vi "CRYPost Processing Editor.vi"() -> ()   [LabVIEW 2013]
uses:
  <vilib>/Utility/miscctls.llb/LVBoundsTypeDef.ctl
  Typedef Control/CRYPost Processing Cluster.ctl
  Typedef Control/CRYUser Equation Cluster.ctl
  CRYProject/CRYProject Editor Global.vi
  SubVI/CRYPost Processing Global.vi
  Program/CRYRef nums global.vi
  CRYWindow/SubVI/CRYMain Sub Window Global.vi
  CRYMainGlobal.vi
  CRYStepSetup/CRYStepSetup Global.vi
panel:
  out "Result Data":string[](array[string])
  in  "A log/lin":u16
  in  "tmp Val_B":dbl min=1.0 format="%#_6p"
  in  "tmp Val_A":dbl min=1.0 format="%#_6p"
  out "Show Calcu":bool
  out "Post Processing Bk":T1 {"user equation cluster"."Results axis" items=["x", "y", "z"]; "user equation cluster"."Input axis" items=["x", "y", "z"]; "user equation cluster"."Custom unit results array"."dB ref" format="%.2f"; "user equation cluster"."Custom unit input array"."dB ref" format="%.2f"; "Constant" format="%#.5p"; "Unary Operator" format="%10.0f"; "Custom unit info"."dB ref" format="%.2f"; "Sampling Rate" format="%#.2p"}
  in  "SW_EdtObj":u8
  in  "CurLibChange":bool caption="Add Lib"
  out "Old Exponent":sgl
  out "Loading_F":bool
  in  "Add Lib":bool
  in  "AddStep":bool
  in  "StateOut":bool
  in  "Board Tab":enum32{"Page 1"}(tab)
  in  "Cancel":bool caption="Apply"
  in  "OK":bool caption="Apply"
  in  "Main Tab":enum32{"Setting", "Help"}(tab)
  in  "Smoothing_Res":bool caption="平滑"
  in  "Freq Sampling Rate":dbl caption="频率" format="%#.2p"
  in  "Freq Sampling Mode":u16(slide) caption="Ref Freq Mode"
  out "Freq Sampling":bool caption="频率"
  in  "Operation1 Tab":enum32{"Page 1"}(tab)
  in  "binary operation":u16(ring) items=[" +", " --", " x", "÷"]
  out "Operation_1":bool caption="运算"
  in  "Work in":u16(slide) caption="运算模式"
  in  "Result_axis Tab":enum32{"Page 1"}(tab)
  out "Resut x_axis":bool caption="结果X轴"
  in  "Axis Mode":u16(slide)
  in  "Desired Tab":enum32{"Page 1"}(tab)
  out "Desired Result":bool caption="结果"
  in  "Use default":bool caption="使用默认值"
  in  "Name":string caption="名称"
  in  "x_1":bool caption="x"
  in  "y_1":bool caption="y"
  in  "z_1":bool caption="z"
  out "Unit String":string caption="单位"
  in  "Unit_Cont":bool
  out "Show data":string
  in  "OpA2 Tab":enum32{"Page 1"}(tab)
  in  "Op_A2":u16(ring) items=["Stimulus", "时间包络 [Direct Out 1]", "Record Wave [Direct In 1]", "2-时间包络 [Direct Out 1]", "调用文件曲线1", "Stimulus - P", "2-Stimulus - P", "3-Stimulus - P"]
  out "Operand_A2":bool caption="操作数 A"
  in  "Sear_range Tab":enum32{"Page 1"}(tab)
  in  "Edit Range":bool
  in  "All":bool caption="所有"
  in  "Search List":i32(listbox) caption="Hz"
  out "Search Range":bool caption="搜索范围"
  in  "Width Tab":enum32{"Page 1"}(tab)
  in  "Octav Mode":u16(ring) items=["1/1 Octave", "1/3 Octave", "1/6 Octave", "1/12 Octave", "1/24 Octave", "User Defined log", "User Defined lin"]
  out "Width":bool caption="宽度"
  out "Weighting":bool caption="加权"
  in  "Weight Mode":u16(ring) items=["None", "Hanning"]
  in  "Hz_Oct_1":dbl=1.0 caption="1/n 倍频程" min=1.0 step=1.0 format="%#.2p"
  in  "Sear_type Tab":enum32{"Page 1"}(tab)
  in  "Search Mode":u16(slide)
  out "Search Type":bool caption="搜索类型"
  in  "Equation Tab":enum32{"Page 1"}(tab)
  in  "Clear All Fields":bool
  out "#Desired Results":u32 caption="结果个数"
  out "#Operands":u32 caption="操作数个数"
  in  "z_2":bool caption="z"
  in  "y_2":bool caption="y"
  in  "x_2":bool caption="x"
  out "Equation":bool caption="公式 (e.g. x=a0+a1;)"
  in  "Equ_List":string
  out "Show xy":string
  in  "Org_res Tab":enum32{"Page 1"}(tab)
  out "Original Res":string
  out "Steps":i32 caption="步骤"
  out "Org_Res":bool caption="原始分辨率"
  in  "New Resolution":u16(ring) items=["1/1 Octave", "1/3 Octave", "1/6 Octave", "1/12 Octave", "1/24 Octave"]
  out "New_Res":bool caption="新的分辨率"
  in  "Frequencies":u16(slide) caption="频率"
  in  "Hz_Oct_2":u32=1 caption="1/n 倍频程" min=1 step=1
  in  "Direct Tab":enum32{"Page 1"}(tab)
  in  "Total Rotation":i32 caption="总旋转"
  in  "Inc(deg.)":i32 caption="增量(deg.)"
  in  "Ref_Curve":u16(ring) items=["unity cal-in corr-in", "CRY33x Mic 1 corr-in", "CRY33x Mic 2 corr-in", "CRY33x Mic 3 corr-in", "CRY33x Mic 4 corr-in", "USB In L corr-in", "USB In R corr-in", "unity cal-out corr-out", "unity cal-out eq-out", "CRY602 Mouth 1 corr-out", "CRY602 Mouth 1 eq-out", "CRY602 Mouth 2 corr-out", "CRY602 Mouth 2 eq-out", "USB Out R corr-out", "USB Out R eq-out", "频率响应 [Direct Out 1]", "谐波 2 [Direct Out 1]", "谐波 3 [Direct Out 1]", "谐波 4 [Direct Out 1]", "谐波 5 [Direct Out 1]", "总谐波失真 [Direct Out 1]", "上下限 上限", "上下限 下限", "2-频率响应 [Direct Out 1]", "2-谐波 2 [Direct Out 1]", "2-谐波 3 [Direct Out 1]", "2-谐波 4 [Direct Out 1]", "2-谐波 5 [Direct Out 1]", "2-总谐波失真 [Direct Out 1]", "调用文件曲线1"]
  in  "Auto Inc":bool caption="自动增量"
  in  "Curve List":i32[](listbox) caption="Hz"
  in  "Direct_weight":bool caption="加权"
  in  "Weight Curve_2":u16(ring) items=["unity cal-in corr-in", "CRY33x Mic 1 corr-in", "CRY33x Mic 2 corr-in", "CRY33x Mic 3 corr-in", "CRY33x Mic 4 corr-in", "USB In L corr-in", "USB In R corr-in", "unity cal-out corr-out", "unity cal-out eq-out", "CRY602 Mouth 1 corr-out", "CRY602 Mouth 1 eq-out", "CRY602 Mouth 2 corr-out", "CRY602 Mouth 2 eq-out", "USB Out R corr-out", "USB Out R eq-out", "频率响应 [Direct Out 1]", "谐波 2 [Direct Out 1]", "谐波 3 [Direct Out 1]", "谐波 4 [Direct Out 1]", "谐波 5 [Direct Out 1]", "总谐波失真 [Direct Out 1]", "上下限 上限", "上下限 下限", "2-频率响应 [Direct Out 1]", "2-谐波 2 [Direct Out 1]", "2-谐波 3 [Direct Out 1]", "2-谐波 4 [Direct Out 1]", "2-谐波 5 [Direct Out 1]", "2-总谐波失真 [Direct Out 1]", "调用文件曲线1"]
  out "Reference Curve":bool caption="参考曲线"
  out "Curve Group":bool caption="曲线组"
  out "Weight Function":bool caption="加权函数"
  out "Increment":bool caption="增量"
  in  "Org_samp Tab":enum32{"Page 1"}(tab)
  in  "New  Samp Val":dbl min=1.0 format="%#_6p"
  out "Origi Samp Val":dbl caption="Original Sampling Rate" format="%#.2p"
  out "Origi SampRate":bool caption="原始采样率"
  out "New Samp Rate":bool caption="新采样率"
  in  "Freq Tab":enum32{"Page 1"}(tab)
  in  "Ref Frequency":dbl caption="参考频率" format="%#.2p"
  in  "Ref Wave":u16(ring) caption="参考波形" items=["Stimulus", "时间包络 [Direct Out 1]", "Record Wave [Direct In 1]", "2-时间包络 [Direct Out 1]", "调用文件曲线1", "Stimulus - P", "2-Stimulus - P", "3-Stimulus - P"]
  in  "Ref Freq Mode":u16(slide)
  out "Ref Freq":bool caption="参考频率"
  in  "Smooth Tab":enum32{"Page 1"}(tab)
  in  "Smoo Width":i32 min=1
  out "Smoothing":bool caption="平滑宽度(Hz)"
  in  "Window Tab":enum32{"Page 1"}(tab)
  out "Window":bool caption="窗口"
  in  "Win Mode":u16(ring) items=["None", "Cosine Taper", "Exponential"]
  in  "Sampling Tab":enum32{"Page 1"}(tab)
  in  "Samp Rate":dbl format="%#.2p"
  out "Sampling":bool caption="采样率"
  in  "Operation2 Tab":enum32{"Page 1"}(tab)
  out "Operation_2":bool caption="运算"
  in  "Statistical Operator":u16(ring) items=["平均值", "功率总和", "最大值", "最小值", "谐振估算", "反谐振估算", "IEEE TOLR", "IEEE ROLR", "IEEE SOLR", "ITU-T SLR", "ITU-T RLR", "ITU-T RLR w/ Leak", "ITU-T STMR", "Attack Time", "Release Time", "Zwicker Loudness"]
  in  "Unary Operator":u16(ring) items=["相反数", "倒数", "绝对值", "平方", "平方根", "指数", "自然对数", "Unwrap Phase", "Group Delay", "FFT", "Inverse FFT"]
  in  "Param Tab":enum32{"Page 1"}(tab)
  out "Parameter":bool caption="参数"
  in  "dB":sgl format="%#.4p"
  in  "%":sgl format="%#.4p"
  in  "Weight_fun Tab":enum32{"Page 1"}(tab)
  in  "Exponent":sgl caption="指数" format="%#.2p"
  out "Weighting_Func":bool caption="加权函数"
  in  "Use Default Exp":bool caption="用户默认值"
  in  "Weight Curve_1":u16(ring) caption="加权曲线" items=["unity cal-in corr-in", "CRY33x Mic 1 corr-in", "CRY33x Mic 2 corr-in", "CRY33x Mic 3 corr-in", "CRY33x Mic 4 corr-in", "USB In L corr-in", "USB In R corr-in", "unity cal-out corr-out", "unity cal-out eq-out", "CRY602 Mouth 1 corr-out", "CRY602 Mouth 1 eq-out", "CRY602 Mouth 2 corr-out", "CRY602 Mouth 2 eq-out", "USB Out R corr-out", "USB Out R eq-out", "频率响应 [Direct Out 1]", "谐波 2 [Direct Out 1]", "谐波 3 [Direct Out 1]", "谐波 4 [Direct Out 1]", "谐波 5 [Direct Out 1]", "总谐波失真 [Direct Out 1]", "上下限 上限", "上下限 下限", "2-频率响应 [Direct Out 1]", "2-谐波 2 [Direct Out 1]", "2-谐波 3 [Direct Out 1]", "2-谐波 4 [Direct Out 1]", "2-谐波 5 [Direct Out 1]", "2-总谐波失真 [Direct Out 1]", "调用文件曲线1"]
  in  "Type":u16(ring) caption="类型" items=["算数运算", "常数", "一元运算", "标量（统计）", "平滑", "交叉区间(搜索)", "自定义公式", "截取", "分辨率", "指向性", "倍频程转换", "重采样", "频率转换", "布尔"]
  in  "OpA1 Tab":enum32{"Page 1"}(tab)
  out "Operand_A1":bool caption="操作数 A"
  in  "Mode_A":u16(slide) scale=0.0..2.0
  out "unit_A":string
  out "Value_A":string caption="值"
  in  "Op_A1":u16(ring) items=["unity cal-in corr-in", "CRY33x Mic 1 corr-in", "CRY33x Mic 2 corr-in", "CRY33x Mic 3 corr-in", "CRY33x Mic 4 corr-in", "USB In L corr-in", "USB In R corr-in", "unity cal-out corr-out", "unity cal-out eq-out", "CRY602 Mouth 1 corr-out", "CRY602 Mouth 1 eq-out", "CRY602 Mouth 2 corr-out", "CRY602 Mouth 2 eq-out", "USB Out R corr-out", "USB Out R eq-out", "unity cal-in corr-in/User Defined", "unity cal-in sens-in", "CRY33x Mic 1 sens-in", "CRY33x Mic 2 sens-in", "CRY33x Mic 3 sens-in", "CRY33x Mic 4 sens-in", "USB In L sens-in", "USB In R sens-in", "unity cal-out sens-out", "CRY602 Mouth 1 sens-out", "CRY602 Mouth 2 sens-out", "USB Out R sens-out"]
  in  "OpB Tab":enum32{"Page 1"}(tab)
  out "Operand_B":bool caption="操作数 B (单值)"
  in  "Mode_B":u16(slide) scale=0.0..2.0
  out "Value_B":string caption="操作值"
  in  "Op_B":u16(ring) items=["User Defined", "unity cal-in sens-in", "CRY33x Mic 1 sens-in", "CRY33x Mic 2 sens-in", "CRY33x Mic 3 sens-in", "CRY33x Mic 4 sens-in", "USB In L sens-in", "USB In R sens-in", "unity cal-out sens-out", "CRY602 Mouth 1 sens-out", "CRY602 Mouth 2 sens-out", "USB Out R sens-out"]
  in  "Constant":dbl caption="常数" format="%#.5p"
  out "unit_B":string
  in  "Zwicker_func Tab":enum32{"Page 1"}(tab)
  out "Zwicker_Func":bool caption="Zwicker"
  in  "Loudness Spectrum":bool caption="光谱"
  in  "X_axis unit":u16(ring) caption="X轴单位" items=["Hz", "Bark"]
  in  "Work in Statics":u16(slide) caption="运算模式"
  in  "Boolean_type Tab":enum32{"Page 1"}(tab)
  out "Boolean Type":bool caption="结果"
  in  "Result Listbox":i32[](listbox)
  in  "Help":string
  in  "Apply":bool
  in  "Save As...":bool caption="Apply"
  in  "Revert":bool caption="Apply"
  in  "Load...":bool caption="Apply"
  out "User Equation String":string
  out "EndFlag":bool
  out "Ref Waveform":string
  out "Width name":string
  out "New_res str":string
  out "B_cur name":string
  out "A_cur name":string
  out "B_xyz array":u16[](array[numeric])
  out "A_xyz array":u16[](array[numeric])
  out "Hz_oct array":dbl[](array[numeric])
  out "Weight_Cur array":string[](array[string])
  out "Search Items":string[](array[string])
  in  "Check_s":bool[](array[boolean])
  in  "Check_Hz":bool[](array[boolean])
  out "All array":bool[](array[boolean])
  out "Work array":u16[](array[numeric])
  out "Show xyz":cluster{"x":bool, "y":bool, "z":bool}[](array[cluster])
  out "Ope_array":u16[](array[ring]) items=["+", "--", "x", "÷"]
  out "Custom unit info":T3 {"dB ref" format="%.2f"}
  out "Post Processing":T1 {"user equation cluster"."Results axis" items=["x", "y", "z"]; "user equation cluster"."Input axis" items=["x", "y", "z"]; "user equation cluster"."Custom unit results array"."dB ref" format="%.2f"; "user equation cluster"."Custom unit input array"."dB ref" format="%.2f"; "Constant" format="%#.5p"; "Unary Operator" format="%10.0f"; "Custom unit info"."dB ref" format="%.2f"; "Sampling Rate" format="%#.2p"}
  in  "stop":bool
  in  "Load Test":bool
  out "Proper VI No":i32
  out "VIMiniumBound":T4
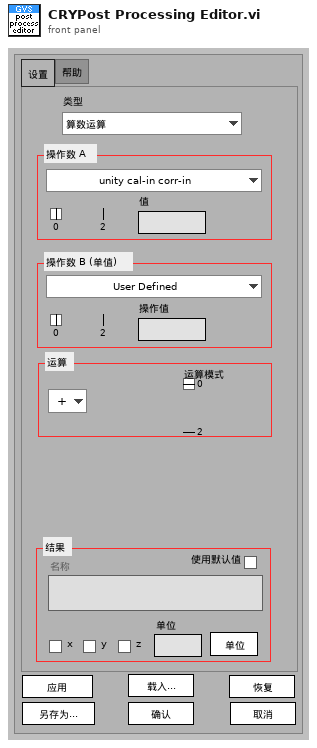
[diagram p1: front panel]
types:
  T1 = typedef "CRYPost Processing Cluster.ctl" = cluster{"Name":string, "Op Type":u16, "Curve A":string, "Curve B":string, "Axis Mode":u16, "Work Mode":u16, "Width":u16, "Weighting win":u16, "Search Mode":u16, "Freq Mode":u16, "New Sampling Rate":dbl, "Use Default Name":bool, "x":bool, "y":bool, "z":bool, "All points":bool, "A_single val axis":u16, "B_single val axis":u16, "Use Default Value":bool, "Result Name":string, "Smoothing Width":i32, "Window":u16, "Para_dB":sgl, "Para_%":sgl, "Exponent":sgl, "Hz":dbl, "Direct Weighting":bool, "Auto Inc":bool, "Inc(deg)":i32, "Total Rotation":i32, "Ref Freq Mode":u16, "Ref Waveform":string, "Sampling Rate":dbl, "Weighting Curve":string, "Ref Freq":dbl, "Curve Group":string[], "Search Items":string[], "Custom unit info":cluster{"use custom":bool, "lin/log":u16, "unit":string, "dB ref":dbl, "common dB":u16}, "Unit":string, "Type A":enum16{"Curves", "Values", "Results", "WFM"}, "Type B":enum16{"Curves", "Values", "Results", "WFM"}, "Unary Operator":u16, "Binary Operator":u16, "Statistical Operator":u16, "Constant ":dbl, "New Resolution":u16, "user equation cluster":T2, "Help":string, "Tab Value":enum32{"Setting", "Help"}, "Zwciker_X-axis":u16, "Zwicker_spectrum":bool, "Freq Sampling Mode":u16, "Freq Sampling Rate":dbl, "Smoothing":bool, "Work in Statics":u16, "Result Data":string[]}
  T2 = typedef "CRYUser Equation Cluster.ctl" = cluster{"Custom unit input array":cluster{"use custom":bool, "lin/log":u16, "unit":string, "dB ref":dbl, "common dB":u16}[], "Custom unit results array ":cluster{"use custom":bool, "lin/log":u16, "unit":string, "dB ref":dbl, "common dB":u16}[], "Desired Result Variables":string[], "Desired Result Names":string[], "Input Curve Names":string[], "Input Curve Variables":string[], "equation":string, "Input axis":u16[], "Results axis":u16[], "# input curves":i32, "# Desired result curves ":i32, "Input Values":string[], "Result Values":string[]}
  T3 = cluster{"use custom":bool, "lin/log":u16, "unit":string, "dB ref":dbl, "common dB":u16}
  T4 = typedef "LVBoundsTypeDef.ctl" = cluster{"Width":u32, "Height":u32}
  T5 = typedef "CRYStep.ctl" = cluster{"No.VI":i32, "Category":string, "StepName":string, "Seq setup flattened":string, "Comment":string, "Steps config.":bool[], "Jump config":i32[], "Start":dbl, "Increment":dbl, "Name":string, "Unit":string, "Y data":u16, "Y prefix":string, "Y dB ref":dbl, "Y unit":string, "Repeat State Array":cluster{"Start":dbl, "Increment":dbl, "Count":i32, "Num":i32}[]}
  T6 = typedef "CRYData Cluster Array.ctl" = T7[]
  T7 = typedef "CRYData Cluster.ctl" = cluster{"Name":string, "Curve":cluster{"x":dbl, "y":dbl, "z":dbl}[], "X data":u16, "Y data":u16, "Z data":u16, "X axis":u16, "Y axis":u16, "Z axis":u16, "X unit":string, "Y unit":string, "Z unit":string, "X dB ref":dbl, "Y dB ref":dbl, "Z dB ref":dbl, "single val":bool, "protected":bool, "display X":bool, "display Y":bool, "display Z":bool, "Test Info":string, "Step No.":i32, "Plot Settings":cluster{"Color":u32, "Interpolation":u8, "Point Style":u8, "Line Style":u8, "Point Color":u32, "Line Width":u8, "Bar Plot Style":u8, "Fill To":i16}, "AutoProtect":bool}
  T8 = enum16{"OK", "Yes", "YesNo", "YesNoCancel", "ReplaceAppend"}
  T9 = enum32{"English", "Chinese", "Korean", "Japanese", "Russian", "Chinese traditional"}
  T10 = enum32{"Invalid", "Standard", "Closed", "Hidden", "Minimized", "Maximized"}
  T11 = enum8{"Enabled", "Disabled", "Disabled and Grayed Out"}
  T12 = typedef "CRYResult Cluster Array.ctl" = T13[]
  T13 = typedef "CRYResult Cluster.ctl" = cluster{"Name":string, "Margin":dbl, "unit":string, "Verdict":bool, "Limit":string, "Max/Min":string, "protected":bool, "Step No.":i32, "Test Info":string, "AutoProtect":bool}
  T14 = typedef "CRYWaveform Cluster Array.ctl" = T15[]
  T15 = typedef "CRYWaveform Cluster.ctl" = cluster{"Waveform":cluster{"X0":dbl, "dX":dbl, "Y":sgl[]}, "X data":u16, "Y data":u16, "Y axis":u16, "X unit":string, "Y unit":string, "Y dB ref":dbl, "display Y":bool, "display X":bool, "Overload?":bool, "Test Info":string, "Step No.":i32, "Name":string, "protected":bool, "Sqc history":string[], "Signal Channel ID":i32, "Plot Settings":cluster{"Color":u32, "Interpolation":u8, "Point Style":u8, "Line Style":u8, "Point Color":u32, "Line Width":u8, "Bar Plot Style":u8, "Fill To":i16}, "AutoProtect":bool}
  T16 = cluster{"use custom":bool, "lin/log":u16, "unit":string, "dB ref":dbl, "common dB":u16}[]
  T17 = cluster{"Load Test":bool, "Apply":bool, "Unit_Cont":bool, "Edit Range":bool, "Clear All Fields":bool, "Add Lib":bool, "OK":bool, "Cancel":bool}
  T18 = cluster{"Res Name":string, "Type out":enum16{"Curves", "Values", "Results", "WFM"}}[]
  T19 = cluster{"Res Name":string, "Type out":enum16{"Curves", "Values", "Results", "WFM"}}
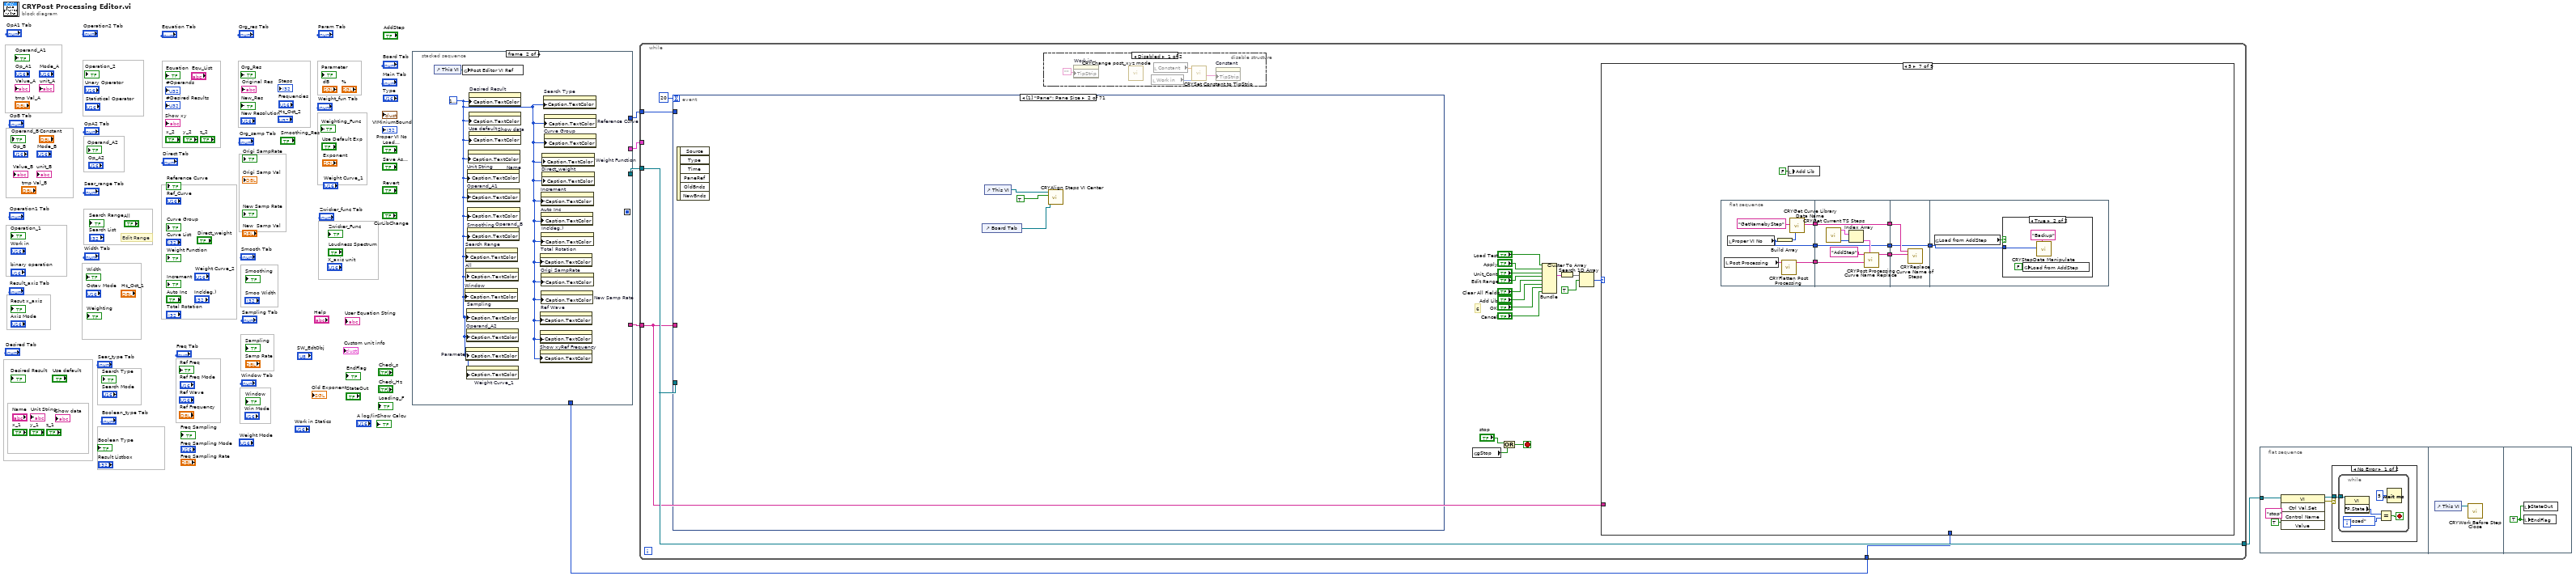
[diagram p0: block diagram]
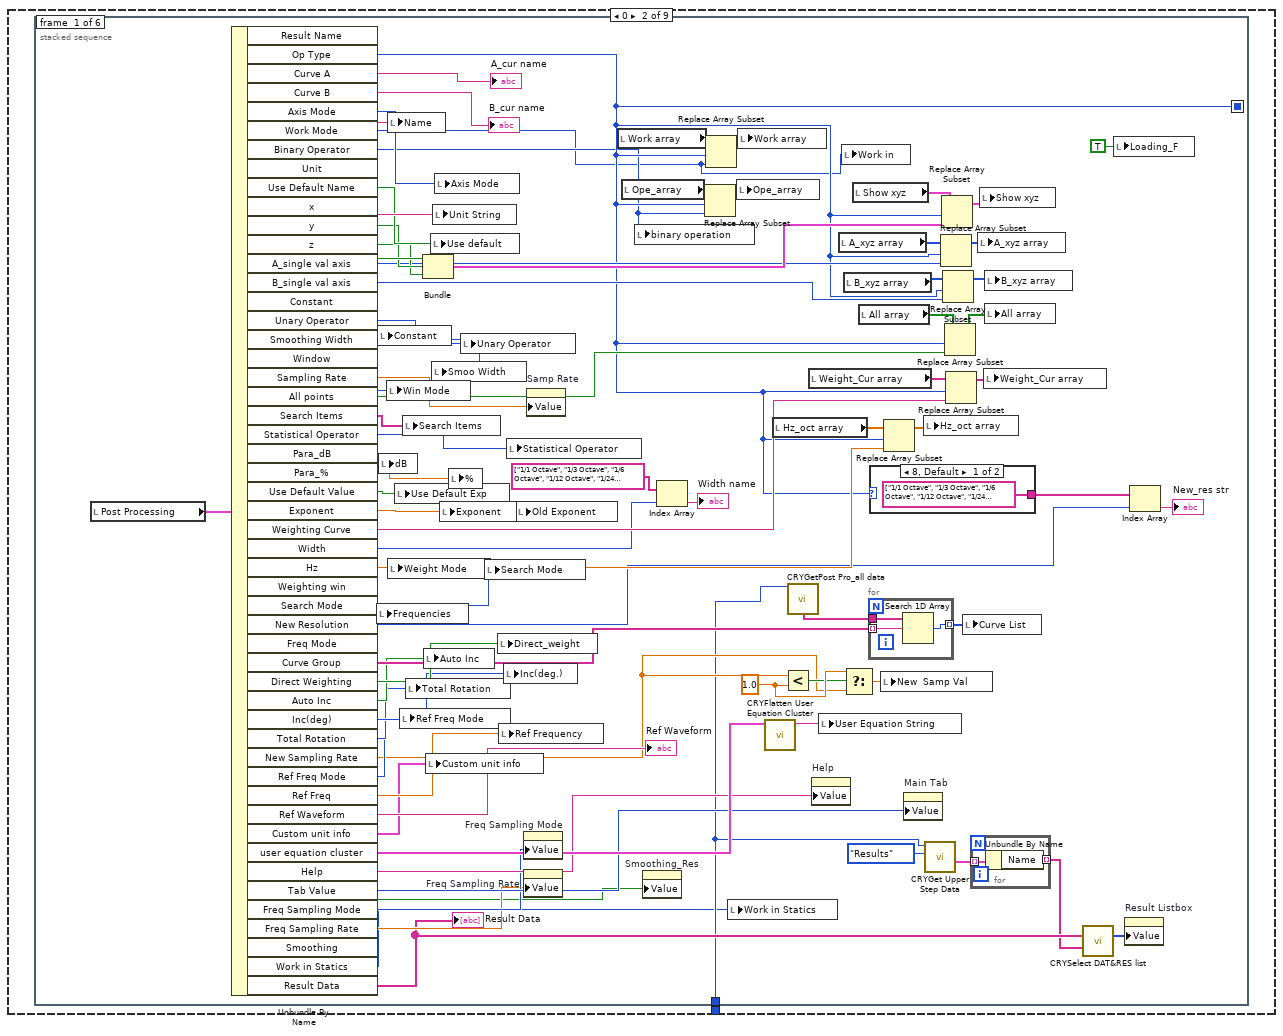
[diagram p5: hidden frame]
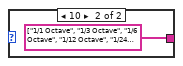
[diagram p6: hidden frame]
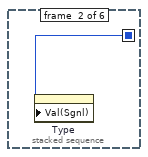
[diagram p7: hidden frame]
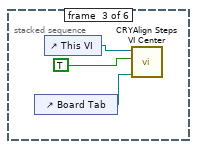
[diagram p8: hidden frame]
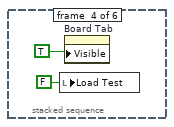
[diagram p9: hidden frame]
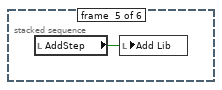
[diagram p10: hidden frame]
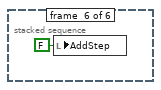
[diagram p11: hidden frame]
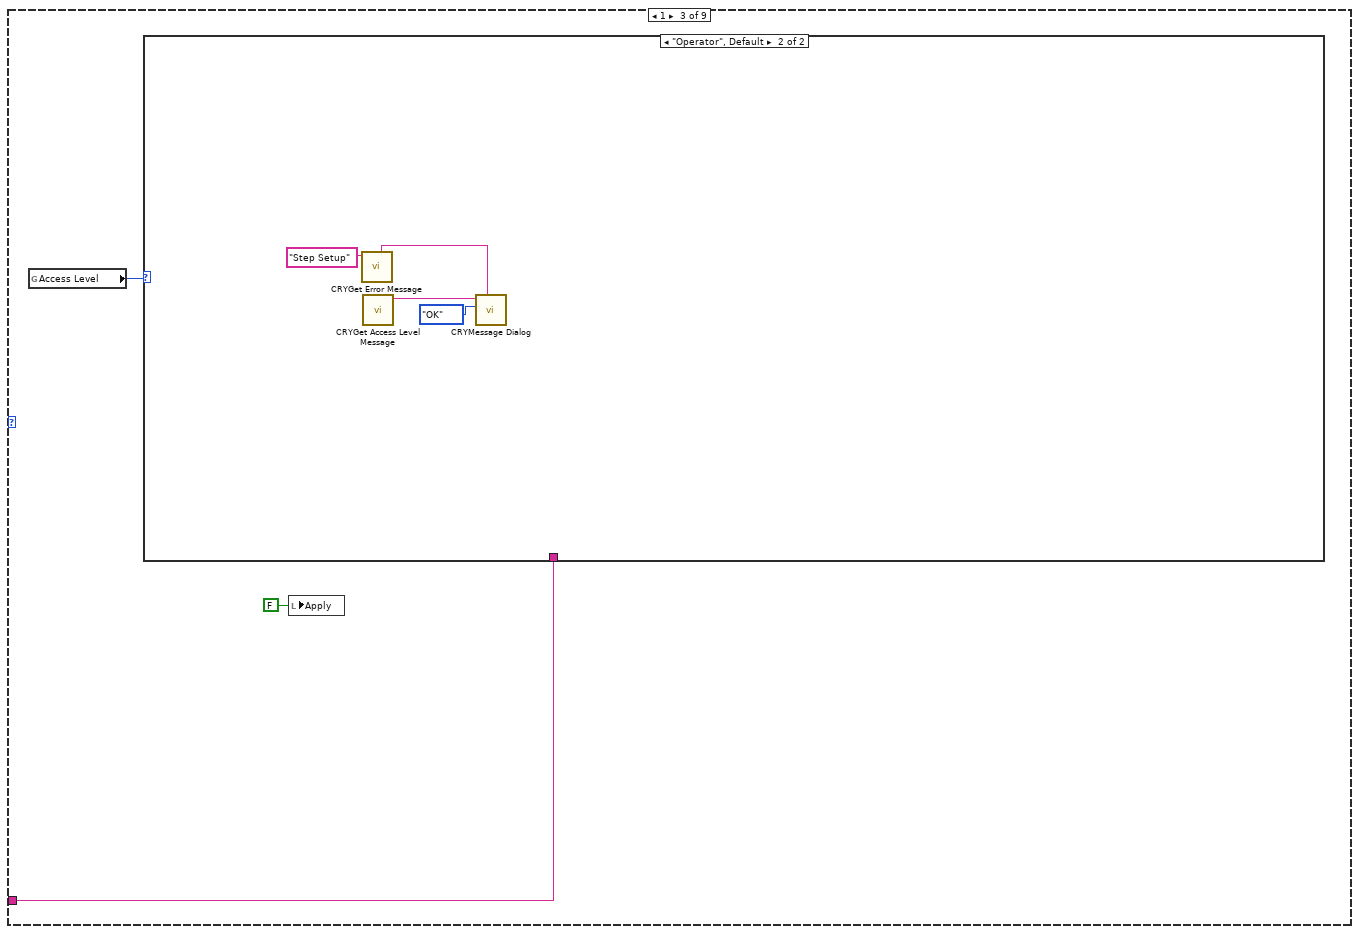
[diagram p12: hidden frame]
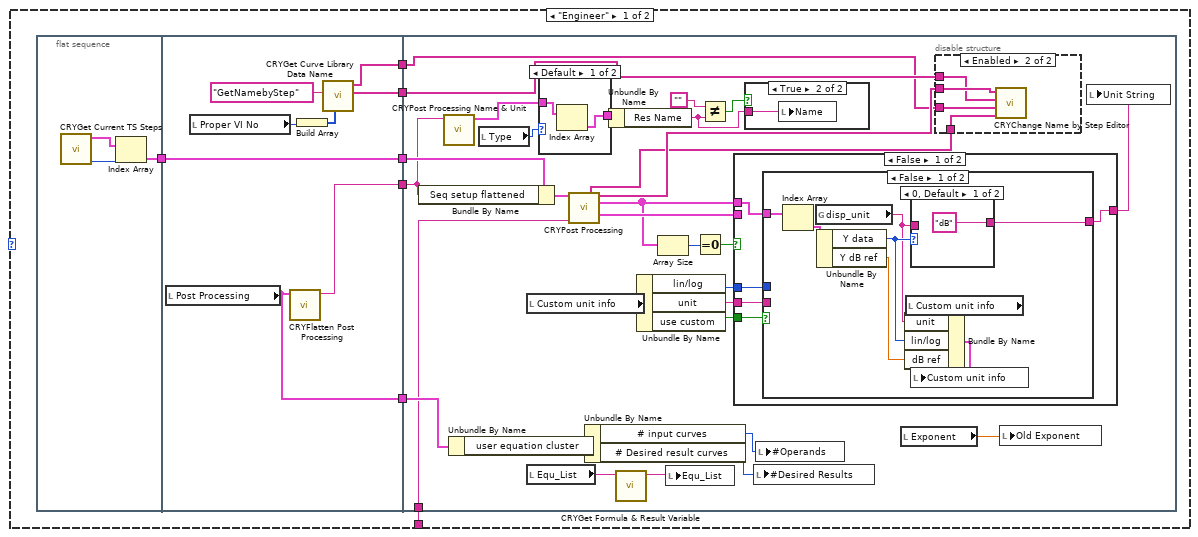
[diagram p13: hidden frame]
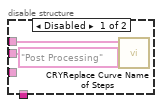
[diagram p14: hidden frame]
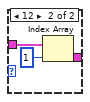
[diagram p16: hidden frame]
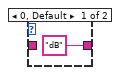
[diagram p19: hidden frame]
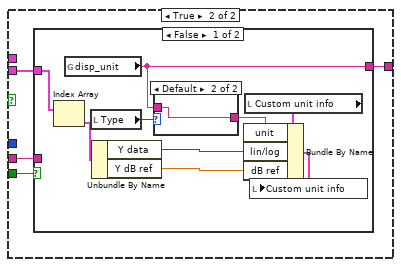
[diagram p20: hidden frame]
diagram:
  # "Edit Range"
  n1 = stacked-sequence {
    seq-local: [w12 _ _ _] -> [_ _ w23 _]
    tunnel: [w10 _ _ _] -> w6
    tunnel: [_ _ _ w45] -> w5
    tunnel: [w12 _ _ _] -> w3
    tunnel: [w12 _ _ _] -> w2
    tunnel: [w11 _ _ _] -> w1
    frame #0 {
      w8 = 0.0 ("tmp Val_A")
      w13 = FALSE ("Visible")
      n2 = call "CRYGet Current TS Steps.vi"() -> ("SelectStepNumber in Tree"=w16:i32, "Steps"=w17:T5[])  [unwired: 7 in, 3 out]
      n3 = Index Array(array=w17, index=w16) -> (element=w19:T5)
      n4 = property on="Board Tab" class="TabCtl (strict)"() -> ("Bounds"=w15:T4)  [unwired: 2 in, 2 out]
      n5 = local write "tmp Val_A"(w8) -> ()
      n6 = local write "tmp Val_B"(w8) -> ()
      n7 = Unbundle By Name(w19) -> ("Seq setup flattened"=w20:string, "StepName"=w11:string, "No.VI"=w12:i32)
      n8 = local write "A log/lin"(u16 0 ("A log/lin")) -> ()
      n9 = global read "CRYProject Editor Global.vi" "Step Setup VI No"() -> (w18:i32)
      n10 = property on="Revert" class="Bool (strict)"("Value"=FALSE ("ApplyTempFin")) -> ()  [unwired: 2 in, 2 out]
      n11 = local write "Load Test"(TRUE ("Load Test")) -> ()
      n12 = local write "stop"(w13) -> ()
      n13 = property on="Board Tab" class="TabCtl (strict)"("Visible"=w13) -> ()  [unwired: 2 in, 2 out]
      n14 = local write "VIMiniumBound"(w15) -> ()
      n15 = local write "Proper VI No"(w18) -> ()
      n16 = call "CRYUnflatten Post Processing.vi"("Unflatten Post Processing"=w20) -> ("Post-Processing"=w10:T1)  [unwired: 10 out]
      "Post Processing" <- w10
      "Post Processing Bk" <- w10
    }
    frame #1 {
      w21 = u32 16777222
      n17 = control-ref of="This VI"() -> (w22:refnum<vi>)
      n18 = global write "CRYPost Processing Global.vi" "Post Editor VI Ref"(w22) -> ()
      n19 = property on="Window" class="Bool (strict)"("Caption.TextColor"=w21) -> ()  [unwired: 2 in, 2 out]
      n20 = property on="Search Range" class="Bool (strict)"("Caption.TextColor"=w21) -> ()  [unwired: 2 in, 2 out]
      n21 = property on="All" class="Bool (strict)"("Caption.TextColor"=w21) -> ()  [unwired: 2 in, 2 out]
      n22 = property on="Parameter" class="Bool (strict)"("Caption.TextColor"=w21) -> ()  [unwired: 2 in, 2 out]
      n23 = property on="Sampling" class="Bool (strict)"("Caption.TextColor"=w21) -> ()  [unwired: 2 in, 2 out]
      n24 = property on="Operand_A2" class="Bool (strict)"("Caption.TextColor"=w21) -> ()  [unwired: 2 in, 2 out]
      n25 = property on="Weight Curve_1" class="Ring (strict)"("Caption.TextColor"=w21) -> ()  [unwired: 2 in, 2 out]
      n26 = property on="Unit String" class="Str"("Caption.TextColor"=w21) -> ()  [unwired: 2 in, 2 out]
      n27 = property on="Smoothing" class="Bool (strict)"("Caption.TextColor"=w21) -> ()  [unwired: 2 in, 2 out]
      n28 = property on="Operand_A1" class="Bool (strict)"("Caption.TextColor"=w21) -> ()  [unwired: 2 in, 2 out]
      n29 = property on="Operand_B" class="Bool (strict)"("Caption.TextColor"=w21) -> ()  [unwired: 2 in, 2 out]
      n30 = property on="Name" class="Str"("Caption.TextColor"=w21) -> ()  [unwired: 2 in, 2 out]
      n31 = property on="Desired Result" class="Bool (strict)"("Caption.TextColor"=w21) -> ()  [unwired: 2 in, 2 out]
      n32 = property on="Show data" class="Str"("Caption.TextColor"=w21) -> ()  [unwired: 2 in, 2 out]
      n33 = property on="Use default" class="Bool (strict)"("Caption.TextColor"=w21) -> ()  [unwired: 2 in, 2 out]
      n34 = property on="Show xy" class="Str"("Caption.TextColor"=w21) -> ()  [unwired: 2 in, 2 out]
      n35 = property on="Total Rotation" class="DigNum (strict)"("Caption.TextColor"=w21) -> ()  [unwired: 2 in, 2 out]
      n36 = property on="Ref Wave" class="Ring (strict)"("Caption.TextColor"=w21) -> ()  [unwired: 2 in, 2 out]
      n37 = property on="Ref Frequency" class="DigNum (strict)"("Caption.TextColor"=w21) -> ()  [unwired: 2 in, 2 out]
      n38 = property on="Auto Inc" class="Bool (strict)"("Caption.TextColor"=w21) -> ()  [unwired: 2 in, 2 out]
      n39 = property on="New Samp Rate" class="Bool (strict)"("Caption.TextColor"=w21) -> ()  [unwired: 2 in, 2 out]
      n40 = property on="Increment" class="Bool (strict)"("Caption.TextColor"=w21) -> ()  [unwired: 2 in, 2 out]
      n41 = property on="Inc(deg.)" class="DigNum (strict)"("Caption.TextColor"=w21) -> ()  [unwired: 2 in, 2 out]
      n42 = property on="Origi SampRate" class="Bool (strict)"("Caption.TextColor"=w21) -> ()  [unwired: 2 in, 2 out]
      n43 = property on="Weight Function" class="Bool (strict)"("Caption.TextColor"=w21) -> ()  [unwired: 2 in, 2 out]
      n44 = property on="Direct_weight" class="Bool (strict)"("Caption.TextColor"=w21) -> ()  [unwired: 2 in, 2 out]
      n45 = property on="Search Type" class="Bool (strict)"("Caption.TextColor"=w21) -> ()  [unwired: 2 in, 2 out]
      n46 = property on="Reference Curve" class="Bool (strict)"("Caption.TextColor"=w21) -> ()  [unwired: 2 in, 2 out]
      n47 = property on="Curve Group" class="Bool (strict)"("Caption.TextColor"=w21) -> ()  [unwired: 2 in, 2 out]
    }
    frame #2 {
      w26 = u16[] [0, 0] items=["+", "--", "x", "÷"] ("Ope_array")
      w27 = u16[] [1, 1, 1, 1, 1, 1] ("A_xyz array")
      n48 = property on="z_2" class="Bool (strict)"("Disabled"=u8 2, "Value"=FALSE ("z_2")) -> ()  [unwired: 2 in, 2 out]
      n49 = call "CRYGet Upper Step Data.vi"("Type In"=enum16{"Curves", "Values", "Results", "WFM"}."Curves", "No.VI"=w23) -> ("Curve array"=w33:T6)  [unwired: 9 out]
      n50 = Index Array(array=w33, index=0) -> (element=w38:T7)
      n51 = Unbundle By Name(w38) -> ("Name"=w36:string)
      n52 = for {
        N: 10 -> [_]
        tunnel: w36 -> [w40]
        tunnel: [w40] -> w35 mode=indexing
      }
      "Weight_Cur array" <- w35
      "Show xyz" <- cluster{"x":bool, "y":bool, "z":bool}[] [{"x"=FALSE, "y"=FALSE, "z"=FALSE}, {"x"=FALSE, "y"=FALSE, "z"=FALSE}, {"x"=FALSE, "y"=FALSE, "z"=FALSE}, {"x"=FALSE, "y"=FALSE, "z"=FALSE}, {"x"=FALSE, "y"=FALSE, "z"=FALSE}, {"x"=FALSE, "y"=FALSE, "z"=FALSE}, {"x"=FALSE, "y"=FALSE, "z"=FALSE}, {"x"=FALSE, "y"=FALSE, "z"=FALSE}, {"x"=FALSE, "y"=FALSE, "z"=FALSE}, {"x"=FALSE, "y"=FALSE, "z"=FALSE}, {"x"=FALSE, "y"=FALSE, "z"=FALSE}, {"x"=FALSE, "y"=FALSE, "z"=FALSE}, {"x"=FALSE, "y"=FALSE, "z"=FALSE}] ("Show data")
      "Work array" <- u16[] [0, 0] ("Work array")
      "Ope_array" <- w26
      "All array" <- bool[] [FALSE, FALSE, FALSE, FALSE, FALSE, FALSE, FALSE, FALSE] ("All array")
      "Search Items" <- string[] [] ("Search Items")
      "Hz_oct array" <- dbl[] [0.0, 0.0, 0.0, 0.0, 0.0, 0.0, 0.0, 0.0, 0.0] ("Hz_oct array")
      "A_xyz array" <- w27
      "B_xyz array" <- w27
    }
    frame #3 {
      n53 = global read "CRYRef nums global.vi" "Post Sub VI ref"() -> (w41:refnum<vi>)
      n54 = local write "EndFlag"(FALSE ("EndFlag")) -> ()
      n55 = invoke class="VI" method="Run VI"(reference=w41, "Wait until done"=FALSE ("Wait Until Done")) -> (reference out=w43:refnum<vi>)  [unwired: 3 in, 4 out]
      n56 = property class="VI"(reference=w43, "Front Panel.Open"=FALSE ("Front Panel Window:Open")) -> (reference out=w45:refnum<vi>)  [unwired: 1 in, 1 out]
    }
  }
  n57 = while {
    tunnel: w6 -> [_]
    tunnel: w5 -> [w56]
    tunnel: [w56] -> w4
    tunnel: w3 -> [w52]
    tunnel: w2 -> [w51]
    tunnel: w1 -> [w50]
    stop <- w55 stop-if-true
    # "6"
    n58 = event shown="[1] \"Pane\": Pane Size" {
      selector: _ -> [_ _ _ _ _ _ _ _ _ _ _ _ _ _ _ _ _ _ _ _ _ _ _ _ _ _ _ _ _ _ _ _ _ _ _ _ _ _ _ _ _ _ _ _ _ _ _ _ _ _ _ _ _ _ _ _ _ _ _ _ _ _ _ _ _ _ _ _ _ _ _]
      dyn-events: _ -> [_ _ _ _ _ _ _ _ _ _ _ _ _ _ _ _ _ _ _ _ _ _ _ _ _ _ _ _ _ _ _ _ _ _ _ _ _ _ _ _ _ _ _ _ _ _ _ _ _ _ _ _ _ _ _ _ _ _ _ _ _ _ _ _ _ _ _ _ _ _ _]
      timeout: 20 -> [_ _ _ _ _ _ _ _ _ _ _ _ _ _ _ _ _ _ _ _ _ _ _ _ _ _ _ _ _ _ _ _ _ _ _ _ _ _ _ _ _ _ _ _ _ _ _ _ _ _ _ _ _ _ _ _ _ _ _ _ _ _ _ _ _ _ _ _ _ _ _]
      tunnel: w56 -> [_ _ _ _ _ _ _ w467 _ _ _ _ _ _ _ _ _ _ _ _ _ _ _ _ _ _ _ _ _ _ _ _ _ _ _ _ _ _ _ _ _ _ _ _ _ _ _ _ _ _ _ _ _ _ _ _ _ _ _ _ w1977 _ _ _ _ _ _ _ _ _ _]
      tunnel: w51 -> [_ _ _ _ _ _ _ w445 w696 w912 w1041 w1193 _ _ _ _ w1392 w1421 _ _ _ _ _ _ _ _ _ _ _ _ _ _ _ w1672 _ w1722 _ _ _ _ _ _ _ w1840 w1848 _ w1864 _ _ _ _ _ w1901 _ _ _ _ _ _ _ _ w1993 _ _ _ _ _ _ _ _ _]
      tunnel: w50 -> [_ _ _ _ _ _ _ _ _ _ _ _ w1230 _ _ _ _ _ _ _ _ _ _ _ _ _ _ _ _ _ _ _ _ _ _ _ _ _ _ _ _ _ _ _ _ _ _ _ _ _ _ _ _ _ _ _ _ _ _ _ _ _ _ _ _ _ _ _ _ _ _]
      event Timeout {
        n59 = event-data() -> ()  [unwired: 3 out]
        n60 = local write "Loading_F"(FALSE ("Loading_F")) -> ()
      }
      event Pane Size {
        n61 = event-data() -> ()  [unwired: 7 out]
        n62 = control-ref of="Board Tab"() -> (w391:refnum<vi>)
        n63 = control-ref of="This VI"() -> (w393:refnum<vi>)
        n64 = call "CRYAlign Steps VI Center.vi"("Tab2"=w391, "Input/Output"=TRUE, "VIRef"=w393) -> ()  [unwired: 1 in, 8 out]
      }
      event "Load...": Value Change {
        n65 = event-data() -> ("CtlRef"=w394:refnum<vi>)  [unwired: 6 out]
        n66 = property class="Bool (strict)"(reference=w394, "Value"=FALSE) -> ()  [unwired: 1 in, 2 out]
        n67 = local read "Load Test"() -> (w396:bool)
        n68 = case shown="False" w396 {
          frame False {
            n69 = global read "CRYMainGlobal.vi" "Steps path"() -> (w402:path)
            n70 = local read "Proper VI No"() -> (w397:i32)
            n71 = Build Path(base path=w402, name or relative path="CRYPost Processing") -> (appended path=w401:path)
            n72 = call "CRYStep Read.vi"("Category Name"="Post Processing" ("Step File Name"), "Proper VI No"=w397, "Step File Path"=w401) -> ("status"=w400:bool, "selected path"=w398:path, "Flatten Step"=w399:string)  [unwired: 1 in, 3 out]
            n73 = case shown="True" w400 {
              tunnel: w399 -> [_ w406]
              tunnel: w398 -> [_ w405]
              tunnel: w397 -> [_ w407]
              frame False {
              }
              frame True {
                n74 = call "CRYUnflatten Post Processing.vi"("Unflatten Post Processing"=w406) -> ("Error?"=w409:bool, "Post-Processing"=w408:T1)  [unwired: 9 out]
                n75 = case shown="False" w409 {
                  tunnel: w408 -> [w413 _]
                  tunnel: w407 -> [w412 _]
                  tunnel: w406 -> [w411 _]
                  tunnel: w405 -> [w410 _]
                  frame False {
                    n76 = flat-sequence {
                      tunnel: w413 -> [w425]
                      tunnel: w412 -> [w422]
                      tunnel: w411 -> [w421]
                      tunnel: w410 -> [w420]
                      frame #0 {
                        n77 = Strip Path(path=w420) -> (name=w415:string)  [unwired: 1 out]
                        n78 = local write "Post Processing"(w425) -> ()
                        n79 = Reverse String(1:w415) -> (0:w417:string)
                        n80 = Match Pattern(string=w417, regular expression="[.]") -> (after substring=w418:string)  [unwired: 4 out]
                        n81 = Reverse String(1:w418) -> (0:w414:string)
                        n82 = call "CRYPreUpdate Sequence.vi"("EventName"="Load", "StepName Arg3"=w414, "Proper VI No"=w422, "Project View Step Name Identifier Arg1"="", "Step flattened Arg2"=w421, "AllChangeFlg"=TRUE ("Name/Identifier")) -> ()  [unwired: 10 in]
                      }
                      frame #1 {
                        n83 = local write "Load Test"(TRUE ("Load Test")) -> ()
                      }
                    }
                  }
                  frame True {
                  }
                }
              }
            }
          }
          frame True {
          }
        }
      }
      event "Save As...": Value Change {
        w429 = "Post Processing" ("Step File Name")
        n84 = event-data() -> ("CtlRef"=w427:refnum<vi>)  [unwired: 6 out]
        n85 = property class="Bool (strict)"(reference=w427, "Value"=FALSE) -> ()  [unwired: 1 in, 2 out]
        n86 = local read "Post Processing"() -> (w431:T1)
        n87 = global read "CRYMainGlobal.vi" "Steps path"() -> (w432:path)
        n88 = local read "Proper VI No"() -> (w430:i32)
        n89 = call "CRYFlatten Post Processing.vi"("Post-Processing"=w431) -> ("Post Processing flattened"=w437:string)  [unwired: 10 out]
        n90 = Build Path(base path=w432, name or relative path="CRYPost Processing") -> (appended path=w434:path)
        n91 = call "CRYStep Write.vi"("StepIdentifier"="", "Default"=FALSE, "Proper VI No"=w430, "Category Name"=w429, "Step File Path"=w434, "Step flattened"=w437, "Step File Name"=w429) -> ()  [unwired: 1 in, 4 out]
      }
      event "Revert": Value Change {
        n92 = event-data() -> ("CtlRef"=w439:refnum<vi>)  [unwired: 6 out]
        n93 = property class="Bool (strict)"(reference=w439, "Value"=FALSE) -> ()  [unwired: 1 in, 2 out]
        n94 = flat-sequence {
          frame #0 {
            n95 = local read "Post Processing Bk"() -> (w440:T1)
            n96 = local write "Post Processing"(w440) -> ()
          }
          frame #1 {
            n97 = local write "Load Test"(TRUE ("Load Test")) -> ()
          }
        }
      }
      event Panel Close {
        n98 = event-data() -> ()  [unwired: 5 out]
        n99 = local write "Cancel"(TRUE ("Cancel")) -> ()
        n100 = control-ref of="This VI"() -> (w443:refnum<vi>)
        n101 = call "CRYWork Before Step Close.vi"("StepVI Ref"=w443) -> ()  [unwired: 11 in]
      }
      event "CurLibChange": Value Change {
        n102 = event-data() -> ()  [unwired: 7 out]
        n103 = property on="Type" class="Ring (strict)"() -> ("Value"=w444:u16)  [unwired: 2 in, 2 out]
        n104 = property on="Type" class="Ring (strict)"("Val(Sgnl)"=w444) -> ()  [unwired: 2 in, 2 out]
      }
      event "Type": Value Change {
        n105 = event-data() -> ("OldVal"=w450:u16, "NewVal"=w449:u16)  [unwired: 5 out]
        n106 = local read "Post Processing"() -> (w458:T1)
        n107 = call "CRYGetPost Pro_all data.vi"("No.VI"=w445) -> ("All Names"=w465:string[], "C&W Names"=w463:string[], "Value Names"=w464:string[], "Curve Names"=w461:string[], "Wave names"=w462:string[])  [unwired: 1 in, 9 out]
        n108 = Bundle By Name(cluster=w458, "Op Type"=w449) -> (w459:T1)
        n109 = local write "Post Processing"(w459) -> ()
        n110 = call "CRYGet Error Message.vi"("Kind"="Post Processing Sub") -> ("Unicode Message Sub"=w457:string[])  [unwired: 5 in, 5 out]
        n111 = for {
          tunnel: w457 -> [w482] mode=indexing
          tunnel: [w481] -> w456 mode=indexing
          n112 = call "CRYConvert Unicode to ASCII.vi"("Unicode"=w482) -> ("ASCII"=w481:string)  [unwired: 4 in]
        }
        n113 = local read "Loading_F"() -> (w452:bool)
        n114 = Not Equal?(x=w450, y=w449) -> (x != y?=w453:bool)
        n115 = Not(x=w452) -> (.not. x?=w451:bool)
        n116 = And(x=w453, y=w451) -> (x .and. y?=w454:bool)
        n117 = case shown="True" w454 {
          frame True {
            n118 = local read "Custom unit info"() -> (w479:T3)
            n119 = Unbundle By Name(w479) -> ("use custom"=w478:bool)
            n120 = case shown="False" w478 {
              frame False {
                n121 = local write "Unit String"("") -> ()
              }
              frame True {
              }
            }
          }
          frame False {
          }
        }
        n122 = case shown="\"English\", Default" T9."English" ("Language") {
          tunnel: [string[] ["1\u0000/\u00001\u0000 \u0000O\u0000c\u0000t\u0000a\u0000v\u0000e\u0000", "1\u0000/\u00003\u0000 \u0000O\u0000c\u0000t\u0000a\u0000v\u0000e\u0000", "1\u0000/\u00006\u0000 \u0000O\u0000c\u0000t\u0000a\u0000v\u0000e\u0000", "1\u0000/\u00001\u00002\u0000 \u0000O\u0000c\u0000t\u0000a\u0000v\u0000e\u0000", "1\u0000/\u00002\u00004\u0000 \u0000O\u0000c\u0000t\u0000a\u0000v\u0000e\u0000", "U\u0000s\u0000e\u0000r\u0000 \u0000D\u0000e\u0000f\u0000i\u0000n\u0000e\u0000d\u0000 \u0000l\u0000o\u0000g\u0000", "U\u0000s\u0000e\u0000r\u0000 \u0000D\u0000e\u0000f\u0000i\u0000n\u0000e\u0000d\u0000 \u0000l\u0000i\u0000n\u0000"] string[] ["1\u0000/\u00001\u0000 \u0000\rP‘˜\u000bz", "1\u0000/\u00003\u0000 \u0000\rP‘˜\u000bz", "1\u0000/\u00006\u0000 \u0000\rP‘˜\u000bz", "1\u0000/\u00001\u00002\u0000 \u0000\rP‘˜\u000bz", "1\u0000/\u00002\u00004\u0000 \u0000\rP‘˜\u000bz", "ê[INù[pe", "ê[IN¿~'`"]] -> w448
          frame "English", Default {
          }
          frame "Chinese" {
          }
        }
        n123 = for {
          tunnel: w448 -> [w475] mode=indexing
          tunnel: [w474] -> w447 mode=indexing
          n124 = call "CRYConvert Unicode to ASCII.vi"("Unicode"=w475) -> ("ASCII"=w474:string)  [unwired: 4 in]
        }
        n125 = case shown="6" w449 {
          selector: w449 -> [w483 w508 w536 w547 w562 w571 w597 w607 w620 w642 w659 w667 w687]
          tunnel: w465 -> [w490 w510 w537 _ _ w572 _ _ _ _ _ _ _]
          tunnel: w464 -> [_ w509 _ _ _ _ _ _ _ _ _ _ _]
          tunnel: w463 -> [_ _ _ w548 w564 _ _ w608 _ _ _ _ _]
          tunnel: w462 -> [_ _ _ _ _ _ _ _ _ _ w660 w681 _]
          tunnel: w461 -> [_ _ _ _ _ _ _ _ w619 w656 _ _ _]
          tunnel: w456 -> [w501 w515 _ _ _ w580 _ _ _ _ _ _ _]
          tunnel: w447 -> [_ _ _ _ w561 _ _ _ w618 _ _ _ _]
          tunnel: w445 -> [_ _ _ _ _ _ _ _ _ _ _ _ w685]
          frame 0, Default {
            # "Arithmetic"
            n126 = property on="SW_EdtObj" class="DigNum (strict)"("Val(Sgnl)"=w483) -> ()  [unwired: 2 in, 2 out]
            n127 = local read "A_cur name"() -> (w507:string)
            n128 = local read "B_cur name"() -> (w496:string)
            n129 = property on="Op_B" class="Ring (strict)"("Strings []"=w490) -> ()  [unwired: 2 in, 2 out]
            n130 = property on="Op_A1" class="Ring (strict)"("Strings []"=w490) -> ()  [unwired: 2 in, 2 out]
            n131 = local read "Work array"() -> (w487:u16[])
            n132 = local read "Ope_array"() -> (w489:u16[])
            n133 = local read "Axis Mode"() -> (w485:u16)
            n134 = local read "Type"() -> (w484:u16)
            n135 = Search 1D Array(1D array=w490, element=w507) -> (index of element=w503:i32)  [unwired: 1 out]
            n136 = Search 1D Array(1D array=w490, element=w496) -> (index of element=w492:i32)  [unwired: 1 out]
            n137 = Equal?(x=-1 ("y"), y=w503) -> (x = y?=w506:bool)
            n138 = Equal?(x=-1 ("y"), y=w492) -> (x = y?=w493:bool)
            n139 = Index Array(array=w487, index=w484) -> (element=w486:u16)
            n140 = Index Array(array=w489, index=w484) -> (element=w488:u16)
            n141 = Select(t=0 ("y"), s=w506, f=w503) -> (s? t:f=w502:i32)
            n142 = Select(t=0 ("y"), s=w493, f=w492) -> (s? t:f=w491:i32)
            n143 = Index Array(array=w501, index #1=0 ("index"), index #2=5 ("index")) -> (element #1=w499:string, element #2=w497:string)
            n144 = property on="Op_A1" class="Ring (strict)"("Val(Sgnl)"=w502) -> ()  [unwired: 2 in, 2 out]
            n145 = property on="Op_B" class="Ring (strict)"("Val(Sgnl)"=w491) -> ()  [unwired: 2 in, 2 out]
            n146 = property on="binary operation" class="Ring (strict)"("Val(Sgnl)"=w488) -> ()  [unwired: 2 in, 2 out]
            n147 = property on="Work in" class="Slide (strict)"("Val(Sgnl)"=w486) -> ()  [unwired: 2 in, 2 out]
            n148 = property on="Axis Mode" class="Slide (strict)"("Val(Sgnl)"=w485) -> ()  [unwired: 2 in, 2 out]
            n149 = property on="Value_B" class="Str"("Caption.Text"=w499) -> ()  [unwired: 2 in, 2 out]
            n150 = property on="Operand_B" class="Bool (strict)"("Caption.Text"=w497) -> ()  [unwired: 2 in, 2 out]
          }
          frame 1 {
            # "Constant"
            n151 = flat-sequence {
              tunnel: w508 -> [w516]
              tunnel: w510 -> [w529]
              tunnel: w509 -> [w518]
              frame #0 {
                n152 = property on="SW_EdtObj" class="DigNum (strict)"("Val(Sgnl)"=w516) -> ()  [unwired: 2 in, 2 out]
              }
              frame #1 {
                n153 = local read "A_cur name"() -> (w535:string)
                n154 = local read "B_cur name"() -> (w528:string)
                n155 = local read "Work array"() -> (w519:u16[])
                n156 = local read "Ope_array"() -> (w522:u16[])
                n157 = Search 1D Array(1D array=w529, element=w535) -> (index of element=w531:i32)  [unwired: 1 out]
                n158 = local read "Type"() -> (w517:u16)
                n159 = Search 1D Array(1D array=w518, element=w528) -> (index of element=w524:i32)  [unwired: 1 out]
                n160 = Equal?(x=-1 ("y"), y=w531) -> (x = y?=w534:bool)
                n161 = Equal?(x=-1 ("y"), y=w524) -> (x = y?=w525:bool)
                n162 = Select(t=0 ("y"), s=w534, f=w531) -> (s? t:f=w530:i32)
                n163 = Index Array(array=w519, index=w517) -> (element=w520:u16)
                n164 = Index Array(array=w522, index=w517) -> (element=w521:u16)
                n165 = Select(t=0 ("y"), s=w525, f=w524) -> (s? t:f=w523:i32)
                n166 = property on="Op_A1" class="Ring (strict)"("Val(Sgnl)"=w530) -> ()  [unwired: 2 in, 2 out]
                n167 = property on="Op_B" class="Ring (strict)"("Val(Sgnl)"=w523) -> ()  [unwired: 2 in, 2 out]
                n168 = property on="binary operation" class="Ring (strict)"("Val(Sgnl)"=w521) -> ()  [unwired: 2 in, 2 out]
                n169 = property on="Work in" class="Slide (strict)"("Val(Sgnl)"=w520) -> ()  [unwired: 2 in, 2 out]
              }
            }
            n170 = property on="Op_A1" class="Ring (strict)"("Strings []"=w510) -> ()  [unwired: 2 in, 2 out]
            n171 = property on="Op_B" class="Ring (strict)"("Strings []"=w509) -> ()  [unwired: 2 in, 2 out]
            n172 = Index Array(array=w515, index #1=1 ("index"), index #2=6 ("index")) -> (element #1=w514:string, element #2=w511:string)
            n173 = property on="Value_B" class="Str"("Caption.Text"=w514) -> ()  [unwired: 2 in, 2 out]
            n174 = property on="Operand_B" class="Bool (strict)"("Caption.Text"=w511) -> ()  [unwired: 2 in, 2 out]
          }
          frame 2 {
            # "Unary"
            n175 = flat-sequence {
              tunnel: w536 -> [w538]
              tunnel: w537 -> [w539]
              frame #0 {
                n176 = property on="SW_EdtObj" class="DigNum (strict)"("Val(Sgnl)"=w538) -> ()  [unwired: 2 in, 2 out]
              }
              frame #1 {
                n177 = local read "A_cur name"() -> (w546:string)
                n178 = local read "Unary Operator"() -> (w540:u16)
                n179 = Search 1D Array(1D array=w539, element=w546) -> (index of element=w542:i32)  [unwired: 1 out]
                n180 = Equal?(x=-1 ("y"), y=w542) -> (x = y?=w545:bool)
                n181 = property on="Unary Operator" class="Ring (strict)"("Val(Sgnl)"=w540) -> ()  [unwired: 2 in, 2 out]
                n182 = Select(t=0 ("y"), s=w545, f=w542) -> (s? t:f=w541:i32)
                n183 = property on="Op_A1" class="Ring (strict)"("Val(Sgnl)"=w541) -> ()  [unwired: 2 in, 2 out]
              }
            }
            n184 = property on="Op_A1" class="Ring (strict)"("Strings []"=w537) -> ()  [unwired: 2 in, 2 out]
          }
          frame 3 {
            # "Scalar(Statistics)"
            n185 = flat-sequence {
              tunnel: w547 -> [w549]
              tunnel: w548 -> [w551]
              frame #0 {
                n186 = property on="SW_EdtObj" class="DigNum (strict)"("Val(Sgnl)"=w549) -> ()  [unwired: 2 in, 2 out]
              }
              frame #1 {
                n187 = local read "A_cur name"() -> (w560:string)
                n188 = local read "All array"() -> (w554:bool[])
                n189 = local read "Statistical Operator"() -> (w550:u16)
                n190 = local read "Type"() -> (w552:u16)
                n191 = Search 1D Array(1D array=w551, element=w560) -> (index of element=w556:i32)  [unwired: 1 out]
                n192 = Equal?(x=-1 ("y"), y=w556) -> (x = y?=w559:bool)
                n193 = Index Array(array=w554, index=w552) -> (element=w553:bool)
                n194 = property on="Statistical Operator" class="Ring (strict)"("Val(Sgnl)"=w550) -> ()  [unwired: 2 in, 2 out]
                n195 = Select(t=0 ("y"), s=w559, f=w556) -> (s? t:f=w555:i32)
                n196 = property on="All" class="Bool (strict)"("Val(Sgnl)"=w553) -> ()  [unwired: 2 in, 2 out]
                n197 = property on="Op_A2" class="Ring (strict)"("Val(Sgnl)"=w555) -> ()  [unwired: 2 in, 2 out]
              }
            }
            n198 = property on="Op_A2" class="Ring (strict)"("Strings []"=w548) -> ()  [unwired: 2 in, 2 out]
          }
          frame 4 {
            # "Smoothing"
            n199 = property on="SW_EdtObj" class="DigNum (strict)"("Val(Sgnl)"=w562) -> ()  [unwired: 2 in, 2 out]
            n200 = property on="Op_A2" class="Ring (strict)"("Strings []"=w564) -> ()  [unwired: 2 in, 2 out]
            n201 = local read "A_cur name"() -> (w570:string)
            n202 = local read "Weight Mode"() -> (w563:u16)
            n203 = Search 1D Array(1D array=w564, element=w570) -> (index of element=w566:i32)  [unwired: 1 out]
            n204 = property on="Weight Mode" class="Ring (strict)"("Value"=w563) -> ()  [unwired: 2 in, 2 out]
            n205 = Equal?(x=-1 ("y"), y=w566) -> (x = y?=w569:bool)
            n206 = Select(t=0 ("y"), s=w569, f=w566) -> (s? t:f=w565:i32)
            n207 = property on="Octav Mode" class="Ring (strict)"("Strings []"=w561) -> ()  [unwired: 2 in, 2 out]
            n208 = property on="Op_A2" class="Ring (strict)"("Val(Sgnl)"=w565) -> ()  [unwired: 2 in, 2 out]
          }
          frame 5 {
            # "Intersection(Search)"
            n209 = flat-sequence {
              tunnel: w571 -> [w581]
              tunnel: w572 -> [w582]
              frame #0 {
                n210 = property on="SW_EdtObj" class="DigNum (strict)"("Val(Sgnl)"=w581) -> ()  [unwired: 2 in, 2 out]
              }
              frame #1 {
                n211 = local read "A_cur name"() -> (w594:string)
                n212 = local read "B_cur name"() -> (w588:string)
                n213 = Search 1D Array(1D array=w582, element=w588) -> (index of element=w584:i32)  [unwired: 1 out]
                n214 = Search 1D Array(1D array=w582, element=w594) -> (index of element=w590:i32)  [unwired: 1 out]
                n215 = Equal?(x=-1 ("y"), y=w590) -> (x = y?=w593:bool)
                n216 = Equal?(x=-1 ("y"), y=w584) -> (x = y?=w585:bool)
                n217 = Select(t=0 ("y"), s=w593, f=w590) -> (s? t:f=w589:i32)
                n218 = Select(t=0 ("y"), s=w585, f=w584) -> (s? t:f=w583:i32)
                n219 = property on="Op_B" class="Ring (strict)"("Val(Sgnl)"=w583) -> ()  [unwired: 2 in, 2 out]
                n220 = property on="Op_A1" class="Ring (strict)"("Val(Sgnl)"=w589) -> ()  [unwired: 2 in, 2 out]
              }
            }
            n221 = property on="Op_A1" class="Ring (strict)"("Strings []"=w572) -> ()  [unwired: 2 in, 2 out]
            n222 = property on="Op_B" class="Ring (strict)"("Strings []"=w572) -> ()  [unwired: 2 in, 2 out]
            n223 = local read "All array"() -> (w575:bool[])
            n224 = local read "Type"() -> (w573:u16)
            n225 = Index Array(array=w580, index #1=0 ("index"), index #2=5 ("index")) -> (element #1=w578:string, element #2=w576:string)
            n226 = Index Array(array=w575, index=w573) -> (element=w574:bool)
            n227 = property on="Value_B" class="Str"("Caption.Text"=w578) -> ()  [unwired: 2 in, 2 out]
            n228 = property on="Operand_B" class="Bool (strict)"("Caption.Text"=w576) -> ()  [unwired: 2 in, 2 out]
            n229 = property on="All" class="Bool (strict)"("Val(Sgnl)"=w574) -> ()  [unwired: 2 in, 2 out]
          }
          frame 6 {
            # "User Equation"
            n230 = property on="SW_EdtObj" class="DigNum (strict)"("Val(Sgnl)"=w597) -> ()  [unwired: 2 in, 2 out]
            n231 = global read "CRYPost Processing Global.vi" "User Equation VI Ref"() -> (w595:refnum<vi>)
            n232 = local read "User Equation String"() -> (w602:string)
            n233 = Not A Number/Path/Refnum?(number/path/refnum=w595) -> (NaN/Path/Refnum?=w596:bool)
            n234 = call "CRYUnflatten User Equation Cluster.vi"("Flatten user equation cluster string"=w602) -> ("User Equation Cluster"=w601:T2)  [unwired: 8 in, 2 out]
            n235 = Unbundle By Name(w601) -> ("equation"=w598:string, "# input curves"=w600:i32, "# Desired result curves"=w599:i32)
            n236 = case shown="False" w596 {
              tunnel: w595 -> [w606 _]
              frame False {
                n237 = call "CRYGet Boolean Reference.vi"("Label Name"="CurLibChange", "VI Refnum"=w606) -> ("Boolean Ref"=w604:refnum<vi>)  [unwired: 7 in, 2 out]
                n238 = property class="Bool"(reference=w604, "Val(Sgnl)"=TRUE ("Loading_F")) -> ()  [unwired: 1 in, 2 out]
              }
              frame True {
              }
            }
            n239 = local write "#Desired Results"(w599) -> ()
            n240 = local write "#Operands"(w600) -> ()
            n241 = property on="Equ_List" class="Str"("Value"=w598) -> ()  [unwired: 2 in, 2 out]
          }
          frame 7 {
            # "Windowing"
            n242 = property on="SW_EdtObj" class="DigNum (strict)"("Val(Sgnl)"=w607) -> ()  [unwired: 2 in, 2 out]
            n243 = local read "A_cur name"() -> (w617:string)
            n244 = local read "All array"() -> (w611:bool[])
            n245 = local read "Type"() -> (w609:u16)
            n246 = Search 1D Array(1D array=w608, element=w617) -> (index of element=w613:i32)  [unwired: 1 out]
            n247 = property on="Op_A2" class="Ring (strict)"("Strings []"=w608) -> ()  [unwired: 2 in, 2 out]
            n248 = Index Array(array=w611, index=w609) -> (element=w610:bool)
            n249 = Equal?(x=-1 ("y"), y=w613) -> (x = y?=w616:bool)
            n250 = Select(t=0 ("y"), s=w616, f=w613) -> (s? t:f=w612:i32)
            n251 = property on="All" class="Bool (strict)"("Val(Sgnl)"=w610) -> ()  [unwired: 2 in, 2 out]
            n252 = property on="Op_A2" class="Ring (strict)"("Val(Sgnl)"=w612) -> ()  [unwired: 2 in, 2 out]
          }
          frame 8, 10 {
            # "Resolution & 1/n Octave Synthesis"
            n253 = flat-sequence {
              tunnel: w620 -> [w622]
              tunnel: w619 -> [w623]
              frame #0 {
                n254 = property on="SW_EdtObj" class="DigNum (strict)"("Val(Sgnl)"=w622) -> ()  [unwired: 2 in, 2 out]
              }
              frame #1 {
                n255 = local read "New_res str"() -> (w626:string)
                n256 = local read "A_cur name"() -> (w635:string)
                n257 = property on="New Resolution" class="Ring (strict)"() -> ("Strings []"=w624:string[])  [unwired: 2 in, 2 out]
                n258 = property on="Op_A2" class="Ring (strict)"("Strings []"=w623) -> ()  [unwired: 2 in, 2 out]
                n259 = Search 1D Array(1D array=w624, element=w626) -> (index of element=w630:i32)  [unwired: 1 out]
                n260 = Search 1D Array(1D array=w623, element=w635) -> (index of element=w632:i32)  [unwired: 1 out]
                n261 = Equal?(x=-1 ("y"), y=w630) -> (x = y?=w628:bool)
                n262 = Equal?(x=-1 ("y"), y=w632) -> (x = y?=w634:bool)
                n263 = Select(t=0 ("y"), s=w628, f=w630) -> (s? t:f=w625:i32)
                n264 = Select(t=0 ("y"), s=w634, f=w632) -> (s? t:f=w631:i32)
                n265 = property on="New Resolution" class="Ring (strict)"("Val(Sgnl)"=w625) -> ()  [unwired: 2 in, 2 out]
                n266 = property on="Op_A2" class="Ring (strict)"("Val(Sgnl)"=w631) -> ()  [unwired: 2 in, 2 out]
              }
            }
            n267 = case shown="10" w620 {
              tunnel: [w637 w638] -> w621
              tunnel: w618 -> [w637 w641]
              frame 8, Default {
              }
              frame 10 {
                n268 = Array Subset(array=w641, index=0, length=5) -> (w638:string[])
              }
            }
            n269 = property on="New Resolution" class="Ring (strict)"("Strings []"=w621) -> ()  [unwired: 2 in, 2 out]
          }
          frame 9 {
            # "Directivity Index"
            n270 = property on="Curve List" class="LstBox (strict)"("Item Names"=w656) -> ()  [unwired: 2 in, 2 out]
            n271 = property on="Weight Curve_2" class="Ring (strict)"("Strings []"=w656) -> ()  [unwired: 2 in, 2 out]
            n272 = property on="Ref_Curve" class="Ring (strict)"("Strings []"=w656) -> ()  [unwired: 2 in, 2 out]
            n273 = flat-sequence {
              tunnel: w642 -> [w657]
              frame #0 {
                n274 = property on="SW_EdtObj" class="DigNum (strict)"("Val(Sgnl)"=w657) -> ()  [unwired: 2 in, 2 out]
              }
              frame #1 {
                n275 = local read "Direct_weight"() -> (w658:bool)
                n276 = property on="Direct_weight" class="Bool (strict)"("Val(Sgnl)"=w658) -> ()  [unwired: 2 in, 2 out]
              }
            }
            n277 = local read "A_cur name"() -> (w652:string)
            n278 = local read "Weight_Cur array"() -> (w655:string[])
            n279 = Index Array(array=w655, index=w642) -> (element=w654:string)
            n280 = Search 1D Array(1D array=w656, element=w654) -> (index of element=w644:i32)  [unwired: 1 out]
            n281 = Search 1D Array(1D array=w656, element=w652) -> (index of element=w649:i32)  [unwired: 1 out]
            n282 = Equal?(x=-1 ("y"), y=w644) -> (x = y?=w646:bool)
            n283 = Equal?(x=-1 ("y"), y=w649) -> (x = y?=w651:bool)
            n284 = Select(t=0 ("y"), s=w646, f=w644) -> (s? t:f=w643:i32)
            n285 = Select(t=0 ("y"), s=w651, f=w649) -> (s? t:f=w648:i32)
            n286 = property on="Weight Curve_2" class="Ring (strict)"("Val(Sgnl)"=w643) -> ()  [unwired: 2 in, 2 out]
            n287 = property on="Ref_Curve" class="Ring (strict)"("Val(Sgnl)"=w648) -> ()  [unwired: 2 in, 2 out]
          }
          frame 11 {
            # "Resampling"
            n288 = property on="SW_EdtObj" class="DigNum (strict)"("Val(Sgnl)"=w659) -> ()  [unwired: 2 in, 2 out]
            n289 = local read "A_cur name"() -> (w661:string)
            n290 = property on="Op_A2" class="Ring (strict)"("Strings []"=w660) -> ()  [unwired: 2 in, 2 out]
            n291 = Search 1D Array(1D array=w660, element=w661) -> (index of element=w665:i32)  [unwired: 1 out]
            n292 = Equal?(x=-1 ("y"), y=w665) -> (x = y?=w662:bool)
            n293 = Select(t=0 ("y"), s=w662, f=w665) -> (s? t:f=w666:i32)
            n294 = property on="Op_A2" class="Ring (strict)"("Val(Sgnl)"=w666) -> ()  [unwired: 2 in, 2 out]
          }
          frame 12 {
            # "Frequency Shift"
            n295 = property on="SW_EdtObj" class="DigNum (strict)"("Val(Sgnl)"=w667) -> ()  [unwired: 2 in, 2 out]
            n296 = property on="Op_A2" class="Ring (strict)"("Strings []"=w681) -> ()  [unwired: 2 in, 2 out]
            n297 = property on="Ref Wave" class="Ring (strict)"("Strings []"=w681) -> ()  [unwired: 2 in, 2 out]
            n298 = local read "Ref Waveform"() -> (w669:string)
            n299 = local read "A_cur name"() -> (w676:string)
            n300 = local read "Ref Freq Mode"() -> (w674:u16)
            n301 = Search 1D Array(1D array=w681, element=w676) -> (index of element=w680:i32)  [unwired: 1 out]
            n302 = Search 1D Array(1D array=w681, element=w669) -> (index of element=w670:i32)  [unwired: 1 out]
            n303 = Equal?(x=-1 ("y"), y=w680) -> (x = y?=w677:bool)
            n304 = Equal?(x=-1 ("y"), y=w670) -> (x = y?=w673:bool)
            n305 = Select(t=0 ("y"), s=w677, f=w680) -> (s? t:f=w675:i32)
            n306 = Select(t=0 ("y"), s=w673, f=w670) -> (s? t:f=w668:i32)
            n307 = property on="Ref Freq Mode" class="Slide (strict)"("Val(Sgnl)"=w674) -> ()  [unwired: 2 in, 2 out]
            n308 = property on="Op_A2" class="Ring (strict)"("Val(Sgnl)"=w675) -> ()  [unwired: 2 in, 2 out]
            n309 = property on="Ref Wave" class="Ring (strict)"("Value"=w668) -> ()  [unwired: 2 in, 2 out]
          }
          frame 13 {
            # "Boolean"
            n310 = property on="SW_EdtObj" class="DigNum (strict)"("Val(Sgnl)"=w687) -> ()  [unwired: 2 in, 2 out]
            n311 = call "CRYGet Upper Step Data.vi"("Type In"=enum16{"Curves", "Values", "Results", "WFM"}."Results", "No.VI"=w685) -> ("Result array"=w684:T12)  [unwired: 9 out]
            n312 = for {
              tunnel: w684 -> [w689] mode=indexing
              tunnel: [w688] -> w683 mode=indexing
              n313 = Unbundle By Name(w689) -> ("Name"=w688:string)
            }
            n314 = property on="Result Listbox" class="LstBox (strict)"("Item Names"=w683) -> ()  [unwired: 2 in, 2 out]
            n315 = property on="Result Listbox" class="LstBox (strict)"("Top Row"=0) -> ()  [unwired: 2 in, 2 out]
          }
        }
        n316 = local read "Show xyz"() -> (w468:cluster{"x":bool, "y":bool, "z":bool}[])
        n317 = Equal?(x=w449, y=u16 6) -> (x = y?=w466:bool)
        n318 = local read "Loading_F"() -> (w455:bool)
        n319 = Index Array(array=w468, index=w449) -> (element=w469:cluster{"x":bool, "y":bool, "z":bool})
        n320 = property class="VI"(reference=w467, "Front Panel.Open"=w466) -> ()  [unwired: 1 in, 2 out]
        n321 = Unbundle By Name(w469) -> ("x"=w473:bool, "y"=w472:bool, "z"=w471:bool)
        n322 = property on="Loading_F" class="Bool (strict)"("Val(Sgnl)"=w455) -> ()  [unwired: 2 in, 2 out]
        n323 = case shown="False" w466 {
          tunnel: w471 -> [w690 w693]
          tunnel: w472 -> [w691 w694]
          tunnel: w473 -> [w692 w695]
          frame False {
            n324 = local write "z_1"(w690) -> ()
            n325 = local write "x_1"(w692) -> ()
            n326 = local write "y_1"(w691) -> ()
          }
          frame True {
            n327 = local write "z_2"(w693) -> ()
            n328 = local write "x_2"(w695) -> ()
            n329 = local write "y_2"(w694) -> ()
          }
        }
      }
      event "Op_A1": Value Change {
        n330 = event-data() -> ("OldVal"=w702:u16, "NewVal"=w701:u16)  [unwired: 5 out]
        n331 = call "CRYGetPost Pro_all data.vi"("No.VI"=w696) -> ("Curve array"=w712:T6, "Value array"=w711:T6, "All Names"=w708:string[], "C&W Names"=w716:string[], "Value Names"=w715:string[], "Waveform Array"=w710:T14, "Curve Names"=w709:string[], "Type array"=w713:enum16{"Curves", "Values", "Results", "WFM"}[], "Wave names"=w714:string[])  [unwired: 1 in, 5 out]
        n332 = local read "Type"() -> (w717:u16)
        n333 = local read "Post Processing"() -> (w707:T1)
        n334 = Index Array(array=w708, index=w701) -> (element=w703:string)
        n335 = Index Array(array=w713, index=w701) -> (element=w704:enum16{"Curves", "Values", "Results", "WFM"})
        n336 = case shown="2" w717 {
          selector: w717 -> [_ w779 w795 w850]
          tunnel: w704 -> [w731 w785 w789 w849]
          tunnel: w703 -> [w730 _ w801 w855]
          tunnel: w716 -> [_ _ w799 w854]
          tunnel: w715 -> [w738 _ _ _]
          tunnel: w714 -> [w737 _ w798 w853]
          tunnel: w712 -> [w735 _ w797 w852]
          tunnel: w711 -> [w734 _ _ _]
          tunnel: w710 -> [w733 _ w796 w851]
          tunnel: w709 -> [w732 _ _ _]
          tunnel: w707 -> [_ _ _ _]
          frame 0, Default {
            n337 = local read "Work in"() -> (w727:u16)
            n338 = case shown="\"Values\"" w731 {
              selector: w731 -> [w745 w758 w771]
              tunnel: [w743 w757 w770] -> w736
              tunnel: w738 -> [_ w763 _]
              tunnel: w730 -> [w751 w762 w778]
              tunnel: [w744 w755 w769] -> w729
              tunnel: w737 -> [_ _ w777]
              tunnel: w735 -> [w749 _ _]
              tunnel: w734 -> [_ w761 _]
              tunnel: w733 -> [_ _ w775]
              tunnel: w732 -> [w748 _ _]
              tunnel: [w742 w756 w768] -> w728
              tunnel: w727 -> [w741 w760 w773]
              tunnel: [w739 w753 w766] -> w725
              tunnel: [w740 w752 w767] -> w726
              frame "Curves", Default {
                n339 = Search 1D Array(1D array=w748, element=w751) -> (index of element=w750:i32)  [unwired: 1 out]
                n340 = Index Array(array=w749, index=w750) -> (element=w747:T7)
                n341 = call "CRYChange post_xyz mode.vi"("Work in"=w741, "Curve In"=w747, "XYZ Mode In"=u16 1, "Type In"=w745) -> ("Value"=w740:dbl, "Tip Out"=w742:string, "Unit Out"=w744:string, "Value Out"=w743:string, "Is Val&log"=w739:u16)  [unwired: 2 in, 1 out]
              }
              frame "Values" {
                n342 = Search 1D Array(1D array=w763, element=w762) -> (index of element=w765:i32)  [unwired: 1 out]
                n343 = Decrement(x=w765) -> (x-1=w764:i32)
                n344 = Index Array(array=w761, index=w764) -> (element=w754:T7)
                n345 = call "CRYChange post_xyz mode.vi"("Work in"=w760, "Value In"=w754, "XYZ Mode In"=u16 1, "Type In"=w758) -> ("Value"=w752:dbl, "Tip Out"=w756:string, "Unit Out"=w755:string, "Value Out"=w757:string, "Is Val&log"=w753:u16)  [unwired: 2 in, 1 out]
              }
              frame "WFM" {
                n346 = Search 1D Array(1D array=w777, element=w778) -> (index of element=w776:i32)  [unwired: 1 out]
                n347 = Index Array(array=w775, index=w776) -> (element=w772:T15)
                n348 = call "CRYChange post_xyz mode.vi"("Wave In"=w772, "Work in"=w773, "XYZ Mode In"=u16 1, "Type In"=w771) -> ("Value"=w767:dbl, "Tip Out"=w768:string, "Unit Out"=w769:string, "Value Out"=w770:string, "Is Val&log"=w766:u16)  [unwired: 2 in, 1 out]
              }
            }
            n349 = Greater Than 0?(x=w725) -> (x > 0?=w723:bool)
            n350 = local write "Value_A"(w736) -> ()
            n351 = local write "unit_A"(w729) -> ()
            n352 = local write "A log/lin"(w725) -> ()
            n353 = property on="Value_A" class="Str"("TipStrip"=w728) -> ()  [unwired: 2 in, 2 out]
            n354 = Select(t=w726, s=w723, f=nan) -> (s? t:f=w722:dbl)
            n355 = local write "tmp Val_A"(w722) -> ()
            n356 = property on="Work in" class="Slide (strict)"("TipStrip"="") -> ()  [unwired: 2 in, 2 out]
          }
          frame 1 {
            n357 = local read "A_xyz array"() -> (w781:u16[])
            n358 = Equal?(x=w785, y=enum16{"Curves", "Values", "Results", "WFM"}."WFM") -> (x = y?=w783:bool)
            n359 = Index Array(array=w781, index=w779) -> (element=w780:u16)
            n360 = case shown="False" w783 {
              tunnel: [string[] ["x", "y", "z"] ("Text Labels[]") string[] ["x0", "dx", "y"] ("Text Labels[]")] -> w782
              frame False {
              }
              frame True {
              }
            }
            n361 = property on="Mode_A" class="Slide (strict)"("Val(Sgnl)"=w780) -> ()  [unwired: 2 in, 2 out]
            n362 = property on="Mode_A" class="Slide (strict)"("TextLbls[]"=w782) -> ()  [unwired: 2 in, 2 out]
          }
          frame 2 {
            n363 = local read "Search Items"() -> (w790:string[])
            n364 = Equal?(x=w789, y=enum16{"Curves", "Values", "Results", "WFM"}."Values") -> (x = y?=w800:bool)
            n365 = property on="Mode_A" class="Slide (strict)"("Visible"=w800) -> ()  [unwired: 2 in, 2 out]
            n366 = call "CRYSet Search Ranges.vi"("Search Items"=w790, "Type"=w789) -> ("Checks"=w788:bool[], "Caption"=w792:string, "Item Names"=w793:string[], "Symbols"=w794:i32[])  [unwired: 6 out]
            n367 = property on="Search List" class="LstBox (strict)"("Item Symbols"=w794, "Item Names"=w793, "Caption.Text"=w792, "Value"=-1 ("Search List")) -> ()  [unwired: 2 in, 2 out]
            n368 = case shown="False" w800 {
              tunnel: w789 -> [w804 _]
              tunnel: w801 -> [w807 _]
              tunnel: w799 -> [w809 _]
              tunnel: w798 -> [w808 _]
              tunnel: w797 -> [w806 _]
              tunnel: w796 -> [w805 _]
              tunnel: w795 -> [_ w846]
              tunnel: w788 -> [w803 w844]
              frame False {
                n369 = case shown="\"Curves\", Default" w804 {
                  tunnel: w807 -> [w824 w840]
                  tunnel: w809 -> [w823 _]
                  tunnel: w808 -> [_ w841]
                  tunnel: w806 -> [w822 _]
                  tunnel: w805 -> [_ w839]
                  tunnel: w803 -> [w810 w827]
                  frame "Curves", Default {
                    n370 = Search 1D Array(1D array=w823, element=w824) -> (index of element=w826:i32)  [unwired: 1 out]
                    n371 = local write "Check_Hz"(w810) -> ()
                    n372 = Index Array(array=w822, index=w826) -> (element=w825:T7)
                    n373 = Unbundle By Name(w825) -> ("Y data"=w819:u16, "Y unit"=w818:string, "Curve"=w813:cluster{"x":dbl, "y":dbl, "z":dbl}[])
                    n374 = Equal To 0?(x=w819) -> (x = 0?=w821:bool)
                    n375 = Array Size(array=w813) -> (size(s)=w815:i32)
                    n376 = Select(t="dB" ("Y unit"), s=w821, f=w818) -> (s? t:f=w817:string)
                    n377 = Equal To 0?(x=w815) -> (x = 0?=w814:bool)
                    n378 = Select(t="No data" ("f"), s=w814, f="Curve") -> (s? t:f=w811:string)
                    n379 = local write "Value_A"(w811) -> ()
                    n380 = local write "unit_A"(w817) -> ()
                  }
                  frame "WFM" {
                    n381 = Search 1D Array(1D array=w841, element=w840) -> (index of element=w843:i32)  [unwired: 1 out]
                    n382 = Index Array(array=w839, index=w843) -> (element=w842:T15)
                    n383 = local write "Check_s"(w827) -> ()
                    n384 = Unbundle By Name(w842) -> ("Y data"=w830:u16, "Y unit"=w828:string, "Waveform.Y"=w835:sgl[])
                    n385 = Array Size(array=w835) -> (size(s)=w837:i32)
                    n386 = Equal To 0?(x=w830) -> (x = 0?=w829:bool)
                    n387 = Equal To 0?(x=w837) -> (x = 0?=w836:bool)
                    n388 = Select(t="dB" ("Y unit"), s=w829, f=w828) -> (s? t:f=w831:string)
                    n389 = Select(t="No data" ("f"), s=w836, f="Waveform") -> (s? t:f=w833:string)
                    n390 = local write "unit_A"(w831) -> ()
                    n391 = local write "Value_A"(w833) -> ()
                  }
                }
              }
              frame True {
                n392 = local write "Check_Hz"(w844) -> ()
                n393 = local read "A_xyz array"() -> (w848:u16[])
                n394 = Index Array(array=w848, index=w846) -> (element=w847:u16)
                n395 = property on="Mode_A" class="Slide (strict)"("Val(Sgnl)"=w847, "TextLbls[]"=string[] ["x", "y", "z"] ("Text Labels[]")) -> ()  [unwired: 2 in, 2 out]
              }
            }
          }
          frame 5 {
            n396 = stacked-sequence {
              tunnel: w855 -> [_ w873]
              tunnel: w854 -> [_ w872]
              tunnel: w853 -> [_ w871]
              tunnel: w852 -> [_ w870]
              tunnel: w851 -> [_ w869]
              tunnel: w850 -> [_ w868]
              tunnel: w849 -> [w856 w867]
              frame #0 {
                n397 = local read "Search Items"() -> (w860:string[])
                n398 = Equal?(x=w856, y=enum16{"Curves", "Values", "Results", "WFM"}."WFM") -> (x = y?=w863:bool)
                n399 = call "CRYSet Search Ranges.vi"("Search Items"=w860, "Type"=w856) -> ("Checks"=w859:bool[], "Caption"=w857:string, "Item Names"=w858:string[], "Symbols"=w861:i32[])  [unwired: 6 out]
                n400 = property on="Search List" class="LstBox (strict)"("Item Symbols"=w861, "Item Names"=w858, "Caption.Text"=w857, "Value"=-1 ("Search List")) -> ()  [unwired: 2 in, 2 out]
                n401 = case shown="True" w863 {
                  tunnel: w859 -> [w865 w866]
                  frame False {
                    n402 = local write "Check_Hz"(w865) -> ()
                  }
                  frame True {
                    n403 = local write "Check_s"(w866) -> ()
                  }
                }
              }
              frame #1 {
                n404 = Equal?(x=w867, y=enum16{"Curves", "Values", "Results", "WFM"}."Values") -> (x = y?=w874:bool)
                n405 = case shown="False" w874 {
                  tunnel: w867 -> [w886 _]
                  tunnel: w873 -> [w885 _]
                  tunnel: w872 -> [w884 _]
                  tunnel: w871 -> [w883 _]
                  tunnel: w870 -> [w881 _]
                  tunnel: w869 -> [w880 _]
                  tunnel: w868 -> [_ w908]
                  frame False {
                    n406 = local read "Work in"() -> (w879:u16)
                    n407 = case shown="\"Curves\", Default" w886 {
                      selector: w886 -> [w891 w900]
                      tunnel: [w888 w898] -> w877
                      tunnel: w885 -> [w896 w906]
                      tunnel: [w889 w899] -> w878
                      tunnel: w884 -> [w895 _]
                      tunnel: w883 -> [_ w905]
                      tunnel: w881 -> [w893 _]
                      tunnel: w880 -> [_ w903]
                      tunnel: w879 -> [w892 w902]
                      frame "Curves", Default {
                        n408 = Search 1D Array(1D array=w895, element=w896) -> (index of element=w894:i32)  [unwired: 1 out]
                        n409 = Index Array(array=w893, index=w894) -> (element=w890:T7)
                        n410 = call "CRYChange post_xyz mode.vi"("Work in"=w892, "Curve In"=w890, "XYZ Mode In"=u16 1, "Type In"=w891) -> ("Unit Out"=w888:string, "Value Out"=w889:string)  [unwired: 2 in, 4 out]
                      }
                      frame "WFM" {
                        n411 = Search 1D Array(1D array=w905, element=w906) -> (index of element=w904:i32)  [unwired: 1 out]
                        n412 = Index Array(array=w903, index=w904) -> (element=w901:T15)
                        n413 = call "CRYChange post_xyz mode.vi"("Wave In"=w901, "Work in"=w902, "XYZ Mode In"=u16 1, "Type In"=w900) -> ("Unit Out"=w898:string, "Value Out"=w899:string)  [unwired: 2 in, 4 out]
                      }
                    }
                    n414 = local write "Value_A"(w878) -> ()
                    n415 = local write "unit_A"(w877) -> ()
                    n416 = property on="Mode_A" class="Slide (strict)"("Visible"=FALSE) -> ()  [unwired: 2 in, 2 out]
                    n417 = property on="Value_A" class="Str"("TipStrip"="") -> ()  [unwired: 2 in, 2 out]
                  }
                  frame True {
                    n418 = local read "A_xyz array"() -> (w909:u16[])
                    n419 = Index Array(array=w909, index=w908) -> (element=w907:u16)
                    n420 = property on="Mode_A" class="Slide (strict)"("Val(Sgnl)"=w907, "Visible"=TRUE, "TextLbls[]"=string[] ["x", "y", "z"] ("Text Labels[]")) -> ()  [unwired: 2 in, 2 out]
                  }
                }
              }
            }
          }
        }
        n421 = local read "Post Processing"() -> (w706:T1)
        n422 = local write "A_cur name"(w703) -> ()
        n423 = Bundle By Name(cluster=w706, "Curve A"=w703, "Type A"=w704) -> (w705:T1)
        n424 = local write "Post Processing"(w705) -> ()
        n425 = local read "Loading_F"() -> (w698:bool)
        n426 = Not Equal?(x=w702, y=w701) -> (x != y?=w699:bool)
        n427 = Not(x=w698) -> (.not. x?=w697:bool)
        n428 = And(x=w699, y=w697) -> (x .and. y?=w700:bool)
        n429 = case shown="True" w700 {
          frame True {
            n430 = local read "Custom unit info"() -> (w719:T3)
            n431 = Unbundle By Name(w719) -> ("use custom"=w718:bool)
            n432 = case shown="False" w718 {
              frame False {
                n433 = local write "Unit String"("") -> ()
              }
              frame True {
              }
            }
          }
          frame False {
          }
        }
      }
      event "Mode_A": Value Change {
        n434 = event-data() -> ("NewVal"=w913:u16)  [unwired: 6 out]
        n435 = local read "Op_A1"() -> (w929:u16)
        n436 = property on="Op_A1" class="Ring (strict)"() -> ("RingText.Text"=w926:string)  [unwired: 2 in, 2 out]
        n437 = call "CRYGetPost Pro_all data.vi"("No.VI"=w912) -> ("Curve array"=w920:T6, "Value array"=w921:T6, "All Names"=w916:string[], "C&W Names"=w922:string[], "Value Names"=w918:string[], "Waveform Array"=w919:T14, "Type array"=w928:enum16{"Curves", "Values", "Results", "WFM"}[], "Wave names"=w917:string[])  [unwired: 1 in, 6 out]
        n438 = local read "Type"() -> (w930:u16)
        n439 = Index Array(array=w928, index=w929) -> (element=w927:enum16{"Curves", "Values", "Results", "WFM"})
        n440 = case shown="1, Default" w930 {
          selector: w930 -> [_ w1015]
          tunnel: w927 -> [w945 _]
          tunnel: w926 -> [w944 w1031]
          tunnel: w913 -> [w943 w1030]
          tunnel: w922 -> [w940 _]
          tunnel: w921 -> [w939 w1023]
          tunnel: w920 -> [w938 _]
          tunnel: w919 -> [w937 _]
          tunnel: w918 -> [w935 w1026]
          tunnel: w917 -> [w936 _]
          tunnel: w916 -> [_ w1012]
          frame 1, Default {
            n441 = local read "Work in"() -> (w934:u16)
            n442 = case shown="\"WFM\"" w945 {
              selector: w945 -> [w970 w991 w1008]
              tunnel: w944 -> [w971 w992 w1009]
              tunnel: w943 -> [w968 w989 w1006]
              tunnel: [w959 w977 w997] -> w942
              tunnel: [w969 w990 w1007] -> w941
              tunnel: w940 -> [w967 _ _]
              tunnel: w939 -> [_ w984 _]
              tunnel: w938 -> [w966 _ _]
              tunnel: w937 -> [_ _ w1004]
              tunnel: w935 -> [_ w987 _]
              tunnel: w936 -> [_ _ w1005]
              tunnel: w934 -> [w958 w976 w996]
              tunnel: [w957 w975 w995] -> w933
              tunnel: [w955 w974 w993] -> w931
              tunnel: [w956 w973 w994] -> w932
              frame "Curves", Default {
                n443 = Search 1D Array(1D array=w967, element=w971) -> (index of element=w972:i32)  [unwired: 1 out]
                n444 = Index Array(array=w966, index=w972) -> (element=w965:T7)
                n445 = call "CRYChange post_xyz mode.vi"("Work in"=w958, "Curve In"=w965, "XYZ Mode In"=w968, "Type In"=w970) -> ("Value"=w956:dbl, "Tip Out"=w957:string, "Unit Out"=w969:string, "Value Out"=w960:string, "Is Val&log"=w955:u16)  [unwired: 2 in, 1 out]
                n446 = Unbundle By Name(w965) -> ("Curve"=w961:cluster{"x":dbl, "y":dbl, "z":dbl}[])
                n447 = Array Size(array=w961) -> (size(s)=w963:i32)
                n448 = Equal To 0?(x=w963) -> (x = 0?=w964:bool)
                n449 = Select(t="No data" ("f"), s=w964, f=w960) -> (s? t:f=w959:string)
              }
              frame "Values" {
                n450 = Delete From Array(array=w987, index=0) -> (array with subset deleted=w985:string[])  [unwired: 1 in, 1 out]
                n451 = Search 1D Array(1D array=w985, element=w992) -> (index of element=w988:i32)  [unwired: 1 out]
                n452 = Index Array(array=w984, index=w988) -> (element=w979:T7)
                n453 = call "CRYChange post_xyz mode.vi"("Work in"=w976, "Value In"=w979, "XYZ Mode In"=w989, "Type In"=w991) -> ("Value"=w973:dbl, "Tip Out"=w975:string, "Unit Out"=w990:string, "Value Out"=w978:string, "Is Val&log"=w974:u16)  [unwired: 2 in, 1 out]
                n454 = Unbundle By Name(w979) -> ("Curve"=w980:cluster{"x":dbl, "y":dbl, "z":dbl}[])
                n455 = Array Size(array=w980) -> (size(s)=w982:i32)
                n456 = Equal To 0?(x=w982) -> (x = 0?=w983:bool)
                n457 = Select(t="No data" ("f"), s=w983, f=w978) -> (s? t:f=w977:string)
              }
              frame "WFM" {
                n458 = Search 1D Array(1D array=w1005, element=w1009) -> (index of element=w1010:i32)  [unwired: 1 out]
                n459 = Index Array(array=w1004, index=w1010) -> (element=w1003:T15)
                n460 = Unbundle By Name(w1003) -> ("Waveform.Y"=w999:sgl[])
                n461 = call "CRYChange post_xyz mode.vi"("Wave In"=w1003, "Work in"=w996, "XYZ Mode In"=w1006, "Type In"=w1008) -> ("Value"=w994:dbl, "Tip Out"=w995:string, "Unit Out"=w1007:string, "Value Out"=w998:string, "Is Val&log"=w993:u16)  [unwired: 2 in, 1 out]
                n462 = Array Size(array=w999) -> (size(s)=w1001:i32)
                n463 = Equal To 0?(x=w1001) -> (x = 0?=w1002:bool)
                n464 = Select(t="No data" ("f"), s=w1002, f=w998) -> (s? t:f=w997:string)
              }
            }
            n465 = flat-sequence {
              tunnel: w942 -> [w953]
              tunnel: w941 -> [w952]
              tunnel: w933 -> [w951]
              tunnel: w932 -> [w950]
              tunnel: w931 -> [w946]
              frame #0 {
                n466 = Greater Than 0?(x=w946) -> (x > 0?=w947:bool)
                n467 = local write "Value_A"(w953) -> ()
                n468 = local write "unit_A"(w952) -> ()
                n469 = property on="Value_A" class="Str"("TipStrip"=w951) -> ()  [unwired: 2 in, 2 out]
                n470 = local write "A log/lin"(w946) -> ()
                n471 = Select(t=w950, s=w947, f=nan) -> (s? t:f=w948:dbl)
                n472 = local write "tmp Val_A"(w948) -> ()
              }
              frame #1 {
                n473 = property on="Show Calcu" class="Bool (strict)"("Val(Sgnl)"=TRUE ("Value (Signaling)")) -> ()  [unwired: 2 in, 2 out]
              }
            }
          }
          frame 2, 5 {
            n474 = Delete From Array(array=w1026, index=0) -> (array with subset deleted=w1024:string[])  [unwired: 1 in, 1 out]
            n475 = Equal?(x=w1015, y=u16 2) -> (x = y?=w1013:bool)
            n476 = Search 1D Array(1D array=w1024, element=w1031) -> (index of element=w1029:i32)  [unwired: 1 out]
            n477 = case shown="False" w1013 {
              tunnel: w1012 -> [w1032 _]
              frame False {
                n478 = disable-structure shown="Enabled" {
                  disable-tunnel: w1032 -> [w1033 _]
                  frame Disabled {
                    n479 = local read "B_cur name"() -> (w1039:string)
                    n480 = Search 1D Array(1D array=w1033, element=w1039) -> (index of element=w1035:i32)  [unwired: 1 out]
                    n481 = Equal?(x=-1 ("y"), y=w1035) -> (x = y?=w1036:bool)
                    n482 = Select(t=0 ("y"), s=w1036, f=w1035) -> (s? t:f=w1034:i32)
                    n483 = property on="Op_B" class="Ring (strict)"("Val(Sgnl)"=w1034) -> ()  [unwired: 2 in, 2 out]
                  }
                  frame Enabled {
                  }
                }
              }
              frame True {
                n484 = disable-structure shown="Disabled" {
                  frame Disabled {
                    n485 = local read "Unary Operator"() -> (w1040:u16)
                    n486 = property on="Unary Operator" class="Ring (strict)"("Val(Sgnl)"=w1040) -> ()  [unwired: 2 in, 2 out]
                  }
                  frame Enabled {
                  }
                }
              }
            }
            n487 = Index Array(array=w1023, index=w1029) -> (element=w1022:T7)
            n488 = Unbundle By Name(w1022) -> ("Curve"=w1018:cluster{"x":dbl, "y":dbl, "z":dbl}[])
            n489 = call "CRYChange post_xyz mode.vi"("Value In"=w1022, "XYZ Mode In"=w1030, "Type In"=enum16{"Curves", "Values", "Results", "WFM"}."Values") -> ("Unit Out"=w1027:string, "Value Out"=w1017:string)  [unwired: 3 in, 4 out]
            n490 = Array Size(array=w1018) -> (size(s)=w1020:i32)
            n491 = Equal To 0?(x=w1020) -> (x = 0?=w1021:bool)
            n492 = Select(t="No data" ("f"), s=w1021, f=w1017) -> (s? t:f=w1016:string)
            n493 = local write "Value_A"(w1016) -> ()
            n494 = local write "unit_A"(w1027) -> ()
            n495 = property on="Value_A" class="Str"("TipStrip"="") -> ()  [unwired: 2 in, 2 out]
          }
        }
        n496 = local read "A_xyz array"() -> (w923:u16[])
        n497 = local read "Type"() -> (w925:u16)
        n498 = Replace Array Subset(array=w923, new element=w913, index=w925) -> (w924:u16[])
        n499 = local write "A_xyz array"(w924) -> ()
        n500 = local read "Post Processing"() -> (w914:T1)
        n501 = Bundle By Name(cluster=w914, "A_single val axis"=w913) -> (w915:T1)
        n502 = local write "Post Processing"(w915) -> ()
      }
      event "Op_B": Value Change {
        n503 = event-data() -> ("OldVal"=w1047:u16, "NewVal"=w1046:u16)  [unwired: 5 out]
        n504 = call "CRYGetPost Pro_all data.vi"("No.VI"=w1041) -> ("Curve array"=w1051:T6, "Value array"=w1052:T6, "All Names"=w1049:string[], "C&W Names"=w1058:string[], "Value Names"=w1054:string[], "Waveform Array"=w1050:T14, "Type array"=w1056:enum16{"Curves", "Values", "Results", "WFM"}[], "Wave names"=w1057:string[])  [unwired: 1 in, 6 out]
        n505 = local read "Type"() -> (w1055:u16)
        n506 = Index Array(array=w1056, index=w1046) -> (element=w1053:enum16{"Curves", "Values", "Results", "WFM"})
        n507 = Not Equal?(x=w1046, y=w1047) -> (x != y?=w1043:bool)
        n508 = Index Array(array=w1049, index=w1046) -> (element=w1048:string)
        n509 = local read "Loading_F"() -> (w1044:bool)
        n510 = case shown="1" w1055 {
          selector: w1055 -> [_ _ w1145]
          tunnel: w1053 -> [w1070 _ w1142]
          tunnel: w1058 -> [w1080 _ w1149]
          tunnel: w1054 -> [w1079 w1123 _]
          tunnel: w1057 -> [w1078 _ w1148]
          tunnel: w1046 -> [_ w1122 _]
          tunnel: w1052 -> [w1074 _ _]
          tunnel: w1051 -> [w1075 _ w1147]
          tunnel: w1050 -> [w1073 _ w1146]
          tunnel: w1049 -> [_ _ _]
          tunnel: w1048 -> [w1069 _ w1141]
          frame 0, Default {
            n511 = local read "Work in"() -> (w1068:u16)
            n512 = local read "Post Processing"() -> (w1071:T1)
            n513 = Bundle By Name(cluster=w1071, "Curve B"=w1069, "Type B"=w1070) -> (w1072:T1)
            n514 = local write "B_cur name"(w1069) -> ()
            n515 = local write "Post Processing"(w1072) -> ()
            n516 = case shown="\"Values\"" w1070 {
              selector: w1070 -> [w1086 w1101 w1114]
              tunnel: [w1085 w1099 w1113] -> w1077
              tunnel: [w1084 w1098 w1112] -> w1076
              tunnel: w1080 -> [w1092 _ _]
              tunnel: w1069 -> [w1091 w1105 w1119]
              tunnel: w1079 -> [_ w1104 _]
              tunnel: w1078 -> [_ _ w1118]
              tunnel: w1075 -> [w1090 _ _]
              tunnel: w1074 -> [_ w1103 _]
              tunnel: w1073 -> [_ _ w1117]
              tunnel: w1068 -> [w1089 w1102 w1116]
              tunnel: [w1083 w1097 w1111] -> w1067
              tunnel: [w1082 w1096 w1110] -> w1066
              tunnel: [w1081 w1095 w1109] -> w1065
              frame "Curves", Default {
                n517 = Search 1D Array(1D array=w1092, element=w1091) -> (index of element=w1093:i32)  [unwired: 1 out]
                n518 = Index Array(array=w1090, index=w1093) -> (element=w1088:T7)
                n519 = call "CRYChange post_xyz mode.vi"("Work in"=w1089, "Curve In"=w1088, "XYZ Mode In"=u16 1, "Type In"=w1086) -> ("Value"=w1082:dbl, "Tip Out"=w1083:string, "Unit Out"=w1084:string, "Value Out"=w1085:string, "Is Val&log"=w1081:u16)  [unwired: 2 in, 1 out]
              }
              frame "Values" {
                n520 = Search 1D Array(1D array=w1104, element=w1105) -> (index of element=w1107:i32)  [unwired: 1 out]
                n521 = Decrement(x=w1107) -> (x-1=w1106:i32)
                n522 = Index Array(array=w1103, index=w1106) -> (element=w1100:T7)
                n523 = call "CRYChange post_xyz mode.vi"("Work in"=w1102, "Value In"=w1100, "XYZ Mode In"=u16 1, "Type In"=w1101) -> ("Value"=w1096:dbl, "Tip Out"=w1097:string, "Unit Out"=w1098:string, "Value Out"=w1099:string, "Is Val&log"=w1095:u16)  [unwired: 2 in, 1 out]
              }
              frame "WFM" {
                n524 = Search 1D Array(1D array=w1118, element=w1119) -> (index of element=w1120:i32)  [unwired: 1 out]
                n525 = Index Array(array=w1117, index=w1120) -> (element=w1115:T15)
                n526 = call "CRYChange post_xyz mode.vi"("Wave In"=w1115, "Work in"=w1116, "XYZ Mode In"=u16 1, "Type In"=w1114) -> ("Value"=w1110:dbl, "Tip Out"=w1111:string, "Unit Out"=w1112:string, "Value Out"=w1113:string, "Is Val&log"=w1109:u16)  [unwired: 2 in, 1 out]
              }
            }
            n527 = Greater Than 0?(x=w1065) -> (x > 0?=w1062:bool)
            n528 = local write "Value_B"(w1077) -> ()
            n529 = local write "unit_B"(w1076) -> ()
            n530 = property on="Value_B" class="Str"("TipStrip"=w1067) -> ()  [unwired: 2 in, 2 out]
            n531 = Select(t=w1066, s=w1062, f=nan) -> (s? t:f=w1063:dbl)
            n532 = local write "tmp Val_B"(w1063) -> ()
          }
          frame 1 {
            n533 = Index Array(array=w1123, index=w1122) -> (element=w1121:string)
            n534 = local read "Post Processing"() -> (w1125:T1)
            n535 = Bundle By Name(cluster=w1125, "Curve B"=w1121, "Type B"=enum16{"Curves", "Values", "Results", "WFM"}."Values") -> (w1126:T1)
            n536 = local write "B_cur name"(w1121) -> ()
            n537 = local write "Post Processing"(w1126) -> ()
            n538 = Greater Or Equal?(x=w1122, y=u16 1) -> (x >= y?=w1127:bool)
            n539 = case shown="False" w1127 {
              frame False {
                w1132 = FALSE ("Visible")
                n540 = property on="Mode_B" class="Slide (strict)"("Visible"=w1132) -> ()  [unwired: 2 in, 2 out]
                n541 = local read "Work in"() -> (w1131:u16)
                n542 = local read "Constant"() -> (w1129:dbl)
                n543 = property on="Value_B" class="Str"("Visible"=w1132) -> ()  [unwired: 2 in, 2 out]
                n544 = property on="Constant" class="DigNum (strict)"("Visible"=TRUE) -> ()  [unwired: 2 in, 2 out]
                n545 = property on="unit_B" class="Str"("Visible"=w1132) -> ()  [unwired: 2 in, 2 out]
                n546 = call "CRYSet Constant to TipStrip.vi"("Work in"=w1131, "Constant"=w1129) -> ("Tip Out"=w1130:string)  [unwired: 9 in]
                n547 = property on="Constant" class="DigNum (strict)"("TipStrip"=w1130) -> ()  [unwired: 2 in, 2 out]
                n548 = flat-sequence {
                  tunnel: w1129 -> [w1134]
                  frame #0 {
                    n549 = local write "tmp Val_B"(w1134) -> ()
                  }
                  frame #1 {
                    n550 = property on="Show Calcu" class="Bool (strict)"("Val(Sgnl)"=TRUE ("Value (Signaling)")) -> ()  [unwired: 2 in, 2 out]
                  }
                }
              }
              frame True {
                w1140 = TRUE ("Visible")
                n551 = local read "B_xyz array"() -> (w1137:u16[])
                n552 = property on="Mode_B" class="Slide (strict)"("Visible"=w1140) -> ()  [unwired: 2 in, 2 out]
                n553 = property on="Constant" class="DigNum (strict)"("Visible"=FALSE) -> ()  [unwired: 2 in, 2 out]
                n554 = property on="Value_B" class="Str"("Visible"=w1140) -> ()  [unwired: 2 in, 2 out]
                n555 = Index Array(array=w1137, index=1) -> (element=w1138:u16)
                n556 = property on="unit_B" class="Str"("Visible"=w1140) -> ()  [unwired: 2 in, 2 out]
                n557 = property on="Mode_B" class="Slide (strict)"("Val(Sgnl)"=w1138) -> ()  [unwired: 2 in, 2 out]
              }
            }
          }
          frame 5 {
            n558 = local read "Post Processing"() -> (w1143:T1)
            n559 = Bundle By Name(cluster=w1143, "Curve B"=w1141, "Type B"=w1142) -> (w1144:T1)
            n560 = local write "B_cur name"(w1141) -> ()
            n561 = local write "Post Processing"(w1144) -> ()
            n562 = Equal?(x=w1142, y=enum16{"Curves", "Values", "Results", "WFM"}."Values") -> (x = y?=w1150:bool)
            n563 = property on="Mode_B" class="Slide (strict)"("Visible"=w1150) -> ()  [unwired: 2 in, 2 out]
            n564 = case shown="True" w1150 {
              tunnel: w1142 -> [w1159 _]
              tunnel: w1149 -> [w1162 _]
              tunnel: w1141 -> [w1161 _]
              tunnel: w1148 -> [w1160 _]
              tunnel: w1147 -> [w1158 _]
              tunnel: w1146 -> [w1157 _]
              tunnel: w1145 -> [_ w1183]
              frame False {
                n565 = local read "Work in"() -> (w1155:u16)
                n566 = case shown="\"Curves\", Default" w1159 {
                  selector: w1159 -> [w1166 w1178]
                  tunnel: w1162 -> [w1171 _]
                  tunnel: w1161 -> [w1170 w1180]
                  tunnel: w1160 -> [_ w1181]
                  tunnel: w1158 -> [w1169 _]
                  tunnel: w1157 -> [_ w1179]
                  tunnel: w1155 -> [w1168 w1177]
                  tunnel: [w1165 w1175] -> w1154
                  tunnel: [w1164 w1174] -> w1153
                  frame "Curves", Default {
                    n567 = Search 1D Array(1D array=w1171, element=w1170) -> (index of element=w1172:i32)  [unwired: 1 out]
                    n568 = Index Array(array=w1169, index=w1172) -> (element=w1167:T7)
                    n569 = call "CRYChange post_xyz mode.vi"("Work in"=w1168, "Curve In"=w1167, "XYZ Mode In"=u16 1, "Type In"=w1166) -> ("Unit Out"=w1164:string, "Value Out"=w1165:string)  [unwired: 2 in, 4 out]
                  }
                  frame "WFM" {
                    n570 = Search 1D Array(1D array=w1181, element=w1180) -> (index of element=w1182:i32)  [unwired: 1 out]
                    n571 = Index Array(array=w1179, index=w1182) -> (element=w1176:T15)
                    n572 = call "CRYChange post_xyz mode.vi"("Wave In"=w1176, "Work in"=w1177, "XYZ Mode In"=u16 1, "Type In"=w1178) -> ("Unit Out"=w1174:string, "Value Out"=w1175:string)  [unwired: 2 in, 4 out]
                  }
                }
                n573 = local read "Use default"() -> (w1156:bool)
                n574 = property on="Use default" class="Bool (strict)"("Val(Sgnl)"=w1156) -> ()  [unwired: 2 in, 2 out]
                n575 = local write "Value_B"(w1154) -> ()
                n576 = local write "unit_B"(w1153) -> ()
                n577 = property on="Value_B" class="Str"("TipStrip"="") -> ()  [unwired: 2 in, 2 out]
              }
              frame True {
                n578 = local read "B_xyz array"() -> (w1185:u16[])
                n579 = Index Array(array=w1185, index=w1183) -> (element=w1184:u16)
                n580 = property on="Mode_B" class="Slide (strict)"("Val(Sgnl)"=w1184) -> ()  [unwired: 2 in, 2 out]
              }
            }
          }
        }
        n581 = Not(x=w1044) -> (.not. x?=w1045:bool)
        n582 = And(x=w1043, y=w1045) -> (x .and. y?=w1042:bool)
        n583 = case shown="True" w1042 {
          frame True {
            n584 = local read "Custom unit info"() -> (w1060:T3)
            n585 = Unbundle By Name(w1060) -> ("use custom"=w1059:bool)
            n586 = case shown="False" w1059 {
              frame False {
                n587 = local write "Unit String"("") -> ()
              }
              frame True {
              }
            }
          }
          frame False {
          }
        }
      }
      event "Mode_B": Value Change {
        n588 = event-data() -> ("NewVal"=w1194:u16)  [unwired: 6 out]
        n589 = local read "Type"() -> (w1190:u16)
        n590 = call "CRYGetPost Pro_all data.vi"("No.VI"=w1193) -> ("Value array"=w1199:T6, "Value Names"=w1198:string[])  [unwired: 1 in, 12 out]
        n591 = property on="Op_B" class="Ring (strict)"() -> ("RingText.Text"=w1203:string)  [unwired: 2 in, 2 out]
        n592 = case shown="1, Default" w1190 {
          selector: w1190 -> [_ w1222]
          tunnel: [w1220 w1226] -> w1205
          tunnel: w1203 -> [w1221 w1224]
          tunnel: w1198 -> [w1219 w1223]
          frame 5 {
            n593 = Delete From Array(array=w1219, index=0) -> (array with subset deleted=w1217:string[])  [unwired: 1 in, 1 out]
            n594 = local read "Use default"() -> (w1216:bool)
            n595 = Search 1D Array(1D array=w1217, element=w1221) -> (index of element=w1220:i32)  [unwired: 1 out]
            n596 = property on="Use default" class="Bool (strict)"("Val(Sgnl)"=w1216) -> ()  [unwired: 2 in, 2 out]
          }
          frame 1, Default {
            n597 = disable-structure shown="Disabled" {
              disable-tunnel: w1222 -> [w1227 _]
              frame Disabled {
                n598 = local read "Ope_array"() -> (w1228:u16[])
                n599 = Index Array(array=w1228, index=w1227) -> (element=w1229:u16)
                n600 = property on="binary operation" class="Ring (strict)"("Val(Sgnl)"=w1229) -> ()  [unwired: 2 in, 2 out]
              }
              frame Enabled {
              }
            }
            n601 = Search 1D Array(1D array=w1223, element=w1224) -> (index of element=w1225:i32)  [unwired: 1 out]
            n602 = Decrement(x=w1225) -> (x-1=w1226:i32)
          }
        }
        n603 = Index Array(array=w1199, index=w1205) -> (element=w1197:T7)
        n604 = local read "B_xyz array"() -> (w1202:u16[])
        n605 = local read "Type"() -> (w1200:u16)
        n606 = local read "Work in"() -> (w1188:u16)
        n607 = call "CRYChange post_xyz mode.vi"("Work in"=w1188, "Value In"=w1197, "XYZ Mode In"=w1194, "Type In"=enum16{"Curves", "Values", "Results", "WFM"}."Values") -> ("Value"=w1187:dbl, "Tip Out"=w1192:string, "Unit Out"=w1206:string, "Value Out"=w1191:string, "Is Val&log"=w1186:u16)  [unwired: 2 in, 1 out]
        n608 = Replace Array Subset(array=w1202, new element=w1194, index=w1200) -> (w1201:u16[])
        n609 = case shown="1" w1190 {
          tunnel: w1192 -> [_ w1213]
          tunnel: ["" w1213] -> w1189
          tunnel: w1187 -> [_ w1210]
          tunnel: w1186 -> [_ w1211]
          frame 5, Default {
          }
          frame 1 {
            n610 = Greater Than 0?(x=w1211) -> (x > 0?=w1208:bool)
            n611 = Select(t=w1210, s=w1208, f=nan) -> (s? t:f=w1209:dbl)
            n612 = flat-sequence {
              tunnel: w1209 -> [w1214]
              frame #0 {
                n613 = local write "tmp Val_B"(w1214) -> ()
              }
              frame #1 {
                n614 = property on="Show Calcu" class="Bool (strict)"("Val(Sgnl)"=TRUE ("Value (Signaling)")) -> ()  [unwired: 2 in, 2 out]
              }
            }
          }
        }
        n615 = local write "B_xyz array"(w1201) -> ()
        n616 = local read "Post Processing"() -> (w1196:T1)
        n617 = Bundle By Name(cluster=w1196, "B_single val axis"=w1194) -> (w1195:T1)
        n618 = local write "Value_B"(w1191) -> ()
        n619 = local write "unit_B"(w1206) -> ()
        n620 = local write "Post Processing"(w1195) -> ()
        n621 = property on="Value_B" class="Str"("TipStrip"=w1189) -> ()  [unwired: 2 in, 2 out]
      }
      event "Use default": Value Change {
        n622 = event-data() -> ("NewVal"=w1235:bool)  [unwired: 6 out]
        n623 = disable-structure shown="Disabled" {
          disable-tunnel: w1230 -> [w1237 _]
          frame Disabled {
            n624 = local read "Statistical Operator"() -> (w1246:u16)
            n625 = local read "New Resolution"() -> (w1240:u16)
            n626 = local read "binary operation"() -> (w1257:u16)
            n627 = local read "Unary Operator"() -> (w1247:u16)
            n628 = call "CRYGetPost Pro_all data.vi"("No.VI"=w1237) -> ("C&W Type array"=w1245:enum16{"Curves", "Values", "Results", "WFM"}[], "All Names"=w1255:string[], "C&W Names"=w1244:string[], "Value Names"=w1251:string[], "Curve Names"=w1241:string[], "Type array"=w1254:enum16{"Curves", "Values", "Results", "WFM"}[], "Wave names"=w1238:string[])  [unwired: 1 in, 7 out]
            n629 = local read "Octav Mode"() -> (w1242:u16)
            n630 = local read "Ref_Curve"() -> (w1239:u16)
            n631 = local read "Mode_B"() -> (w1249:u16)
            n632 = local read "Op_A2"() -> (w1243:u16)
            n633 = local read "Mode_A"() -> (w1250:u16)
            n634 = local read "Op_B"() -> (w1253:u16)
            n635 = local read "Work in"() -> (w1248:u16)
            n636 = local read "Op_A1"() -> (w1256:u16)
            n637 = local read "Type"() -> (w1252:u16)
            n638 = case shown="8, 10" w1252 {
              selector: w1252 -> [w1258 w1283 w1295 w1303 w1312 w1326 w1334 w1340 w1349 w1357]
              tunnel: w1248 -> [w1270 w1285 _ _ _ _ _ _ _ _]
              tunnel: [w1269 w1271 w1294 w1297 w1306 w1315 w1328 w1336 w1347 w1355] -> _
              tunnel: _ -> [w1268 w1286 w1296 w1305 w1314 w1327 w1335 w1341 w1350 w1358]
              tunnel: w1257 -> [w1267 w1284 _ _ _ _ _ _ _ _]
              tunnel: w1256 -> [w1266 w1280 w1289 _ _ w1323 _ _ _ _]
              tunnel: w1255 -> [w1263 w1282 w1290 _ _ w1321 _ _ _ _]
              tunnel: w1254 -> [w1262 w1281 w1292 _ _ w1320 _ _ _ _]
              tunnel: w1253 -> [w1261 w1276 _ _ _ w1324 _ _ _ _]
              tunnel: w1251 -> [_ w1275 _ _ _ _ _ _ _ _]
              tunnel: w1250 -> [_ w1273 w1287 _ _ w1317 _ _ _ _]
              tunnel: w1249 -> [_ w1272 _ _ _ w1316 _ _ _ _]
              tunnel: w1247 -> [_ _ w1293 _ _ _ _ _ _ _]
              tunnel: w1246 -> [_ _ _ w1304 _ _ _ _ _ _]
              tunnel: w1245 -> [_ _ _ w1302 w1311 _ w1333 w1344 _ _]
              tunnel: w1244 -> [_ _ _ w1301 w1310 _ w1332 _ _ _]
              tunnel: w1243 -> [_ _ _ w1300 w1309 _ w1331 w1342 _ w1353]
              tunnel: w1242 -> [_ _ _ _ w1313 _ _ _ _ _]
              tunnel: w1241 -> [_ _ _ _ _ _ _ w1343 w1351 _]
              tunnel: w1240 -> [_ _ _ _ _ _ _ w1337 _ _]
              tunnel: w1239 -> [_ _ _ _ _ _ _ _ w1345 _]
              tunnel: w1238 -> [_ _ _ _ _ _ _ _ _ w1352]
              frame 0, Default {
                n639 = Index Array(array=w1262, index=w1266) -> (element=w1264:enum16{"Curves", "Values", "Results", "WFM"})
                n640 = Index Array(array=w1263, index=w1266) -> (element=w1265:string)
                n641 = Index Array(array=w1263, index=w1261) -> (element=w1260:string)
                n642 = Index Array(array=w1262, index=w1261) -> (element=w1259:enum16{"Curves", "Values", "Results", "WFM"})
                n643 = Bundle By Name(cluster=w1268, "Work Mode"=w1270, "Binary Operator"=w1267, "Op Type"=w1258, "Curve A"=w1265, "Type A"=w1264, "Curve B"=w1260, "Type B"=w1259) -> (w1269:cluster{})
              }
              frame 1 {
                n644 = Index Array(array=w1281, index=w1280) -> (element=w1278:enum16{"Curves", "Values", "Results", "WFM"})
                n645 = Index Array(array=w1282, index=w1280) -> (element=w1279:string)
                n646 = Index Array(array=w1275, index=w1276) -> (element=w1274:string)
                n647 = Bundle By Name(cluster=w1286, "Work Mode"=w1285, "Binary Operator"=w1284, "Op Type"=w1283, "Curve A"=w1279, "Type A"=w1278, "Curve B"=w1274, "Type B"=enum16{"Curves", "Values", "Results", "WFM"}."Values", "A_single val axis"=w1273, "B_single val axis"=w1272) -> (w1271:cluster{})
              }
              frame 2 {
                n648 = Index Array(array=w1292, index=w1289) -> (element=w1291:enum16{"Curves", "Values", "Results", "WFM"})
                n649 = Index Array(array=w1290, index=w1289) -> (element=w1288:string)
                n650 = Bundle By Name(cluster=w1296, "Unary Operator"=w1293, "Op Type"=w1295, "Type A"=w1291, "Curve A"=w1288, "A_single val axis"=w1287) -> (w1294:cluster{})
              }
              frame 3 {
                n651 = Index Array(array=w1301, index=w1300) -> (element=w1298:string)
                n652 = Index Array(array=w1302, index=w1300) -> (element=w1299:enum16{"Curves", "Values", "Results", "WFM"})
                n653 = Bundle By Name(cluster=w1305, "Statistical Operator"=w1304, "Op Type"=w1303, "Type A"=w1299, "Curve A"=w1298) -> (w1297:cluster{})
              }
              frame 4 {
                n654 = Index Array(array=w1310, index=w1309) -> (element=w1307:string)
                n655 = Index Array(array=w1311, index=w1309) -> (element=w1308:enum16{"Curves", "Values", "Results", "WFM"})
                n656 = Bundle By Name(cluster=w1314, "Width"=w1313, "Op Type"=w1312, "Type A"=w1308, "Curve A"=w1307) -> (w1306:cluster{})
              }
              frame 5 {
                n657 = Index Array(array=w1320, index=w1323) -> (element=w1322:enum16{"Curves", "Values", "Results", "WFM"})
                n658 = Index Array(array=w1320, index=w1324) -> (element=w1318:enum16{"Curves", "Values", "Results", "WFM"})
                n659 = Index Array(array=w1321, index=w1323) -> (element=w1325:string)
                n660 = Index Array(array=w1321, index=w1324) -> (element=w1319:string)
                n661 = Bundle By Name(cluster=w1327, "Op Type"=w1326, "Curve A"=w1325, "Type A"=w1322, "Curve B"=w1319, "Type B"=w1318, "A_single val axis"=w1317, "B_single val axis"=w1316) -> (w1315:cluster{})
              }
              frame 7 {
                n662 = Index Array(array=w1332, index=w1331) -> (element=w1329:string)
                n663 = Index Array(array=w1333, index=w1331) -> (element=w1330:enum16{"Curves", "Values", "Results", "WFM"})
                n664 = Bundle By Name(cluster=w1335, "Op Type"=w1334, "Type A"=w1330, "Curve A"=w1329) -> (w1328:cluster{})
              }
              frame 8, 10 {
                n665 = Index Array(array=w1343, index=w1342) -> (element=w1338:string)
                n666 = Index Array(array=w1344, index=w1342) -> (element=w1339:enum16{"Curves", "Values", "Results", "WFM"})
                n667 = Bundle By Name(cluster=w1341, "Op Type"=w1340, "Type A"=w1339, "Curve A"=w1338, "New Resolution"=w1337) -> (w1336:cluster{})
              }
              frame 9 {
                n668 = Index Array(array=w1351, index=w1345) -> (element=w1348:string)
                n669 = Bundle By Name(cluster=w1350, "Op Type"=w1349, "Type A"=enum16{"Curves", "Values", "Results", "WFM"}."Curves", "Curve A"=w1348) -> (w1347:cluster{})
              }
              frame 11, 12 {
                n670 = Index Array(array=w1352, index=w1353) -> (element=w1356:string)
                n671 = Bundle By Name(cluster=w1358, "Op Type"=w1357, "Type A"=enum16{"Curves", "Values", "Results", "WFM"}."WFM", "Curve A"=w1356) -> (w1355:cluster{})
              }
            }
          }
          frame Enabled {
          }
        }
        n672 = Select(t=u8 2, s=w1235, f=u8 0) -> (s? t:f=w1233:u8)
        n673 = property on="Name" class="Str"("Disabled"=w1233) -> ()  [unwired: 2 in, 2 out]
        n674 = local read "Post Processing"() -> (w1231:T1)
        n675 = Bundle By Name(cluster=w1231, "Use Default Name"=w1235) -> (w1236:T1)
        n676 = case shown="False" w1235 {
          frame False {
            n677 = local read "Name"() -> (w1359:string)
            n678 = property on="Name" class="Str"("Val(Sgnl)"=w1359) -> ()  [unwired: 2 in, 2 out]
          }
          frame True {
            n679 = local write "Name"("") -> ()
          }
        }
        n680 = local write "Post Processing"(w1236) -> ()
      }
      event "binary operation": Value Change {
        n681 = event-data() -> ("NewVal"=w1362:u16)  [unwired: 6 out]
        n682 = local read "Ope_array"() -> (w1367:u16[])
        n683 = local read "Type"() -> (w1365:u16)
        n684 = local read "Post Processing"() -> (w1363:T1)
        n685 = Bundle By Name(cluster=w1363, "Binary Operator"=w1362) -> (w1364:T1)
        n686 = Replace Array Subset(array=w1367, new element=w1362, index=w1365) -> (w1366:u16[])
        n687 = disable-structure shown="Disabled" {
          disable-tunnel: w1365 -> [w1368 _]
          frame Disabled {
            n688 = local read "Work array"() -> (w1369:u16[])
            n689 = Index Array(array=w1369, index=w1368) -> (element=w1370:u16)
            n690 = property on="Work in" class="Slide (strict)"("Val(Sgnl)"=w1370) -> ()  [unwired: 2 in, 2 out]
          }
          frame Enabled {
          }
        }
        n691 = local write "Ope_array"(w1366) -> ()
        n692 = local write "Post Processing"(w1364) -> ()
        n693 = property on="Show Calcu" class="Bool (strict)"("Val(Sgnl)"=TRUE ("Value (Signaling)")) -> ()  [unwired: 2 in, 2 out]
      }
      event "Work in": Value Change {
        n694 = event-data() -> ("OldVal"=w1374:u16, "NewVal"=w1373:u16)  [unwired: 5 out]
        n695 = Not Equal?(x=w1374, y=w1373) -> (x != y?=w1372:bool)
        n696 = local read "Type"() -> (w1371:u16)
        n697 = local read "Work array"() -> (w1379:u16[])
        n698 = case shown="True" w1372 {
          tunnel: w1371 -> [_ w1380]
          frame False {
          }
          frame True {
            n699 = case shown="1" w1380 {
              frame Default {
              }
              frame 0 {
                n700 = local read "Op_A1"() -> (w1382:u16)
                n701 = local read "Op_B"() -> (w1381:u16)
                n702 = property on="Op_A1" class="Ring (strict)"("Val(Sgnl)"=w1382) -> ()  [unwired: 2 in, 2 out]
                n703 = property on="Op_B" class="Ring (strict)"("Val(Sgnl)"=w1381) -> ()  [unwired: 2 in, 2 out]
              }
              frame 1 {
                n704 = local read "Mode_A"() -> (w1386:u16)
                n705 = local read "Op_B"() -> (w1385:u16)
                n706 = Greater Or Equal?(x=w1385, y=u16 1) -> (x >= y?=w1383:bool)
                n707 = property on="Mode_A" class="Slide (strict)"("Val(Sgnl)"=w1386) -> ()  [unwired: 2 in, 2 out]
                n708 = case shown="True" w1383 {
                  frame False {
                    n709 = property on="Op_B" class="Ring (strict)"("Val(Sgnl)"=u16 0 ("Value (Signaling)")) -> ()  [unwired: 2 in, 2 out]
                  }
                  frame True {
                    n710 = local read "Mode_B"() -> (w1388:u16)
                    n711 = property on="Mode_B" class="Slide (strict)"("Val(Sgnl)"=w1388) -> ()  [unwired: 2 in, 2 out]
                  }
                }
              }
            }
          }
        }
        n712 = Replace Array Subset(array=w1379, new element=w1373, index=w1371) -> (w1375:u16[])
        n713 = local read "Use default"() -> (w1376:bool)
        n714 = local write "Work array"(w1375) -> ()
        n715 = local read "Post Processing"() -> (w1378:T1)
        n716 = property on="Use default" class="Bool (strict)"("Val(Sgnl)"=w1376) -> ()  [unwired: 2 in, 2 out]
        n717 = Bundle By Name(cluster=w1378, "Work Mode"=w1373) -> (w1377:T1)
        n718 = local write "Post Processing"(w1377) -> ()
      }
      event "Axis Mode": Value Change {
        n719 = event-data() -> ("NewVal"=w1390:u16)  [unwired: 6 out]
        n720 = local read "Post Processing"() -> (w1391:T1)
        n721 = Bundle By Name(cluster=w1391, "Axis Mode"=w1390) -> (w1389:T1)
        n722 = local write "Post Processing"(w1389) -> ()
      }
      event "Unary Operator": Value Change {
        n723 = event-data() -> ("NewVal"=w1394:u16)  [unwired: 6 out]
        n724 = local read "Post Processing"() -> (w1396:T1)
        n725 = Bundle By Name(cluster=w1396, "Unary Operator"=w1394) -> (w1395:T1)
        n726 = case shown="9" w1394 {
          tunnel: w1392 -> [_ _ w1401 _]
          frame 0..7, Default {
            w1397 = FALSE ("Visible")
            n727 = property on="Smooth Tab" class="TabCtl (strict)"("Visible"=w1397) -> ()  [unwired: 2 in, 2 out]
            n728 = property on="Window Tab" class="TabCtl (strict)"("Visible"=w1397) -> ()  [unwired: 2 in, 2 out]
            n729 = property on="Sampling Tab" class="TabCtl (strict)"("Visible"=w1397) -> ()  [unwired: 2 in, 2 out]
            n730 = property on="Sear_range Tab" class="TabCtl (strict)"("Visible"=w1397) -> ()  [unwired: 2 in, 2 out]
          }
          frame 8 {
            w1399 = FALSE ("Visible")
            n731 = property on="Smooth Tab" class="TabCtl (strict)"("Visible"=TRUE) -> ()  [unwired: 2 in, 2 out]
            n732 = property on="Window Tab" class="TabCtl (strict)"("Visible"=w1399) -> ()  [unwired: 2 in, 2 out]
            n733 = property on="Sampling Tab" class="TabCtl (strict)"("Visible"=w1399) -> ()  [unwired: 2 in, 2 out]
            n734 = property on="Sear_range Tab" class="TabCtl (strict)"("Visible"=w1399) -> ()  [unwired: 2 in, 2 out]
            n735 = property on="Smoo Width" class="DigNum (strict)"("Minimum"=1.0 ("Data Entry Limits:Minimum")) -> ()  [unwired: 2 in, 2 out]
          }
          frame 9 {
            n736 = stacked-sequence {
              tunnel: w1401 -> [w1402 _]
              frame #0 {
                w1412 = TRUE ("Visible")
                w1413 = FALSE ("Visible")
                n737 = property on="Window Tab" class="TabCtl (strict)"("Visible"=w1412) -> ()  [unwired: 2 in, 2 out]
                n738 = property on="Sear_range Tab" class="TabCtl (strict)"("Visible"=w1412) -> ()  [unwired: 2 in, 2 out]
                n739 = property on="Smooth Tab" class="TabCtl (strict)"("Visible"=w1413) -> ()  [unwired: 2 in, 2 out]
                n740 = property on="Sampling Tab" class="TabCtl (strict)"("Visible"=w1413) -> ()  [unwired: 2 in, 2 out]
                n741 = local read "Op_A1"() -> (w1411:u16)
                n742 = local read "Search Items"() -> (w1409:string[])
                n743 = call "CRYGetPost Pro_all data.vi"("No.VI"=w1402) -> ("Type array"=w1410:enum16{"Curves", "Values", "Results", "WFM"}[])  [unwired: 1 in, 13 out]
                n744 = Index Array(array=w1410, index=w1411) -> (element=w1403:enum16{"Curves", "Values", "Results", "WFM"})
                n745 = call "CRYSet Search Ranges.vi"("Search Items"=w1409, "Type"=w1403) -> ("Checks"=w1405:bool[], "Caption"=w1406:string, "Item Names"=w1407:string[], "Symbols"=w1408:i32[])  [unwired: 6 out]
                n746 = case shown="\"WFM\"" w1403 {
                  tunnel: w1405 -> [w1414 w1415]
                  frame "Curves", Default {
                    n747 = local write "Check_Hz"(w1414) -> ()
                  }
                  frame "WFM" {
                    n748 = local write "Check_s"(w1415) -> ()
                  }
                }
                n749 = property on="Search List" class="LstBox (strict)"("Item Symbols"=w1408, "Item Names"=w1407, "Caption.Text"=w1406, "Value"=-1 ("Search List")) -> ()  [unwired: 2 in, 2 out]
              }
              frame #1 {
                n750 = local read "Type"() -> (w1416:u16)
                n751 = local read "All array"() -> (w1418:bool[])
                n752 = Index Array(array=w1418, index=w1416) -> (element=w1417:bool)
                n753 = property on="All" class="Bool (strict)"("Val(Sgnl)"=w1417) -> ()  [unwired: 2 in, 2 out]
              }
            }
          }
          frame 10 {
            w1419 = FALSE ("Visible")
            n754 = property on="Window Tab" class="TabCtl (strict)"("Visible"=w1419) -> ()  [unwired: 2 in, 2 out]
            n755 = property on="Sear_range Tab" class="TabCtl (strict)"("Visible"=w1419) -> ()  [unwired: 2 in, 2 out]
            n756 = property on="Smooth Tab" class="TabCtl (strict)"("Visible"=w1419) -> ()  [unwired: 2 in, 2 out]
            n757 = property on="Sampling Tab" class="TabCtl (strict)"("Visible"=TRUE) -> ()  [unwired: 2 in, 2 out]
          }
        }
        n758 = local write "Post Processing"(w1395) -> ()
        n759 = local read "Use default"() -> (w1393:bool)
        n760 = property on="Use default" class="Bool (strict)"("Val(Sgnl)"=w1393) -> ()  [unwired: 2 in, 2 out]
      }
      event "Op_A2": Value Change {
        n761 = event-data() -> ("OldVal"=w1427:u16, "NewVal"=w1426:u16)  [unwired: 5 out]
        n762 = local read "Type"() -> (w1428:u16)
        n763 = local read "Loading_F"() -> (w1424:bool)
        n764 = Not Equal?(x=w1427, y=w1426) -> (x != y?=w1423:bool)
        n765 = Not(x=w1424) -> (.not. x?=w1425:bool)
        n766 = call "CRYGetPost Pro_all data.vi"("No.VI"=w1421) -> ("Curve array"=w1434:T6, "C&W Type array"=w1430:enum16{"Curves", "Values", "Results", "WFM"}[], "C&W Names"=w1432:string[], "Curve Names"=w1433:string[], "Wave names"=w1435:string[])  [unwired: 1 in, 9 out]
        n767 = And(x=w1423, y=w1425) -> (x .and. y?=w1422:bool)
        n768 = case shown="True" w1422 {
          frame True {
            n769 = local read "Custom unit info"() -> (w1438:T3)
            n770 = Unbundle By Name(w1438) -> ("use custom"=w1437:bool)
            n771 = case shown="False" w1437 {
              frame False {
                n772 = local write "Unit String"("") -> ()
              }
              frame True {
              }
            }
          }
          frame False {
          }
        }
        n773 = Index Array(array=w1430, index=w1426) -> (element=w1429:enum16{"Curves", "Values", "Results", "WFM"})
        n774 = Index Array(array=w1434, index=w1426) -> (element=w1436:T7)
        n775 = case shown="3, 7, Default" w1428 {
          selector: w1428 -> [w1452 _ _ w1500]
          tunnel: w1426 -> [w1450 w1467 w1482 w1496]
          tunnel: w1436 -> [_ _ w1487 _]
          tunnel: w1435 -> [_ _ _ w1498]
          tunnel: w1433 -> [_ _ w1484 _]
          tunnel: w1432 -> [w1448 w1469 _ _]
          tunnel: [w1451 w1468 w1483 w1497] -> w1431
          tunnel: w1429 -> [w1449 w1466 _ _]
          frame 3, 7, Default {
            n776 = Index Array(array=w1448, index=w1450) -> (element=w1451:string)
            n777 = stacked-sequence {
              tunnel: w1449 -> [w1453 _]
              tunnel: w1452 -> [_ w1462]
              frame #0 {
                n778 = local read "Search Items"() -> (w1459:string[])
                n779 = call "CRYSet Search Ranges.vi"("Search Items"=w1459, "Type"=w1453) -> ("Checks"=w1455:bool[], "Caption"=w1456:string, "Item Names"=w1457:string[], "Symbols"=w1458:i32[])  [unwired: 6 out]
                n780 = case shown="\"Curves\", Default" w1453 {
                  tunnel: w1455 -> [w1460 w1461]
                  frame "Curves", Default {
                    n781 = local write "Check_Hz"(w1460) -> ()
                  }
                  frame "WFM" {
                    n782 = local write "Check_s"(w1461) -> ()
                  }
                }
                n783 = property on="Search List" class="LstBox (strict)"("Item Symbols"=w1458, "Item Names"=w1457, "Caption.Text"=w1456, "Value"=-1 ("Search List")) -> ()  [unwired: 2 in, 2 out]
              }
              frame #1 {
                n784 = Equal?(x=w1462, y=u16 3) -> (x = y?=w1463:bool)
                n785 = case shown="False" w1463 {
                  frame False {
                    n786 = local read "Use default"() -> (w1465:bool)
                    n787 = property on="Use default" class="Bool (strict)"("Val(Sgnl)"=w1465) -> ()  [unwired: 2 in, 2 out]
                  }
                  frame True {
                  }
                }
              }
            }
          }
          frame 4 {
            n788 = Index Array(array=w1469, index=w1467) -> (element=w1468:string)
            n789 = case shown="\"Curves\", Default" w1466 {
              tunnel: [u8 0 ("Disabled") u8 2 ("Disabled")] -> w1471
              tunnel: [w1472 w1480] -> w1470
              frame "Curves", Default {
                n790 = local read "Width name"() -> (w1473:string)
                n791 = Search 1D Array(1D array=string[] ["1/1 Octave", "1/3 Octave", "1/6 Octave", "1/12 Octave", "1/24 Octave", "User Defined log", "User Defined lin"] ("Array"), element=w1473) -> (index of element=w1474:i32)  [unwired: 1 out]
                n792 = Equal?(x=-1 ("y"), y=w1474) -> (x = y?=w1477:bool)
                n793 = Select(t=0 ("y"), s=w1477, f=w1474) -> (s? t:f=w1472:i32)
              }
              frame "WFM" {
                w1480 = u16 4 items=["1/1 Octave", "1/3 Octave", "1/6 Octave", "1/12 Octave", "1/24 Octave", "User Defined log", "User Defined lin"] ("Octav Mode")
              }
            }
            n794 = property on="Octav Mode" class="Ring (strict)"("Disabled"=w1471, "Val(Sgnl)"=w1470) -> ()  [unwired: 2 in, 2 out]
          }
          frame 8, 10 {
            n795 = Index Array(array=w1484, index=w1482) -> (element=w1483:string)
            n796 = call "CRYGet Resolution_Steps of Curves.vi"("Curve In"=w1487) -> ("Steps Out"=w1485:i32, "Original Resolution Out"=w1486:string)  [unwired: 9 in]
            n797 = disable-structure shown="Disabled" {
              frame Disabled {
                n798 = local read "New_res str"() -> (w1490:string)
                n799 = property on="New Resolution" class="Ring (strict)"() -> ("Strings []"=w1488:string[])  [unwired: 2 in, 2 out]
                n800 = Search 1D Array(1D array=w1488, element=w1490) -> (index of element=w1494:i32)  [unwired: 1 out]
                n801 = Equal?(x=-1 ("y"), y=w1494) -> (x = y?=w1492:bool)
                n802 = Select(t=0 ("y"), s=w1492, f=w1494) -> (s? t:f=w1489:i32)
                n803 = property on="New Resolution" class="Ring (strict)"("Val(Sgnl)"=w1489) -> ()  [unwired: 2 in, 2 out]
              }
              frame Enabled {
              }
            }
            n804 = local write "Original Res"(w1486) -> ()
            n805 = local write "Steps"(w1485) -> ()
          }
          frame 11, 12 {
            n806 = Index Array(array=w1498, index=w1496) -> (element=w1497:string)
            n807 = Equal?(x=w1500, y=u16 11) -> (x = y?=w1501:bool)
            n808 = case shown="True" w1501 {
              tunnel: w1498 -> [_ w1509]
              tunnel: w1496 -> [_ w1508]
              frame False {
              }
              frame True {
                n809 = Index Array(array=w1509, index=w1508) -> (element=w1506:string)
                n810 = call "CRYGet Curve Library Data.vi"("Type"=enum16{"Curves", "Values", "Results", "WFM"}."WFM", "Data Name"=w1506) -> ("Wave"=w1504:T15)  [unwired: 4 out]
                n811 = Unbundle By Name(w1504) -> ("Waveform.dX"=w1503:dbl)
                n812 = property on="New  Samp Val" class="DigNum (strict)"("Minimum"=1.0 ("Data Entry Limits:Minimum")) -> ()  [unwired: 2 in, 2 out]
                n813 = Reciprocal(x=w1503) -> (1/x=w1502:dbl)
                n814 = local write "Origi Samp Val"(w1502) -> ()
              }
            }
            n815 = local read "Use default"() -> (w1495:bool)
            n816 = property on="Use default" class="Bool (strict)"("Val(Sgnl)"=w1495) -> ()  [unwired: 2 in, 2 out]
          }
        }
        n817 = case shown="11, 12" w1428 {
          tunnel: w1431 -> [w1441 w1444]
          tunnel: w1429 -> [w1440 _]
          frame Default {
            n818 = local read "Post Processing"() -> (w1443:T1)
            n819 = Bundle By Name(cluster=w1443, "Type A"=w1440, "Curve A"=w1441) -> (w1442:T1)
            n820 = local write "Post Processing"(w1442) -> ()
          }
          frame 11, 12 {
            n821 = local read "Post Processing"() -> (w1445:T1)
            n822 = Bundle By Name(cluster=w1445, "Type A"=enum16{"Curves", "Values", "Results", "WFM"}."WFM", "Curve A"=w1444) -> (w1446:T1)
            n823 = local write "Post Processing"(w1446) -> ()
          }
        }
        n824 = local write "A_cur name"(w1431) -> ()
      }
      event "Statistical Operator": Value Change {
        n825 = event-data() -> ("NewVal"=w1510:u16)  [unwired: 6 out]
        n826 = flat-sequence {
          tunnel: w1510 -> [w1513]
          frame #0 {
            n827 = disable-structure shown="Disabled" {
              frame Disabled {
                n828 = property on="Sear_range Tab" class="TabCtl (strict)"("Visible"=TRUE) -> ()  [unwired: 2 in, 2 out]
              }
              frame Enabled {
              }
            }
            n829 = property on="Zwicker_func Tab" class="TabCtl (strict)"("Visible"=FALSE) -> ()  [unwired: 2 in, 2 out]
            n830 = local read "Post Processing"() -> (w1515:T1)
            n831 = Bundle By Name(cluster=w1515, "Statistical Operator"=w1513) -> (w1514:T1)
            n832 = case shown="0..3, Default" w1513 {
              selector: w1513 -> [w1521 _ _ _]
              tunnel: [w1517 _ _ _] -> w1511
              frame 0..3, Default {
                w1523 = FALSE ("Visible")
                n833 = property on="Param Tab" class="TabCtl (strict)"("Visible"=w1523) -> ()  [unwired: 2 in, 2 out]
                n834 = property on="Weight_fun Tab" class="TabCtl (strict)"("Visible"=w1523) -> ()  [unwired: 2 in, 2 out]
                n835 = property on="Sear_range Tab" class="TabCtl (strict)"("Visible"=TRUE) -> ()  [unwired: 2 in, 2 out]
                n836 = Equal To 0?(x=w1521) -> (x = 0?=w1520:bool)
                n837 = Select(t=TRUE ("Visible"), s=w1520, f=FALSE) -> (s? t:f=w1517:bool)
              }
              frame 4, 5, 13, 14 {
                n838 = property on="Weight_fun Tab" class="TabCtl (strict)"("Visible"=FALSE) -> ()  [unwired: 2 in, 2 out]
                n839 = property on="Param Tab" class="TabCtl (strict)"("Visible"=TRUE) -> ()  [unwired: 2 in, 2 out]
                n840 = property on="Sear_range Tab" class="TabCtl (strict)"("Visible"=TRUE) -> ()  [unwired: 2 in, 2 out]
              }
              frame 6..12 {
                n841 = property on="Weight_fun Tab" class="TabCtl (strict)"("Visible"=TRUE) -> ()  [unwired: 2 in, 2 out]
                n842 = property on="Sear_range Tab" class="TabCtl (strict)"("Visible"=TRUE) -> ()  [unwired: 2 in, 2 out]
                n843 = property on="Param Tab" class="TabCtl (strict)"("Visible"=FALSE) -> ()  [unwired: 2 in, 2 out]
                n844 = local read "Use Default Exp"() -> (w1528:bool)
                n845 = property on="Use Default Exp" class="Bool (strict)"("Val(Sgnl)"=w1528) -> ()  [unwired: 2 in, 2 out]
              }
              frame 15 {
                w1532 = FALSE ("Visible")
                n846 = property on="Param Tab" class="TabCtl (strict)"("Visible"=w1532) -> ()  [unwired: 2 in, 2 out]
                n847 = property on="Weight_fun Tab" class="TabCtl (strict)"("Visible"=w1532) -> ()  [unwired: 2 in, 2 out]
                n848 = property on="Sear_range Tab" class="TabCtl (strict)"("Visible"=w1532) -> ()  [unwired: 2 in, 2 out]
                n849 = property on="Zwicker_func Tab" class="TabCtl (strict)"("Visible"=TRUE) -> ()  [unwired: 2 in, 2 out]
              }
            }
            n850 = local write "Post Processing"(w1514) -> ()
            n851 = property on="Work in Statics" class="Slide (strict)"("Visible"=w1511) -> ()  [unwired: 2 in, 2 out]
          }
          frame #1 {
            n852 = local read "Use default"() -> (w1533:bool)
            n853 = property on="Use default" class="Bool (strict)"("Val(Sgnl)"=w1533) -> ()  [unwired: 2 in, 2 out]
          }
        }
      }
      event "Constant": Value Change {
        n854 = event-data() -> ("NewVal"=w1534:dbl)  [unwired: 6 out]
        n855 = local read "Post Processing"() -> (w1538:T1)
        n856 = local read "Work in"() -> (w1536:u16)
        n857 = Bundle By Name(cluster=w1538, "Constant"=w1534) -> (w1537:T1)
        n858 = call "CRYSet Constant to TipStrip.vi"("Work in"=w1536, "Constant"=w1534) -> ("Tip Out"=w1535:string)  [unwired: 9 in]
        n859 = local write "Post Processing"(w1537) -> ()
        n860 = property on="Constant" class="DigNum (strict)"("TipStrip"=w1535) -> ()  [unwired: 2 in, 2 out]
      }
      event "Name": Value Change {
        n861 = event-data() -> ("NewVal"=w1540:string)  [unwired: 6 out]
        n862 = local read "Post Processing"() -> (w1541:T1)
        n863 = Bundle By Name(cluster=w1541, "Result Name"=w1540) -> (w1539:T1)
        n864 = local write "Post Processing"(w1539) -> ()
      }
      event "Smoo Width": Value Change {
        w1543 = 0 ("Data Entry Limits:Minimum")
        n865 = event-data() -> ("NewVal"=w1545:i32)  [unwired: 6 out]
        n866 = Less?(x=w1545, y=w1543) -> (x < y?=w1546:bool)
        n867 = Select(t=w1543, s=w1546, f=w1545) -> (s? t:f=w1544:i32)
        n868 = local read "Post Processing"() -> (w1547:T1)
        n869 = Bundle By Name(cluster=w1547, "Smoothing Width"=w1544) -> (w1542:T1)
        n870 = local write "Post Processing"(w1542) -> ()
      }
      event "Win Mode": Value Change {
        n871 = event-data() -> ("NewVal"=w1550:u16)  [unwired: 6 out]
        n872 = local read "Post Processing"() -> (w1549:T1)
        n873 = Bundle By Name(cluster=w1549, "Window"=w1550) -> (w1548:T1)
        n874 = local write "Post Processing"(w1548) -> ()
      }
      event "Samp Rate": Value Change {
        n875 = event-data() -> ("NewVal"=w1552:dbl)  [unwired: 6 out]
        n876 = local read "Post Processing"() -> (w1553:T1)
        n877 = Bundle By Name(cluster=w1553, "Sampling Rate"=w1552) -> (w1551:T1)
        n878 = local write "Post Processing"(w1551) -> ()
      }
      event "All": Value Change {
        n879 = event-data() -> ("NewVal"=w1564:bool)  [unwired: 6 out]
        n880 = Select(t=u8 2 ("Disabled"), s=w1564, f=u8 0 ("Disabled")) -> (s? t:f=w1561:u8)
        n881 = local read "Post Processing"() -> (w1560:T1)
        n882 = local read "All array"() -> (w1557:bool[])
        n883 = local read "Type"() -> (w1559:u16)
        n884 = Bundle By Name(cluster=w1560, "All points"=w1564) -> (w1554:T1)
        n885 = property on="Search List" class="LstBox (strict)"("Disabled"=w1561, "Value"=-1 ("Search List")) -> ()  [unwired: 2 in, 2 out]
        n886 = To Long Integer(number=w1559) -> (32bit integer=w1558:i32)
        n887 = Replace Array Subset(array=w1557, new element=w1564, index=w1558) -> (w1556:bool[])
        n888 = property on="Edit Range" class="Bool (strict)"("Disabled"=w1561) -> ()  [unwired: 2 in, 2 out]
        n889 = local write "Post Processing"(w1554) -> ()
        n890 = local write "All array"(w1556) -> ()
      }
      event "x_1": Value Change {
        n891 = event-data() -> ("NewVal"=w1571:bool)  [unwired: 6 out]
        n892 = local read "Post Processing"() -> (w1573:T1)
        n893 = local read "Type"() -> (w1568:u16)
        n894 = local read "Show xyz"() -> (w1569:cluster{"x":bool, "y":bool, "z":bool}[])
        n895 = Bundle By Name(cluster=w1573, "x"=w1571) -> (w1565:T1)
        n896 = To Long Integer(number=w1568) -> (32bit integer=w1566:i32)
        n897 = local write "Post Processing"(w1565) -> ()
        n898 = Index Array(array=w1569, index=w1566) -> (element=w1567:cluster{"x":bool, "y":bool, "z":bool})
        n899 = Bundle By Name(cluster=w1567, "x"=w1571) -> (w1570:cluster{"x":bool, "y":bool, "z":bool})
        n900 = Replace Array Subset(array=w1569, new element=w1570, index=w1566) -> (w1572:cluster{"x":bool, "y":bool, "z":bool}[])
        n901 = local write "Show xyz"(w1572) -> ()
      }
      event "y_1": Value Change {
        n902 = event-data() -> ("NewVal"=w1579:bool)  [unwired: 6 out]
        n903 = local read "Type"() -> (w1578:u16)
        n904 = local read "Post Processing"() -> (w1582:T1)
        n905 = local read "Show xyz"() -> (w1577:cluster{"x":bool, "y":bool, "z":bool}[])
        n906 = To Long Integer(number=w1578) -> (32bit integer=w1575:i32)
        n907 = Bundle By Name(cluster=w1582, "y"=w1579) -> (w1574:T1)
        n908 = Index Array(array=w1577, index=w1575) -> (element=w1576:cluster{"x":bool, "y":bool, "z":bool})
        n909 = local write "Post Processing"(w1574) -> ()
        n910 = Bundle By Name(cluster=w1576, "y"=w1579) -> (w1580:cluster{"x":bool, "y":bool, "z":bool})
        n911 = Replace Array Subset(array=w1577, new element=w1580, index=w1575) -> (w1581:cluster{"x":bool, "y":bool, "z":bool}[])
        n912 = local write "Show xyz"(w1581) -> ()
      }
      event "z_1": Value Change {
        n913 = event-data() -> ("NewVal"=w1588:bool)  [unwired: 6 out]
        n914 = local read "Post Processing"() -> (w1591:T1)
        n915 = local read "Type"() -> (w1587:u16)
        n916 = local read "Show xyz"() -> (w1586:cluster{"x":bool, "y":bool, "z":bool}[])
        n917 = Bundle By Name(cluster=w1591, "z"=w1588) -> (w1583:T1)
        n918 = To Long Integer(number=w1587) -> (32bit integer=w1584:i32)
        n919 = local write "Post Processing"(w1583) -> ()
        n920 = Index Array(array=w1586, index=w1584) -> (element=w1585:cluster{"x":bool, "y":bool, "z":bool})
        n921 = Bundle By Name(cluster=w1585, "z"=w1588) -> (w1589:cluster{"x":bool, "y":bool, "z":bool})
        n922 = Replace Array Subset(array=w1586, new element=w1589, index=w1584) -> (w1590:cluster{"x":bool, "y":bool, "z":bool}[])
        n923 = local write "Show xyz"(w1590) -> ()
      }
      event "x_2": Value Change {
        n924 = event-data() -> ("NewVal"=w1597:bool)  [unwired: 6 out]
        n925 = local read "Show xyz"() -> (w1595:cluster{"x":bool, "y":bool, "z":bool}[])
        n926 = local read "Post Processing"() -> (w1600:T1)
        n927 = Index Array(array=w1595, index=6) -> (element=w1593:cluster{"x":bool, "y":bool, "z":bool})
        n928 = Bundle By Name(cluster=w1600, "x"=w1597) -> (w1592:T1)
        n929 = Bundle By Name(cluster=w1593, "x"=w1597) -> (w1598:cluster{"x":bool, "y":bool, "z":bool})
        n930 = local write "Post Processing"(w1592) -> ()
        n931 = Replace Array Subset(array=w1595, new element=w1598, index=6) -> (w1599:cluster{"x":bool, "y":bool, "z":bool}[])
        n932 = local write "Show xyz"(w1599) -> ()
      }
      event "y_2": Value Change {
        n933 = event-data() -> ("NewVal"=w1605:bool)  [unwired: 6 out]
        n934 = local read "Post Processing"() -> (w1609:T1)
        n935 = local read "Show xyz"() -> (w1604:cluster{"x":bool, "y":bool, "z":bool}[])
        n936 = Bundle By Name(cluster=w1609, "y"=w1605) -> (w1601:T1)
        n937 = Index Array(array=w1604, index=6) -> (element=w1602:cluster{"x":bool, "y":bool, "z":bool})
        n938 = local write "Post Processing"(w1601) -> ()
        n939 = Bundle By Name(cluster=w1602, "y"=w1605) -> (w1607:cluster{"x":bool, "y":bool, "z":bool})
        n940 = Replace Array Subset(array=w1604, new element=w1607, index=6) -> (w1608:cluster{"x":bool, "y":bool, "z":bool}[])
        n941 = local write "Show xyz"(w1608) -> ()
      }
      event "Search List": Value Change {
        n942 = event-data() -> ("NewVal"=w1610:i32)  [unwired: 6 out]
        n943 = stacked-sequence {
          seq-local: [w1614 _ _ _] -> [_ _ _ w1645]
          tunnel: w1610 -> [w1611 _ _ _]
          frame #0 {
            n944 = property on="Search List" class="LstBox (strict)"("Top Row"=0) -> ("Caption.Text"=w1617:string, "Item Symbols"=w1612:i32[])  [unwired: 2 in, 2 out]
            n945 = case shown="\"s\"" w1617 {
              tunnel: [w1625 w1626] -> w1618
              tunnel: w1612 -> [_ w1635]
              tunnel: w1611 -> [_ w1633]
              frame "Hz", Default {
                n946 = local read "Check_Hz"() -> (w1625:bool[])
              }
              frame "s" {
                n947 = Search 1D Array(1D array=w1635, element=1) -> (index of element=w1631:i32)  [unwired: 1 in]
                n948 = Equal?(x=w1631, y=w1633) -> (x = y?=w1629:bool)
                n949 = Equal?(x=w1631, y=-1) -> (x = y?=w1628:bool)
                n950 = local read "Check_s"() -> (w1632:bool[])
                n951 = Or(x=w1629, y=w1628) -> (x .or. y?=w1627:bool)
                n952 = case shown="False" w1627 {
                  tunnel: w1632 -> [w1637 w1638]
                  tunnel: [w1636 w1638] -> w1626
                  frame False {
                    n953 = call "CRYOne Check.vi"("In"=w1637) -> ("Out"=w1636:bool[])  [unwired: 4 out]
                  }
                  frame True {
                  }
                }
              }
            }
            n954 = Index Array(array=w1618, index=w1611) -> (element=w1619:bool)
            n955 = Not(x=w1619) -> (.not. x?=w1620:bool)
            n956 = Wait (ms)(milliseconds to wait=u32 50) -> ()  [unwired: 1 out]
            n957 = Replace Array Subset(array=w1618, new element=w1620, index=w1611) -> (w1614:bool[])
            n958 = for {
              tunnel: w1614 -> [w1624] mode=indexing
              tunnel: [w1623] -> w1616 mode=indexing
              n959 = Select(t=0, s=w1624, f=1) -> (s? t:f=w1623:i32)
            }
            n960 = property on="Search List" class="LstBox (strict)"("Item Symbols"=w1616) -> ()  [unwired: 2 in, 2 out]
          }
          frame #1 {
            n961 = local write "Search List"(-1 ("Search List")) -> ()
          }
          frame #2 {
            n962 = Wait (ms)(milliseconds to wait=u32 20) -> ()  [unwired: 1 out]
          }
          frame #3 {
            n963 = property on="Search List" class="LstBox (strict)"() -> ("Item Names"=w1644:string[], "Caption.Text"=w1648:string)  [unwired: 2 in, 2 out]
            n964 = disable-structure shown="Disabled" {
              frame Disabled {
                n965 = call "CRYItems Sort.vi"() -> ()  [unwired: 3 in, 9 out]
              }
              frame Enabled {
              }
            }
            n966 = call "CRYItemCheckSort.vi"("Check_s"=w1645, "In Items"=w1644) -> ("Out Check"=w1642:bool[], "Out Items"=w1643:string[], "Chked Items"=w1641:string[])  [unwired: 6 in, 1 out]
            n967 = for {
              tunnel: w1642 -> [w1653] mode=indexing
              tunnel: [w1652] -> w1647 mode=indexing
              n968 = Select(t=0, s=w1653, f=1) -> (s? t:f=w1652:i32)
            }
            n969 = local read "Post Processing"() -> (w1649:T1)
            n970 = case shown="\"s\"" w1648 {
              tunnel: w1642 -> [w1654 w1655]
              frame "Hz", Default {
                n971 = local write "Check_Hz"(w1654) -> ()
              }
              frame "s" {
                n972 = local write "Check_s"(w1655) -> ()
              }
            }
            n973 = Bundle By Name(cluster=w1649, "Search Items"=w1641) -> (w1646:T1)
            n974 = property on="Search List" class="LstBox (strict)"("Item Names"=w1643, "Item Symbols"=w1647) -> ()  [unwired: 2 in, 2 out]
            n975 = local write "Post Processing"(w1646) -> ()
          }
        }
      }
      event "dB": Value Change {
        n976 = event-data() -> ("NewVal"=w1658:sgl)  [unwired: 6 out]
        n977 = Divide(x=w1658, y=20.0) -> (x/y=w1661:dbl)
        n978 = Power Of 10(x=w1661) -> (10^x=w1662:dbl)
        n979 = Multiply(x=w1662, y=100.0) -> (x*y=w1657:dbl)
        n980 = local read "Post Processing"() -> (w1659:T1)
        n981 = local write "%"(w1657) -> ()
        n982 = Bundle By Name(cluster=w1659, "Para_%"=w1657, "Para_dB"=w1658) -> (w1656:T1)
        n983 = local write "Post Processing"(w1656) -> ()
      }
      event "%": Value Change {
        n984 = event-data() -> ("NewVal"=w1665:sgl)  [unwired: 6 out]
        n985 = Divide(x=w1665, y=sgl 100.0) -> (x/y=w1670:sgl)
        n986 = Logarithm Base 10(1:w1670) -> (0:w1669:sgl)
        n987 = local read "Post Processing"() -> (w1667:T1)
        n988 = Multiply(x=w1669, y=20.0) -> (x*y=w1666:dbl)
        n989 = local write "dB"(w1666) -> ()
        n990 = Bundle By Name(cluster=w1667, "Para_%"=w1665, "Para_dB"=w1666) -> (w1664:T1)
        n991 = local write "Post Processing"(w1664) -> ()
      }
      event "Use Default Exp": Value Change {
        n992 = event-data() -> ("NewVal"=w1675:bool)  [unwired: 6 out]
        n993 = local read "Statistical Operator"() -> (w1677:u16)
        n994 = call "CRYGetPost Pro_all data.vi"("No.VI"=w1672) -> ("Curve Names"=w1674:string[])  [unwired: 1 in, 13 out]
        n995 = case shown="9..11" w1677 {
          tunnel: w1675 -> [w1679 w1684 w1701]
          tunnel: w1674 -> [_ w1683 w1700]
          frame 6..8, Default {
            n996 = case shown="True" w1679 {
              frame False {
                n997 = property on="Exponent" class="DigNum (strict)"("Disabled"=u8 0) -> ()  [unwired: 2 in, 2 out]
              }
              frame True {
                n998 = property on="Exponent" class="DigNum (strict)"("Disabled"=u8 2, "Val(Sgnl)"=sgl 2.2 ("Exponent")) -> ()  [unwired: 2 in, 2 out]
              }
            }
            n999 = property on="Weight Curve_1" class="Ring (strict)"("Visible"=FALSE) -> ()  [unwired: 2 in, 2 out]
          }
          frame 9..11 {
            n1000 = case shown="False" w1684 {
              tunnel: w1683 -> [w1691 _]
              frame False {
                n1001 = local read "Weight_Cur array"() -> (w1694:string[])
                n1002 = property on="Weight Curve_1" class="Ring (strict)"("Visible"=TRUE) -> ()  [unwired: 2 in, 2 out]
                n1003 = local read "Type"() -> (w1692:u16)
                n1004 = local read "Old Exponent"() -> (w1685:sgl)
                n1005 = Index Array(array=w1694, index=w1692) -> (element=w1693:string)
                n1006 = Search 1D Array(1D array=w1691, element=w1693) -> (index of element=w1687:i32)  [unwired: 1 out]
                n1007 = property on="Exponent" class="DigNum (strict)"("Disabled"=u8 0, "Value"=w1685) -> ()  [unwired: 2 in, 2 out]
                n1008 = Equal?(x=-1, y=w1687) -> (x = y?=w1689:bool)
                n1009 = Select(t=0.0, s=w1689, f=w1687) -> (s? t:f=w1686:dbl)
                n1010 = property on="Weight Curve_1" class="Ring (strict)"("Strings []"=w1691, "Value"=w1686) -> ()  [unwired: 2 in, 2 out]
              }
              frame True {
                n1011 = property on="Weight Curve_1" class="Ring (strict)"("Visible"=FALSE) -> ()  [unwired: 2 in, 2 out]
                n1012 = property on="Exponent" class="DigNum (strict)"("Disabled"=u8 2, "Val(Sgnl)"=sgl 0.175 ("Exponent")) -> ()  [unwired: 2 in, 2 out]
              }
            }
          }
          frame 12 {
            n1013 = case shown="False" w1701 {
              tunnel: w1700 -> [w1708 _]
              frame False {
                n1014 = local read "Weight_Cur array"() -> (w1711:string[])
                n1015 = local read "Type"() -> (w1709:u16)
                n1016 = property on="Weight Curve_1" class="Ring (strict)"("Visible"=TRUE) -> ()  [unwired: 2 in, 2 out]
                n1017 = Index Array(array=w1711, index=w1709) -> (element=w1710:string)
                n1018 = local read "Old Exponent"() -> (w1702:sgl)
                n1019 = Search 1D Array(1D array=w1708, element=w1710) -> (index of element=w1704:i32)  [unwired: 1 out]
                n1020 = Equal?(x=-1, y=w1704) -> (x = y?=w1706:bool)
                n1021 = Select(t=0.0, s=w1706, f=w1704) -> (s? t:f=w1703:dbl)
                n1022 = property on="Exponent" class="DigNum (strict)"("Disabled"=u8 0, "Value"=w1702) -> ()  [unwired: 2 in, 2 out]
                n1023 = property on="Weight Curve_1" class="Ring (strict)"("Strings []"=w1708, "Value"=w1703) -> ()  [unwired: 2 in, 2 out]
              }
              frame True {
                n1024 = property on="Weight Curve_1" class="Ring (strict)"("Visible"=FALSE) -> ()  [unwired: 2 in, 2 out]
                n1025 = property on="Exponent" class="DigNum (strict)"("Disabled"=u8 2, "Val(Sgnl)"=sgl 0.225 ("Exponent")) -> ()  [unwired: 2 in, 2 out]
              }
            }
          }
        }
        n1026 = local read "Post Processing"() -> (w1676:T1)
        n1027 = Bundle By Name(cluster=w1676, "Use Default Value"=w1675) -> (w1673:T1)
        n1028 = local write "Post Processing"(w1673) -> ()
      }
      event "Exponent": Value Change {
        n1029 = event-data() -> ("NewVal"=w1717:sgl)  [unwired: 6 out]
        n1030 = local read "Use Default Exp"() -> (w1718:bool)
        n1031 = local read "Post Processing"() -> (w1720:T1)
        n1032 = Bundle By Name(cluster=w1720, "Exponent"=w1717) -> (w1719:T1)
        n1033 = case shown="False" w1718 {
          tunnel: w1717 -> [w1721 _]
          frame False {
            n1034 = local write "Old Exponent"(w1721) -> ()
          }
          frame True {
          }
        }
        n1035 = local write "Post Processing"(w1719) -> ()
      }
      event "Weight Curve_1": Value Change {
        n1036 = event-data() -> ("NewVal"=w1730:u16)  [unwired: 6 out]
        n1037 = local read "Weight_Cur array"() -> (w1728:string[])
        n1038 = call "CRYGetPost Pro_all data.vi"("No.VI"=w1722) -> ("Curve Names"=w1724:string[])  [unwired: 1 in, 13 out]
        n1039 = local read "Type"() -> (w1725:u16)
        n1040 = Index Array(array=w1724, index=w1730) -> (element=w1727:string)
        n1041 = local read "Post Processing"() -> (w1729:T1)
        n1042 = Replace Array Subset(array=w1728, new element=w1727, index=w1725) -> (w1726:string[])
        n1043 = Bundle By Name(cluster=w1729, "Weighting Curve"=w1727) -> (w1723:T1)
        n1044 = local write "Weight_Cur array"(w1726) -> ()
        n1045 = local write "Post Processing"(w1723) -> ()
      }
      event "Octav Mode": Value Change {
        n1046 = event-data() -> ("OldVal"=w1736:u16, "NewVal"=w1734:u16)  [unwired: 5 out]
        n1047 = local read "Post Processing"() -> (w1739:T1)
        n1048 = Not Equal?(x=w1736, y=w1734) -> (x != y?=w1735:bool)
        n1049 = Bundle By Name(cluster=w1739, "Width"=w1734) -> (w1738:T1)
        n1050 = case shown="True" w1735 {
          tunnel: w1734 -> [_ w1743]
          frame False {
          }
          frame True {
            n1051 = Index Array(array=string[] ["1/1 Octave", "1/3 Octave", "1/6 Octave", "1/12 Octave", "1/24 Octave", "User Defined log", "User Defined lin"] ("Array"), index=w1743) -> (element=w1745:string)
            n1052 = local write "Width name"(w1745) -> ()
          }
        }
        n1053 = local write "Post Processing"(w1738) -> ()
        n1054 = call "CRYGet Error Message.vi"("Kind"="Post Processing Sub") -> ("Unicode Message Sub"=w1732:string[])  [unwired: 5 in, 5 out]
        n1055 = for {
          tunnel: w1732 -> [w1742] mode=indexing
          tunnel: [w1741] -> w1731 mode=indexing
          n1056 = call "CRYConvert Unicode to ASCII.vi"("Unicode"=w1742) -> ("ASCII"=w1741:string)  [unwired: 4 in]
        }
        n1057 = case shown="5" w1734 {
          tunnel: w1731 -> [_ w1749 w1761]
          frame 0..4, Default {
            n1058 = property on="Hz_Oct_1" class="DigNum (strict)"("Visible"=FALSE) -> ()  [unwired: 2 in, 2 out]
          }
          frame 5 {
            n1059 = local read "Hz_oct array"() -> (w1754:dbl[])
            n1060 = local read "Type"() -> (w1752:u16)
            n1061 = Index Array(array=w1749, index=2) -> (element=w1747:string)
            n1062 = Index Array(array=w1754, index=w1752) -> (element=w1753:dbl)
            n1063 = property on="Hz_Oct_1" class="DigNum (strict)"("Visible"=TRUE, "Caption.Text"=w1747, "Value"=w1753, "Minimum"=1.0 ("Data Entry Limits:Minimum")) -> ()  [unwired: 2 in, 2 out]
          }
          frame 6 {
            n1064 = property on="Octav Mode" class="Ring (strict)"() -> ("DisabledEnum"=w1767:T11)  [unwired: 2 in, 2 out]
            n1065 = Equal To 0?(x=w1767) -> (x = 0?=w1765:bool)
            n1066 = Select(t=1.0, s=w1765, f=0.0) -> (s? t:f=w1762:dbl)
            n1067 = local read "Hz_oct array"() -> (w1769:dbl[])
            n1068 = Index Array(array=w1761, index #1=3 ("index"), index #2=4 ("index")) -> (element #1=w1758:string, element #2=w1757:string)
            n1069 = local read "Type"() -> (w1756:u16)
            n1070 = Index Array(array=w1769, index=w1756) -> (element=w1768:dbl)
            n1071 = Select(t=w1758, s=w1765, f=w1757) -> (s? t:f=w1755:string)
            n1072 = property on="Hz_Oct_1" class="DigNum (strict)"("Visible"=TRUE, "Caption.Text"=w1755, "Value"=w1768, "Minimum"=w1762) -> ()  [unwired: 2 in, 2 out]
          }
        }
        n1073 = local read "Use default"() -> (w1733:bool)
        n1074 = property on="Use default" class="Bool (strict)"("Val(Sgnl)"=w1733) -> ()  [unwired: 2 in, 2 out]
        n1075 = local read "Weight Mode"() -> (w1737:u16)
        n1076 = property on="Weight Mode" class="Ring (strict)"("Value"=w1737) -> ()  [unwired: 2 in, 2 out]
      }
      event "Hz_Oct_1": Value Change {
        n1077 = event-data() -> ("NewVal"=w1772:dbl)  [unwired: 6 out]
        n1078 = property on="Octav Mode" class="Ring (strict)"() -> ("DisabledEnum"=w1775:T11)  [unwired: 2 in, 2 out]
        n1079 = case shown="\"Disabled and Grayed Out\"" w1775 {
          tunnel: [1 ("y") 0 ("y")] -> w1773
          frame "Enabled", Default {
          }
          frame "Disabled and Grayed Out" {
          }
        }
        n1080 = Less?(x=w1772, y=w1773) -> (x < y?=w1774:bool)
        n1081 = Select(t=w1773, s=w1774, f=w1772) -> (s? t:f=w1771:dbl)
        n1082 = local read "Post Processing"() -> (w1779:T1)
        n1083 = local read "Hz_oct array"() -> (w1778:dbl[])
        n1084 = local read "Type"() -> (w1776:u16)
        n1085 = Bundle By Name(cluster=w1779, "Hz"=w1771) -> (w1770:T1)
        n1086 = local write "Post Processing"(w1770) -> ()
        n1087 = Replace Array Subset(array=w1778, new element=w1771, index=w1776) -> (w1777:dbl[])
        n1088 = local write "Hz_oct array"(w1777) -> ()
      }
      event "Weight Mode": Value Change {
        n1089 = event-data() -> ("NewVal"=w1783:u16)  [unwired: 6 out]
        n1090 = local read "Post Processing"() -> (w1784:T1)
        n1091 = Bundle By Name(cluster=w1784, "Weighting win"=w1783) -> (w1782:T1)
        n1092 = local write "Post Processing"(w1782) -> ()
      }
      event "Search Mode": Value Change {
        n1093 = event-data() -> ("NewVal"=w1786:u16)  [unwired: 6 out]
        n1094 = local read "Post Processing"() -> (w1787:T1)
        n1095 = Bundle By Name(cluster=w1787, "Search Mode"=w1786) -> (w1785:T1)
        n1096 = local write "Post Processing"(w1785) -> ()
      }
      event "New Resolution": Value Change {
        n1097 = event-data() -> ("NewVal"=w1791:u16)  [unwired: 6 out]
        n1098 = local read "Type"() -> (w1795:u16)
        n1099 = call "CRYGet Error Message.vi"("Kind"="Post Processing Sub") -> ("Unicode Message Sub"=w1789:string[])  [unwired: 5 in, 5 out]
        n1100 = for {
          tunnel: w1789 -> [w1799] mode=indexing
          tunnel: [w1798] -> w1788 mode=indexing
          n1101 = call "CRYConvert Unicode to ASCII.vi"("Unicode"=w1799) -> ("ASCII"=w1798:string)  [unwired: 4 in]
        }
        n1102 = case shown="8, Default" w1795 {
          tunnel: w1791 -> [_ w1803]
          tunnel: w1788 -> [_ w1802]
          frame 10 {
            n1103 = property on="Frequencies" class="Slide (strict)"("Visible"=FALSE) -> ()  [unwired: 2 in, 2 out]
            n1104 = property on="Hz_Oct_2" class="DigNum (strict)"("Visible"=FALSE) -> ()  [unwired: 2 in, 2 out]
          }
          frame 8, Default {
            n1105 = case shown="0, 1, Default" w1803 {
              tunnel: w1802 -> [_ _ w1810 w1819]
              frame 0, 1, Default {
                n1106 = property on="Frequencies" class="Slide (strict)"("Visible"=FALSE) -> ()  [unwired: 2 in, 2 out]
                n1107 = property on="Hz_Oct_2" class="DigNum (strict)"("Visible"=FALSE) -> ()  [unwired: 2 in, 2 out]
              }
              frame 2..4 {
                n1108 = property on="Frequencies" class="Slide (strict)"("Visible"=TRUE) -> ()  [unwired: 2 in, 2 out]
                n1109 = property on="Hz_Oct_2" class="DigNum (strict)"("Visible"=FALSE) -> ()  [unwired: 2 in, 2 out]
              }
              frame 5 {
                n1110 = local read "Hz_oct array"() -> (w1815:dbl[])
                n1111 = Index Array(array=w1810, index=2) -> (element=w1808:string)
                n1112 = local read "Type"() -> (w1813:u16)
                n1113 = property on="Frequencies" class="Slide (strict)"("Visible"=FALSE) -> ()  [unwired: 2 in, 2 out]
                n1114 = Index Array(array=w1815, index=w1813) -> (element=w1814:dbl)
                n1115 = property on="Hz_Oct_2" class="DigNum (strict)"("Visible"=TRUE, "Caption.Text"=w1808, "Value"=w1814, "Minimum"=1.0 ("Data Entry Limits:Minimum")) -> ()  [unwired: 2 in, 2 out]
              }
              frame 6 {
                n1116 = local read "Hz_oct array"() -> (w1824:dbl[])
                n1117 = local read "Type"() -> (w1822:u16)
                n1118 = Index Array(array=w1819, index=3) -> (element=w1817:string)
                n1119 = property on="Frequencies" class="Slide (strict)"("Visible"=FALSE) -> ()  [unwired: 2 in, 2 out]
                n1120 = Index Array(array=w1824, index=w1822) -> (element=w1823:dbl)
                n1121 = property on="Hz_Oct_2" class="DigNum (strict)"("Visible"=TRUE, "Caption.Text"=w1817, "Value"=w1823, "Minimum"=1.0 ("Data Entry Limits:Minimum")) -> ()  [unwired: 2 in, 2 out]
              }
            }
          }
        }
        n1122 = case shown="8, Default" w1795 {
          tunnel: [string[] ["1/1 Octave", "1/3 Octave", "1/6 Octave", "1/12 Octave", "1/24 Octave", "User Defined log", "User Defined lin"] ("Array") string[] ["1/1 Octave", "1/3 Octave", "1/6 Octave", "1/12 Octave", "1/24 Octave"] ("Array")] -> w1797
          frame 8, Default {
          }
          frame 10 {
          }
        }
        n1123 = Index Array(array=w1797, index=w1791) -> (element=w1796:string)
        n1124 = local write "New_res str"(w1796) -> ()
        n1125 = local read "Post Processing"() -> (w1793:T1)
        n1126 = Bundle By Name(cluster=w1793, "New Resolution"=w1791) -> (w1792:T1)
        n1127 = local read "Use default"() -> (w1790:bool)
        n1128 = local write "Post Processing"(w1792) -> ()
        n1129 = property on="Use default" class="Bool (strict)"("Val(Sgnl)"=w1790) -> ()  [unwired: 2 in, 2 out]
      }
      event "Hz_Oct_2": Value Change {
        w1831 = 1 ("y")
        n1130 = event-data() -> ("NewVal"=w1830:u32)  [unwired: 6 out]
        n1131 = Less?(x=w1830, y=w1831) -> (x < y?=w1832:bool)
        n1132 = local read "Post Processing"() -> (w1836:T1)
        n1133 = Select(t=w1831, s=w1832, f=w1830) -> (s? t:f=w1829:u32)
        n1134 = local read "Hz_oct array"() -> (w1835:dbl[])
        n1135 = Bundle By Name(cluster=w1836, "Hz"=w1829) -> (w1828:T1)
        n1136 = local read "Type"() -> (w1833:u16)
        n1137 = local write "Post Processing"(w1828) -> ()
        n1138 = Replace Array Subset(array=w1835, new element=w1829, index=w1833) -> (w1834:dbl[])
        n1139 = local write "Hz_oct array"(w1834) -> ()
      }
      event "Frequencies": Value Change {
        n1140 = event-data() -> ("NewVal"=w1838:u16)  [unwired: 6 out]
        n1141 = local read "Post Processing"() -> (w1839:T1)
        n1142 = Bundle By Name(cluster=w1839, "Freq Mode"=w1838) -> (w1837:T1)
        n1143 = local write "Post Processing"(w1837) -> ()
      }
      event "Ref_Curve": Value Change {
        n1144 = event-data() -> ("NewVal"=w1847:u16)  [unwired: 6 out]
        n1145 = call "CRYGetPost Pro_all data.vi"("No.VI"=w1840) -> ("Curve Names"=w1846:string[])  [unwired: 1 in, 13 out]
        n1146 = Index Array(array=w1846, index=w1847) -> (element=w1842:string)
        n1147 = local write "A_cur name"(w1842) -> ()
        n1148 = local read "Post Processing"() -> (w1845:T1)
        n1149 = Bundle By Name(cluster=w1845, "Curve A"=w1842, "Type A"=enum16{"Curves", "Values", "Results", "WFM"}."Curves") -> (w1844:T1)
        n1150 = local write "Post Processing"(w1844) -> ()
        n1151 = local read "Use default"() -> (w1841:bool)
        n1152 = property on="Use default" class="Bool (strict)"("Val(Sgnl)"=w1841) -> ()  [unwired: 2 in, 2 out]
      }
      event "Curve List": Value Change {
        n1153 = event-data() -> ("NewVal"=w1853:i32[])  [unwired: 6 out]
        n1154 = call "CRYGetPost Pro_all data.vi"("No.VI"=w1848) -> ("Curve Names"=w1850:string[])  [unwired: 1 in, 13 out]
        n1155 = for {
          tunnel: w1853 -> [w1856] mode=indexing
          tunnel: w1850 -> [w1855]
          tunnel: [w1854] -> w1851 mode=indexing
          n1156 = Index Array(array=w1855, index=w1856) -> (element=w1854:string)
        }
        n1157 = local read "Post Processing"() -> (w1852:T1)
        n1158 = Bundle By Name(cluster=w1852, "Curve Group"=w1851) -> (w1849:T1)
        n1159 = local write "Post Processing"(w1849) -> ()
      }
      event "Direct_weight": Value Change {
        n1160 = event-data() -> ("NewVal"=w1863:bool)  [unwired: 6 out]
        n1161 = local read "Post Processing"() -> (w1858:T1)
        n1162 = Select(t=u8 0 ("Disabled"), s=w1863, f=u8 2) -> (s? t:f=w1860:u8)
        n1163 = Bundle By Name(cluster=w1858, "Direct Weighting"=w1863) -> (w1857:T1)
        n1164 = local read "Auto Inc"() -> (w1862:bool)
        n1165 = property on="Weight Curve_2" class="Ring (strict)"("Disabled"=w1860) -> ()  [unwired: 2 in, 2 out]
        n1166 = property on="Auto Inc" class="Bool (strict)"("Val(Sgnl)"=w1862) -> ()  [unwired: 2 in, 2 out]
        n1167 = local write "Post Processing"(w1857) -> ()
      }
      event "Weight Curve_2": Value Change {
        n1168 = event-data() -> ("NewVal"=w1868:u16)  [unwired: 6 out]
        n1169 = local read "Weight_Cur array"() -> (w1871:string[])
        n1170 = call "CRYGetPost Pro_all data.vi"("No.VI"=w1864) -> ("Curve Names"=w1866:string[])  [unwired: 1 in, 13 out]
        n1171 = local read "Type"() -> (w1867:u16)
        n1172 = Index Array(array=w1866, index=w1868) -> (element=w1870:string)
        n1173 = local read "Post Processing"() -> (w1872:T1)
        n1174 = Bundle By Name(cluster=w1872, "Weighting Curve"=w1870) -> (w1865:T1)
        n1175 = Replace Array Subset(array=w1871, new element=w1870, index=w1867) -> (w1869:string[])
        n1176 = local write "Weight_Cur array"(w1869) -> ()
        n1177 = local write "Post Processing"(w1865) -> ()
      }
      event "Auto Inc": Value Change {
        n1178 = event-data() -> ("NewVal"=w1875:bool)  [unwired: 6 out]
        n1179 = case shown="False" w1875 {
          frame False {
            n1180 = property on="Inc(deg.)" class="DigNum (strict)"("Disabled"=u8 0) -> ()  [unwired: 2 in, 2 out]
            n1181 = property on="Total Rotation" class="DigNum (strict)"("Disabled"=u8 2) -> ()  [unwired: 2 in, 2 out]
          }
          frame True {
            n1182 = property on="Inc(deg.)" class="DigNum (strict)"("Disabled"=u8 2) -> ()  [unwired: 2 in, 2 out]
            n1183 = property on="Total Rotation" class="DigNum (strict)"("Disabled"=u8 0) -> ()  [unwired: 2 in, 2 out]
          }
        }
        n1184 = local read "Post Processing"() -> (w1874:T1)
        n1185 = Bundle By Name(cluster=w1874, "Auto Inc"=w1875) -> (w1873:T1)
        n1186 = local write "Post Processing"(w1873) -> ()
      }
      event "Inc(deg.)": Value Change {
        n1187 = event-data() -> ("NewVal"=w1881:i32)  [unwired: 6 out]
        n1188 = local read "Post Processing"() -> (w1882:T1)
        n1189 = Bundle By Name(cluster=w1882, "Inc(deg)"=w1881) -> (w1880:T1)
        n1190 = local write "Post Processing"(w1880) -> ()
      }
      event "Total Rotation": Value Change {
        n1191 = event-data() -> ("NewVal"=w1884:i32)  [unwired: 6 out]
        n1192 = local read "Post Processing"() -> (w1885:T1)
        n1193 = Bundle By Name(cluster=w1885, "Total Rotation"=w1884) -> (w1883:T1)
        n1194 = local write "Post Processing"(w1883) -> ()
      }
      event "New  Samp Val": Value Change {
        w1889 = 1.0 ("y")
        n1195 = event-data() -> ("NewVal"=w1888:dbl)  [unwired: 6 out]
        n1196 = Less?(x=w1888, y=w1889) -> (x < y?=w1890:bool)
        n1197 = Select(t=w1889, s=w1890, f=w1888) -> (s? t:f=w1887:dbl)
        n1198 = local read "Post Processing"() -> (w1891:T1)
        n1199 = Bundle By Name(cluster=w1891, "New Sampling Rate"=w1887) -> (w1886:T1)
        n1200 = local write "Post Processing"(w1886) -> ()
      }
      event "Ref Freq Mode": Value Change {
        n1201 = event-data() -> ("NewVal"=w1894:u16)  [unwired: 6 out]
        n1202 = case shown="1" w1894 {
          frame 0, Default {
            n1203 = local read "Ref Wave"() -> (w1895:u16)
            n1204 = property on="Ref Frequency" class="DigNum (strict)"("Disabled"=u8 2) -> ()  [unwired: 2 in, 2 out]
            n1205 = property on="Ref Wave" class="Ring (strict)"("Disabled"=u8 0, "Val(Sgnl)"=w1895) -> ()  [unwired: 2 in, 2 out]
          }
          frame 1 {
            n1206 = local read "Ref Frequency"() -> (w1898:dbl)
            n1207 = property on="Ref Wave" class="Ring (strict)"("Disabled"=u8 2) -> ()  [unwired: 2 in, 2 out]
            n1208 = property on="Ref Frequency" class="DigNum (strict)"("Disabled"=u8 0, "Val(Sgnl)"=w1898) -> ()  [unwired: 2 in, 2 out]
          }
        }
        n1209 = local read "Post Processing"() -> (w1893:T1)
        n1210 = Bundle By Name(cluster=w1893, "Ref Freq Mode"=w1894) -> (w1892:T1)
        n1211 = local write "Post Processing"(w1892) -> ()
      }
      event "Ref Wave": Value Change {
        n1212 = event-data() -> ("NewVal"=w1905:u16)  [unwired: 6 out]
        n1213 = local read "Ref Freq Mode"() -> (w1904:u16)
        n1214 = call "CRYGetPost Pro_all data.vi"("No.VI"=w1901) -> ("Wave names"=w1902:string[])  [unwired: 1 in, 13 out]
        n1215 = Equal To 0?(x=w1904) -> (x = 0?=w1903:bool)
        n1216 = case shown="True" w1903 {
          tunnel: w1905 -> [_ w1910]
          tunnel: w1902 -> [_ w1907]
          frame False {
          }
          frame True {
            n1217 = Index Array(array=w1907, index=w1910) -> (element=w1908:string)
            n1218 = local read "Post Processing"() -> (w1909:T1)
            n1219 = Bundle By Name(cluster=w1909, "Ref Waveform"=w1908) -> (w1906:T1)
            n1220 = local write "Post Processing"(w1906) -> ()
          }
        }
      }
      event "Ref Frequency": Value Change {
        n1221 = event-data() -> ("NewVal"=w1912:dbl)  [unwired: 6 out]
        n1222 = local read "Post Processing"() -> (w1913:T1)
        n1223 = Bundle By Name(cluster=w1913, "Ref Freq"=w1912) -> (w1911:T1)
        n1224 = local write "Post Processing"(w1911) -> ()
      }
      event "Custom unit info": Value Change {
        n1225 = event-data() -> ("NewVal"=w1915:T3)  [unwired: 6 out]
        n1226 = local read "Post Processing"() -> (w1916:T1)
        n1227 = Bundle By Name(cluster=w1916, "Custom unit info"=w1915) -> (w1914:T1)
        n1228 = local write "Post Processing"(w1914) -> ()
      }
      event "Unit String": Value Change {
        n1229 = event-data() -> ("NewVal"=w1918:string)  [unwired: 6 out]
        n1230 = local read "Post Processing"() -> (w1919:T1)
        n1231 = Bundle By Name(cluster=w1919, "Unit"=w1918) -> (w1917:T1)
        n1232 = local write "Post Processing"(w1917) -> ()
      }
      event "User Equation String": Value Change {
        n1233 = event-data() -> ("NewVal"=w1921:string)  [unwired: 6 out]
        n1234 = call "CRYUnflatten User Equation Cluster.vi"("Flatten user equation cluster string"=w1921) -> ("User Equation Cluster"=w1922:T2)  [unwired: 8 in, 2 out]
        n1235 = local read "Post Processing"() -> (w1923:T1)
        n1236 = Bundle By Name(cluster=w1923, "user equation cluster"=w1922) -> (w1920:T1)
        n1237 = local write "Post Processing"(w1920) -> ()
      }
      event "Equ_List": Value Change {
        n1238 = event-data() -> ("NewVal"=w1924:string)  [unwired: 6 out]
        n1239 = stacked-sequence {
          tunnel: w1924 -> [w1940 _]
          frame #0 {
            n1240 = local read "Post Processing"() -> (w1939:T1)
            n1241 = call "CRYGet Formula & Result Variable.vi"("String"=w1940) -> ("Formula Out"=w1935:string[], "Result Variable"=w1932:string[], "Out string"=w1936:string)  [unwired: 8 in]
            n1242 = Unbundle By Name(w1939) -> ("user equation cluster"=w1929:T2)
            n1243 = Unbundle By Name(w1929) -> ("Desired Result Variables"=w1930:string[])
            n1244 = Array Size(array=w1935) -> (size(s)=w1931:i32)
            n1245 = for {
              tunnel: w1932 -> [w1945] mode=indexing
              tunnel: w1930 -> [w1949]
              tunnel: w1929 -> [w1947]
              tunnel: [w1944] -> w1928 mode=indexing
              tunnel: [w1943] -> w1927 mode=indexing
              tunnel: [w1942] -> w1926 mode=indexing
              tunnel: [w1941] -> w1925 mode=indexing
              n1246 = Search 1D Array(1D array=w1949, element=w1945) -> (index of element=w1946:i32)  [unwired: 1 in]
              n1247 = Less Than 0?(x=w1946) -> (x < 0?=w1948:bool)
              n1248 = case shown="False" w1948 {
                tunnel: w1946 -> [w1954 _]
                tunnel: w1947 -> [w1959 _]
                tunnel: w1945 -> [_ w1961]
                tunnel: [w1953 w1961] -> w1944
                tunnel: [w1952 w1961] -> w1943
                tunnel: [w1951 "No data"] -> w1942
                tunnel: [w1950 w1962] -> w1941
                frame False {
                  n1249 = Unbundle By Name(w1959) -> ("Desired Result Names"=w1958:string[], "Desired Result Variables"=w1957:string[], "Result Values"=w1956:string[], "Custom unit results array"=w1955:T16)
                  n1250 = Index Array(array=w1958, index=w1954) -> (element=w1953:string)
                  n1251 = Index Array(array=w1957, index=w1954) -> (element=w1952:string)
                  n1252 = Index Array(array=w1956, index=w1954) -> (element=w1951:string)
                  n1253 = Index Array(array=w1955, index=w1954) -> (element=w1950:T3)
                }
                frame True {
                  n1254 = Bundle By Name(cluster=T3 {"use custom"=FALSE, "lin/log"=0, "unit"="", "dB ref"=0.0, "common dB"=0} ("Custom unit info"), "lin/log"=u16 0, "unit"="", "dB ref"=1.0) -> (w1962:T3)
                }
              }
            }
            n1255 = Initialize Array(u16 1 ("element"), w1931) -> (w1933:u16[])
            n1256 = Bundle By Name(cluster=w1929, "equation"=w1936, "Desired Result Names"=w1928, "Desired Result Variables"=w1927, "Result Values"=w1926, "Custom unit results array"=w1925, "Results axis"=w1933, "# Desired result curves"=w1931) -> (w1937:T2)
            n1257 = local write "#Desired Results"(w1931) -> ()
            n1258 = call "CRYFlatten User Equation Cluster.vi"("user equation cluster"=w1937) -> ("Flatten String"=w1938:string)  [unwired: 10 in]
            n1259 = property on="User Equation String" class="Str"("Val(Sgnl)"=w1938) -> ()  [unwired: 2 in, 2 out]
          }
          frame #1 {
            n1260 = global read "CRYPost Processing Global.vi" "User Equation VI Ref"() -> (w1967:refnum<vi>)
            n1261 = call "CRYGet Boolean Reference.vi"("Label Name"=" Res_Table Change", "VI Refnum"=w1967) -> ("Boolean Ref"=w1969:refnum<vi>)  [unwired: 7 in, 2 out]
            n1262 = property class="Bool"(reference=w1969, "Val(Sgnl)"=TRUE) -> ()  [unwired: 1 in, 2 out]
          }
        }
      }
      event "Help": Value Change {
        n1263 = event-data() -> ("NewVal"=w1972:string)  [unwired: 6 out]
        n1264 = local read "Post Processing"() -> (w1973:T1)
        n1265 = Bundle By Name(cluster=w1973, "Help"=w1972) -> (w1971:T1)
        n1266 = local write "Post Processing"(w1971) -> ()
      }
      event "Main Tab": Value Change {
        n1267 = event-data() -> ("NewVal"=w1975:enum32{"Setting", "Help"})  [unwired: 6 out]
        n1268 = local read "Post Processing"() -> (w1976:T1)
        n1269 = Bundle By Name(cluster=w1976, "Tab Value"=w1975) -> (w1974:T1)
        n1270 = local write "Post Processing"(w1974) -> ()
      }
      event "StateOut": Value Change {
        n1271 = event-data() -> ("NewVal"=w1978:bool)  [unwired: 6 out]
        n1272 = case shown="True" w1978 {
          tunnel: w1977 -> [w1983 w1986]
          frame False {
            n1273 = property class="VI"(reference=w1983) -> (reference out=w1980:refnum<vi>, "FP.State"=w1982:T10)  [unwired: 1 in, 1 out]
            n1274 = Equal?(x=w1982, y=T10."Standard" ("Front Panel Window:State")) -> (x = y?=w1979:bool)
            n1275 = case shown="True" w1979 {
              tunnel: w1980 -> [_ w1985]
              frame False {
              }
              frame True {
                n1276 = property class="VI"(reference=w1985, "FP.State"=T10."Hidden" ("Front Panel Window:State")) -> ()  [unwired: 1 in, 2 out]
              }
            }
          }
          frame True {
            n1277 = property class="VI"(reference=w1986) -> (reference out=w1988:refnum<vi>, "FP.State"=w1990:T10)  [unwired: 1 in, 1 out]
            n1278 = Equal?(x=w1990, y=T10."Hidden" ("Front Panel Window:State")) -> (x = y?=w1987:bool)
            n1279 = case shown="True" w1987 {
              tunnel: w1988 -> [_ w1992]
              frame False {
              }
              frame True {
                n1280 = property class="VI"(reference=w1992, "FP.State"=T10."Standard" ("Front Panel Window:State")) -> ()  [unwired: 1 in, 2 out]
              }
            }
          }
        }
      }
      event "Loading_F": Value Change {
        n1281 = event-data() -> ("NewVal"=w1994:bool)  [unwired: 6 out]
        n1282 = case shown="True" w1994 {
          tunnel: w1993 -> [_ w1995]
          frame False {
          }
          frame True {
            n1283 = local read "Custom unit info"() -> (w2000:T3)
            n1284 = Unbundle By Name(w2000) -> ("lin/log"=w1998:u16, "use custom"=w1999:bool, "unit"=w1997:string)
            n1285 = case shown="False" w1999 {
              tunnel: w1998 -> [w2003 _]
              tunnel: w1997 -> [w2002 _]
              tunnel: [w2001 w2007] -> w1996
              tunnel: w1995 -> [_ w2006]
              frame True {
                n1286 = Equal To 0?(x=w2003) -> (x = 0?=w2005:bool)
                n1287 = Select(t="dB" ("Y unit"), s=w2005, f=w2002) -> (s? t:f=w2001:string)
              }
              frame False {
                n1288 = local read "A_cur name"() -> (w2009:string)
                n1289 = call "CRYGetPost Pro_all data.vi"("No.VI"=w2006) -> ("Curve array"=w2014:T6, "Value array"=w2013:T6, "All Names"=w2021:string[], "Value Names"=w2011:string[], "Waveform Array"=w2008:T14, "Type array"=w2017:enum16{"Curves", "Values", "Results", "WFM"}[], "Wave names"=w2010:string[])  [unwired: 1 in, 7 out]
                n1290 = Search 1D Array(1D array=w2021, element=w2009) -> (index of element=w2012:i32)  [unwired: 1 out]
                n1291 = Equal?(x=-1 ("y"), y=w2012) -> (x = y?=w2018:bool)
                n1292 = Select(t=0 ("y"), s=w2018, f=w2012) -> (s? t:f=w2016:i32)
                n1293 = Index Array(array=w2017, index=w2016) -> (element=w2015:enum16{"Curves", "Values", "Results", "WFM"})
                n1294 = case shown="\"WFM\"" w2015 {
                  tunnel: [w2023 w2033 w2040] -> w2007
                  tunnel: w2014 -> [w2028 _ _]
                  tunnel: w2013 -> [_ w2038 _]
                  tunnel: w2012 -> [w2022 _ _]
                  tunnel: w2011 -> [_ w2032 _]
                  tunnel: w2009 -> [_ w2031 w2047]
                  tunnel: w2008 -> [_ _ w2049]
                  tunnel: w2010 -> [_ _ w2048]
                  frame "Curves", Default {
                    n1295 = Index Array(array=w2028, index=w2022) -> (element=w2029:T7)
                    n1296 = Unbundle By Name(w2029) -> ("Y data"=w2027:u16, "Y unit"=w2024:string)
                    n1297 = Equal To 0?(x=w2027) -> (x = 0?=w2026:bool)
                    n1298 = Select(t="dB" ("Y unit"), s=w2026, f=w2024) -> (s? t:f=w2023:string)
                  }
                  frame "Values" {
                    n1299 = Search 1D Array(1D array=w2032, element=w2031) -> (index of element=w2030:i32)  [unwired: 1 out]
                    n1300 = Index Array(array=w2038, index=w2030) -> (element=w2039:T7)
                    n1301 = Unbundle By Name(w2039) -> ("Y data"=w2035:u16, "Y unit"=w2034:string)
                    n1302 = Equal To 0?(x=w2035) -> (x = 0?=w2037:bool)
                    n1303 = Select(t="dB" ("Y unit"), s=w2037, f=w2034) -> (s? t:f=w2033:string)
                  }
                  frame "WFM" {
                    n1304 = Search 1D Array(1D array=w2048, element=w2047) -> (index of element=w2046:i32)  [unwired: 1 out]
                    n1305 = Index Array(array=w2049, index=w2046) -> (element=w2041:T15)
                    n1306 = Unbundle By Name(w2041) -> ("Y data"=w2045:u16, "Y unit"=w2042:string)
                    n1307 = Equal To 0?(x=w2045) -> (x = 0?=w2044:bool)
                    n1308 = Select(t="dB" ("Y unit"), s=w2044, f=w2042) -> (s? t:f=w2040:string)
                  }
                }
              }
            }
            n1309 = local write "Unit String"(w1996) -> ()
          }
        }
      }
      event "Loudness Spectrum": Value Change {
        n1310 = event-data() -> ("NewVal"=w2050:bool)  [unwired: 6 out]
        n1311 = local read "Post Processing"() -> (w2052:T1)
        n1312 = Bundle By Name(cluster=w2052, "Zwicker_spectrum"=w2050) -> (w2051:T1)
        n1313 = local write "Post Processing"(w2051) -> ()
      }
      event "Freq Sampling Mode": Value Change {
        n1314 = event-data() -> ("NewVal"=w2056:u16)  [unwired: 6 out]
        n1315 = Equal?(x=w2056, y=u16 0) -> (x = y?=w2054:bool)
        n1316 = case shown="True" w2054 {
          tunnel: [T11."Enabled" ("Disabled") T11."Disabled and Grayed Out" ("Disabled")] -> w2053
          frame False {
            n1317 = property on="Ref Freq Mode" class="Slide (strict)"() -> ("Value"=w2060:u16)  [unwired: 2 in, 2 out]
            n1318 = Equal?(x=w2060, y=u16 0) -> (x = y?=w2062:bool)
            n1319 = case shown="False" w2062 {
              tunnel: T11."Disabled and Grayed Out" ("Disabled") -> [w2065 w2066]
              tunnel: w2060 -> [_ _]
              frame True {
                n1320 = property on="Ref Freq Mode" class="Slide (strict)"("DisabledEnum"=w2065) -> ()  [unwired: 2 in, 2 out]
                n1321 = property on="Ref Frequency" class="DigNum (strict)"("DisabledEnum"=w2065) -> ()  [unwired: 2 in, 2 out]
                n1322 = property on="Ref Wave" class="Ring (strict)"("DisabledEnum"=T11."Enabled" ("Disabled")) -> ()  [unwired: 2 in, 2 out]
              }
              frame False {
                n1323 = property on="Ref Freq Mode" class="Slide (strict)"("DisabledEnum"=w2066) -> ()  [unwired: 2 in, 2 out]
                n1324 = property on="Ref Frequency" class="DigNum (strict)"("DisabledEnum"=w2066) -> ()  [unwired: 2 in, 2 out]
                n1325 = property on="Ref Wave" class="Ring (strict)"("DisabledEnum"=w2066) -> ()  [unwired: 2 in, 2 out]
              }
            }
          }
          frame True {
            n1326 = property on="Ref Freq Mode" class="Slide (strict)"() -> ("Value"=w2069:u16)  [unwired: 2 in, 2 out]
            n1327 = property on="Ref Freq Mode" class="Slide (strict)"("DisabledEnum"=T11."Enabled" ("Disabled"), "Val(Sgnl)"=w2069) -> ()  [unwired: 2 in, 2 out]
          }
        }
        n1328 = local read "Post Processing"() -> (w2058:T1)
        n1329 = Bundle By Name(cluster=w2058, "Freq Sampling Mode"=w2056) -> (w2057:T1)
        n1330 = local write "Post Processing"(w2057) -> ()
        n1331 = property on="Freq Sampling Rate" class="DigNum (strict)"("DisabledEnum"=w2053) -> ()  [unwired: 2 in, 2 out]
      }
      event "Freq Sampling Rate": Value Change {
        n1332 = event-data() -> ("NewVal"=w2070:dbl)  [unwired: 6 out]
        n1333 = local read "Post Processing"() -> (w2072:T1)
        n1334 = Bundle By Name(cluster=w2072, "Freq Sampling Rate"=w2070) -> (w2071:T1)
        n1335 = local write "Post Processing"(w2071) -> ()
      }
      event "X_axis unit": Value Change {
        n1336 = event-data() -> ("NewVal"=w2073:u16)  [unwired: 6 out]
        n1337 = local read "Post Processing"() -> (w2075:T1)
        n1338 = Bundle By Name(cluster=w2075, "Zwciker_X-axis"=w2073) -> (w2074:T1)
        n1339 = local write "Post Processing"(w2074) -> ()
      }
      event "Smoothing_Res": Value Change {
        n1340 = event-data() -> ("NewVal"=w2076:bool)  [unwired: 6 out]
        n1341 = local read "Post Processing"() -> (w2078:T1)
        n1342 = Bundle By Name(cluster=w2078, "Smoothing"=w2076) -> (w2077:T1)
        n1343 = local write "Post Processing"(w2077) -> ()
      }
      event "Work in Statics": Value Change {
        n1344 = event-data() -> ("NewVal"=w2079:u16)  [unwired: 6 out]
        n1345 = local read "Post Processing"() -> (w2081:T1)
        n1346 = Bundle By Name(cluster=w2081, "Work in Statics"=w2079) -> (w2080:T1)
        n1347 = local write "Post Processing"(w2080) -> ()
      }
      event "Result Listbox": Value Change {
        n1348 = event-data() -> ("NewVal"=w2083:i32[])  [unwired: 6 out]
        n1349 = property on="Result Listbox" class="LstBox (strict)"() -> ("Item Names"=w2084:string[])  [unwired: 2 in, 2 out]
        n1350 = for {
          tunnel: w2084 -> [w2088]
          tunnel: w2083 -> [w2089] mode=indexing
          tunnel: [w2087] -> w2082 mode=indexing
          n1351 = Index Array(array=w2088, index=w2089) -> (element=w2087:string)
        }
        n1352 = local read "Post Processing"() -> (w2086:T1)
        n1353 = Bundle By Name(cluster=w2086, "Result Data"=w2082) -> (w2085:T1)
        n1354 = local write "Post Processing"(w2085) -> ()
      }
      event "SW_EdtObj": Value Change {
        n1355 = event-data() -> ("NewVal"=w2127:u8)  [unwired: 6 out]
        n1356 = case shown="13" w2127 {
          tunnel: [TRUE TRUE TRUE FALSE FALSE TRUE FALSE FALSE FALSE FALSE FALSE FALSE FALSE FALSE] -> w2126
          tunnel: [FALSE FALSE FALSE TRUE TRUE FALSE FALSE TRUE TRUE FALSE TRUE TRUE TRUE FALSE] -> w2124
          tunnel: [TRUE TRUE FALSE FALSE FALSE TRUE FALSE FALSE FALSE FALSE FALSE FALSE FALSE FALSE] -> w2125
          tunnel: [FALSE FALSE TRUE TRUE FALSE FALSE FALSE FALSE FALSE FALSE FALSE FALSE FALSE FALSE] -> w2123
          tunnel: [FALSE FALSE FALSE FALSE TRUE FALSE FALSE FALSE FALSE FALSE FALSE FALSE FALSE FALSE] -> w2122
          tunnel: [FALSE FALSE FALSE FALSE FALSE FALSE FALSE FALSE FALSE FALSE FALSE FALSE FALSE FALSE] -> w2121
          tunnel: [FALSE FALSE FALSE FALSE FALSE FALSE FALSE FALSE FALSE FALSE FALSE FALSE FALSE FALSE] -> w2120
          tunnel: [FALSE TRUE FALSE FALSE FALSE FALSE FALSE FALSE FALSE FALSE FALSE FALSE FALSE FALSE] -> w2119
          tunnel: [FALSE FALSE FALSE FALSE FALSE FALSE FALSE FALSE FALSE FALSE FALSE FALSE FALSE FALSE] -> w2118
          tunnel: [TRUE TRUE FALSE FALSE FALSE FALSE FALSE FALSE FALSE FALSE FALSE FALSE FALSE FALSE] -> w2117
          tunnel: [FALSE FALSE FALSE FALSE FALSE FALSE FALSE FALSE FALSE FALSE FALSE FALSE FALSE FALSE] -> w2116
          tunnel: [FALSE FALSE FALSE FALSE FALSE FALSE FALSE FALSE FALSE FALSE FALSE FALSE FALSE FALSE] -> w2115
          tunnel: [FALSE FALSE FALSE FALSE FALSE FALSE FALSE FALSE FALSE FALSE FALSE FALSE FALSE FALSE] -> w2114
          tunnel: [FALSE FALSE FALSE FALSE FALSE FALSE FALSE FALSE FALSE FALSE FALSE FALSE FALSE FALSE] -> w2113
          tunnel: [FALSE FALSE FALSE FALSE FALSE FALSE FALSE FALSE FALSE TRUE FALSE FALSE FALSE FALSE] -> w2112
          tunnel: [FALSE FALSE FALSE FALSE FALSE FALSE FALSE FALSE FALSE FALSE FALSE FALSE TRUE FALSE] -> w2111
          tunnel: [FALSE FALSE FALSE w2226 FALSE TRUE FALSE TRUE FALSE FALSE FALSE FALSE FALSE FALSE] -> w2110
          tunnel: [FALSE FALSE FALSE FALSE FALSE TRUE FALSE FALSE FALSE FALSE FALSE FALSE FALSE FALSE] -> w2109
          tunnel: [FALSE FALSE FALSE FALSE FALSE FALSE TRUE FALSE FALSE FALSE FALSE FALSE FALSE FALSE] -> w2108
          tunnel: [FALSE FALSE FALSE FALSE FALSE FALSE FALSE FALSE TRUE FALSE TRUE FALSE FALSE FALSE] -> w2107
          tunnel: [FALSE FALSE FALSE FALSE FALSE FALSE FALSE FALSE FALSE FALSE FALSE TRUE FALSE FALSE] -> w2106
          tunnel: [TRUE FALSE FALSE FALSE FALSE FALSE FALSE FALSE FALSE FALSE FALSE FALSE FALSE FALSE] -> w2105
          tunnel: [TRUE TRUE TRUE TRUE TRUE TRUE FALSE TRUE TRUE TRUE TRUE TRUE TRUE TRUE] -> w2104
          tunnel: [FALSE FALSE TRUE FALSE FALSE FALSE FALSE FALSE FALSE FALSE FALSE FALSE FALSE FALSE] -> w2103
          tunnel: [FALSE TRUE FALSE FALSE FALSE FALSE FALSE FALSE FALSE FALSE FALSE FALSE FALSE FALSE] -> w2102
          tunnel: [TRUE TRUE TRUE FALSE FALSE FALSE FALSE FALSE FALSE FALSE FALSE FALSE FALSE FALSE] -> w2101
          tunnel: [TRUE TRUE TRUE FALSE FALSE FALSE FALSE FALSE FALSE FALSE FALSE FALSE FALSE FALSE] -> w2100
          tunnel: [TRUE FALSE FALSE FALSE FALSE TRUE FALSE FALSE FALSE FALSE FALSE FALSE FALSE FALSE] -> w2099
          tunnel: [TRUE FALSE FALSE FALSE FALSE TRUE FALSE FALSE FALSE FALSE FALSE FALSE FALSE FALSE] -> w2098
          tunnel: [FALSE FALSE FALSE TRUE FALSE FALSE FALSE FALSE FALSE FALSE FALSE FALSE FALSE FALSE] -> w2097
          tunnel: [_ _ _ _ _ _ _ _ _ _ _ _ TRUE FALSE] -> w2096
          tunnel: [_ _ _ _ _ _ _ _ _ _ _ _ TRUE FALSE] -> w2095
          tunnel: [_ _ _ _ _ _ _ _ _ _ _ _ TRUE FALSE] -> w2094
          tunnel: [_ _ _ _ _ _ _ _ TRUE ("Visible") _ _ _ _ _] -> w2093
          tunnel: [_ _ _ w2224 _ _ _ _ _ _ _ _ _ _] -> w2092
          tunnel: [_ _ _ _ _ _ _ _ _ _ _ _ _ TRUE] -> w2091
          tunnel: [w2130 w2161 w2192 w2223 w2259 w2290 w2321 w2352 w2383 w2415 w2446 w2477 w2508 T11."Disabled and Grayed Out" ("Disabled")] -> _
          tunnel: T11."Enabled" ("Disabled") -> [w2130 w2161 w2192 w2223 w2259 w2290 w2321 w2352 w2383 w2415 w2446 w2477 w2508 _]
          frame 0, Default {
            # "Arith"
          }
          frame 1 {
            # "Constant"
          }
          frame 2 {
            # "Unary"
          }
          frame 3 {
            # "Scalar"
            n1357 = local read "Statistical Operator"() -> (w2227:u16)
            n1358 = case shown="0" w2227 {
              tunnel: [TRUE FALSE _] -> w2226
              tunnel: [_ _ TRUE] -> w2224
              frame Default {
              }
              frame 15 {
              }
              frame 0 {
              }
            }
          }
          frame 4 {
            # "Smoothing"
          }
          frame 5 {
            # "Intersection"
          }
          frame 6 {
            # "User Equation"
          }
          frame 7 {
            # "Windowing"
          }
          frame 8 {
          }
          frame 9 {
            # "Directivity Index"
          }
          frame 10 {
          }
          frame 11 {
            # "Resampling"
          }
          frame 12 {
            # "Shift"
          }
          frame 13 {
            # "Shift"
          }
        }
        n1359 = disable-structure shown="Disabled" {
          disable-tunnel: w2101 -> [w2129 _]
          disable-tunnel: w2100 -> [w2128 _]
          frame Disabled {
            n1360 = property on="Value_A" class="Str"("Visible"=w2129) -> ()  [unwired: 2 in, 2 out]
            n1361 = property on="unit_A" class="Str"("Visible"=w2128) -> ()  [unwired: 2 in, 2 out]
          }
          frame Enabled {
          }
        }
        n1362 = property on="OpA1 Tab" class="TabCtl (strict)"("Visible"=w2126) -> ()  [unwired: 2 in, 2 out]
        n1363 = property on="Mode_A" class="Slide (strict)"("Visible"=w2119) -> ()  [unwired: 2 in, 2 out]
        n1364 = property on="Window Tab" class="TabCtl (strict)"("Visible"=w2116) -> ()  [unwired: 2 in, 2 out]
        n1365 = property on="Direct Tab" class="TabCtl (strict)"("Visible"=w2112) -> ()  [unwired: 2 in, 2 out]
        n1366 = property on="Equation Tab" class="TabCtl (strict)"("Visible"=w2108) -> ()  [unwired: 2 in, 2 out]
        n1367 = property on="Desired Tab" class="TabCtl (strict)"("Visible"=w2104) -> ()  [unwired: 2 in, 2 out]
        n1368 = property on="Work in Statics" class="Slide (strict)"("Visible"=w2092) -> ()  [unwired: 2 in, 2 out]
        n1369 = property on="Freq Sampling" class="Bool (strict)"("Visible"=w2096) -> ()  [unwired: 2 in, 2 out]
        n1370 = property on="OpA2 Tab" class="TabCtl (strict)"("Visible"=w2124) -> ()  [unwired: 2 in, 2 out]
        n1371 = property on="Mode_B" class="Slide (strict)"("Visible"=w2118) -> ()  [unwired: 2 in, 2 out]
        n1372 = property on="Sampling Tab" class="TabCtl (strict)"("Visible"=w2115) -> ()  [unwired: 2 in, 2 out]
        n1373 = property on="Freq Tab" class="TabCtl (strict)"("Visible"=w2111) -> ()  [unwired: 2 in, 2 out]
        n1374 = property on="Org_res Tab" class="TabCtl (strict)"("Visible"=w2107) -> ()  [unwired: 2 in, 2 out]
        n1375 = property on="Unary Operator" class="Ring (strict)"("Visible"=w2103) -> ()  [unwired: 2 in, 2 out]
        n1376 = property on="Freq Sampling Mode" class="Slide (strict)"("Visible"=w2095) -> ()  [unwired: 2 in, 2 out]
        n1377 = property on="OpB Tab" class="TabCtl (strict)"("Visible"=w2125) -> ()  [unwired: 2 in, 2 out]
        n1378 = property on="Value_B" class="Str"("Visible"=w2099) -> ()  [unwired: 2 in, 2 out]
        n1379 = property on="Operation1 Tab" class="TabCtl (strict)"("Visible"=w2117) -> ()  [unwired: 2 in, 2 out]
        n1380 = property on="Smooth Tab" class="TabCtl (strict)"("Visible"=w2114) -> ()  [unwired: 2 in, 2 out]
        n1381 = property on="Sear_range Tab" class="TabCtl (strict)"("Visible"=w2110) -> ()  [unwired: 2 in, 2 out]
        n1382 = property on="Org_samp Tab" class="TabCtl (strict)"("Visible"=w2106) -> ()  [unwired: 2 in, 2 out]
        n1383 = property on="Statistical Operator" class="Ring (strict)"("Visible"=w2097) -> ()  [unwired: 2 in, 2 out]
        n1384 = property on="Constant" class="DigNum (strict)"("Visible"=w2102) -> ()  [unwired: 2 in, 2 out]
        n1385 = property on="unit_B" class="Str"("Visible"=w2098) -> ()  [unwired: 2 in, 2 out]
        n1386 = property on="Operation2 Tab" class="TabCtl (strict)"("Visible"=w2123) -> ()  [unwired: 2 in, 2 out]
        n1387 = property on="Param Tab" class="TabCtl (strict)"("Visible"=w2113) -> ()  [unwired: 2 in, 2 out]
        n1388 = property on="Sear_type Tab" class="TabCtl (strict)"("Visible"=w2109) -> ()  [unwired: 2 in, 2 out]
        n1389 = property on="Smoothing_Res" class="Bool (strict)"("Visible"=w2093) -> ()  [unwired: 2 in, 2 out]
        n1390 = property on="Result_axis Tab" class="TabCtl (strict)"("Visible"=w2105) -> ()  [unwired: 2 in, 2 out]
        n1391 = property on="Freq Sampling Rate" class="DigNum (strict)"("Visible"=w2094) -> ()  [unwired: 2 in, 2 out]
        n1392 = property on="Width Tab" class="TabCtl (strict)"("Visible"=w2122) -> ()  [unwired: 2 in, 2 out]
        n1393 = property on="Weight_fun Tab" class="TabCtl (strict)"("Visible"=w2121) -> ()  [unwired: 2 in, 2 out]
        n1394 = property on="Zwicker_func Tab" class="TabCtl (strict)"("Visible"=w2120) -> ()  [unwired: 2 in, 2 out]
        n1395 = property on="Boolean_type Tab" class="TabCtl (strict)"("Visible"=w2091) -> ()  [unwired: 2 in, 2 out]
      }
      event "Show Calcu": Value Change {
        n1396 = event-data() -> ()  [unwired: 7 out]
        n1397 = local read "Type"() -> (w2577:u16)
        n1398 = case shown="1" w2577 {
          tunnel: ["" w2580] -> w2578
          frame 0, Default {
          }
          frame 1 {
            n1399 = local read "tmp Val_A"() -> (w2582:dbl)
            n1400 = Not A Number/Path/Refnum?(number/path/refnum=w2582) -> (NaN/Path/Refnum?=w2581:bool)
            n1401 = case shown="False" w2581 {
              tunnel: [w2584 w2590] -> w2580
              frame True {
                n1402 = local read "tmp Val_B"() -> (w2587:dbl)
                n1403 = Not A Number/Path/Refnum?(number/path/refnum=w2587) -> (NaN/Path/Refnum?=w2586:bool)
                n1404 = case shown="True" w2586 {
                  tunnel: [16 ("Error No") 18 ("Error No")] -> w2583
                  frame False {
                  }
                  frame True {
                  }
                }
                n1405 = call "CRYGet Error Message.vi"("Error No"=w2583, "Kind"="Post Processing") -> ("Message Sub 3"=w2584:string)  [unwired: 4 in, 5 out]
              }
              frame False {
                n1406 = local read "tmp Val_B"() -> (w2592:dbl)
                n1407 = Not A Number/Path/Refnum?(number/path/refnum=w2592) -> (NaN/Path/Refnum?=w2591:bool)
                n1408 = case shown="False" w2591 {
                  tunnel: [w2593 w2762] -> w2590
                  frame False {
                    n1409 = local read "Work in"() -> (w2594:u16)
                    n1410 = case shown="1" w2594 {
                      tunnel: [w2595 w2647 w2675] -> w2593
                      frame 0, Default {
                        # "dB"
                        n1411 = local read "A log/lin"() -> (w2596:u16)
                        n1412 = case shown="1, Default" w2596 {
                          tunnel: [w2598 w2618] -> w2595
                          frame 1, Default {
                            # "log"
                            n1413 = local read "binary operation"() -> (w2597:u16)
                            n1414 = case shown="0" w2597 {
                              tunnel: [w2600 w2608 w2611] -> w2598
                              frame 1 {
                                n1415 = local read "tmp Val_B"() -> (w2604:dbl)
                                n1416 = local read "tmp Val_A"() -> (w2605:dbl)
                                n1417 = Format Value(format string="%#f", value (0)=w2605) -> (output string=w2602:string)  [unwired: 1 in]
                                n1418 = Format Value(format string="%#f", value (0)=w2604) -> (output string=w2601:string)  [unwired: 1 in]
                                n1419 = Concatenate Strings(w2602, " - " ("string"), w2601) -> (w2600:string)
                              }
                              frame Default {
                                n1420 = call "CRYGet Error Message.vi"("Error No"=0, "Kind"="Post Processing") -> ("Message Sub 3"=w2608:string)  [unwired: 4 in, 5 out]
                              }
                              frame 0 {
                                n1421 = local read "tmp Val_B"() -> (w2615:dbl)
                                n1422 = local read "tmp Val_A"() -> (w2616:dbl)
                                n1423 = Format Value(format string="%#f", value (0)=w2616) -> (output string=w2613:string)  [unwired: 1 in]
                                n1424 = Format Value(format string="%#f", value (0)=w2615) -> (output string=w2612:string)  [unwired: 1 in]
                                n1425 = Concatenate Strings(w2613, " + " ("string"), w2612) -> (w2611:string)
                              }
                            }
                          }
                          frame 2 {
                            # "lin"
                            n1426 = local read "binary operation"() -> (w2619:u16)
                            n1427 = case shown="0" w2619 {
                              tunnel: [w2620 w2632 w2645] -> w2618
                              frame 0 {
                                # "+"
                                n1428 = local read "tmp Val_B"() -> (w2629:dbl)
                                n1429 = local read "tmp Val_A"() -> (w2630:dbl)
                                n1430 = Divide(x=w2630, y=20.0) -> (x/y=w2625:dbl)
                                n1431 = Divide(x=w2629, y=20.0) -> (x/y=w2623:dbl)
                                n1432 = Format Value(format string="10^(%#.3f", value (0)=w2625) -> (output string=w2627:string)  [unwired: 1 in]
                                n1433 = Format Value(format string="%#.3f)", value (0)=w2623) -> (output string=w2626:string)  [unwired: 1 in]
                                n1434 = Concatenate Strings(w2627, " + ", w2626) -> (w2620:string)
                              }
                              frame 1 {
                                # "-"
                                n1435 = local read "tmp Val_B"() -> (w2641:dbl)
                                n1436 = local read "tmp Val_A"() -> (w2642:dbl)
                                n1437 = Divide(x=w2642, y=20.0) -> (x/y=w2637:dbl)
                                n1438 = Divide(x=w2641, y=20.0) -> (x/y=w2635:dbl)
                                n1439 = Format Value(format string="10^(%#.2f", value (0)=w2637) -> (output string=w2639:string)  [unwired: 1 in]
                                n1440 = Format Value(format string="%#.2f)", value (0)=w2635) -> (output string=w2638:string)  [unwired: 1 in]
                                n1441 = Concatenate Strings(w2639, " - ", w2638) -> (w2632:string)
                              }
                              frame Default {
                                n1442 = call "CRYGet Error Message.vi"("Error No"=0, "Kind"="Post Processing") -> ("Message Sub 3"=w2645:string)  [unwired: 4 in, 5 out]
                              }
                            }
                          }
                        }
                      }
                      frame 1 {
                        # "lin"
                        n1443 = local read "A log/lin"() -> (w2648:u16)
                        n1444 = case shown="2" w2648 {
                          tunnel: [w2650 w2662] -> w2647
                          frame 1, Default {
                            # "log"
                            n1445 = local read "binary operation"() -> (w2657:u16)
                            n1446 = case shown="3" w2657 {
                              tunnel: [" + " " - " " * " " / "] -> w2651
                              frame 0, Default {
                                # "+"
                              }
                              frame 1 {
                                # "-"
                              }
                              frame 2 {
                                # "*"
                              }
                              frame 3 {
                                # "/"
                              }
                            }
                            n1447 = local read "tmp Val_A"() -> (w2649:dbl)
                            n1448 = local read "tmp Val_B"() -> (w2655:dbl)
                            n1449 = Format Value(format string="20*log(%#.3f", value (0)=w2649) -> (output string=w2653:string)  [unwired: 1 in]
                            n1450 = Format Value(format string="%#.3f)", value (0)=w2655) -> (output string=w2652:string)  [unwired: 1 in]
                            n1451 = Concatenate Strings(w2653, w2651, w2652) -> (w2650:string)
                          }
                          frame 2 {
                            # "lin"
                            n1452 = local read "binary operation"() -> (w2670:u16)
                            n1453 = case shown="3" w2670 {
                              tunnel: [" + " " - " " * " " / "] -> w2663
                              frame 0, Default {
                                # "+"
                              }
                              frame 1 {
                                # "-"
                              }
                              frame 2 {
                                # "*"
                              }
                              frame 3 {
                                # "/"
                              }
                            }
                            n1454 = local read "tmp Val_B"() -> (w2667:dbl)
                            n1455 = local read "tmp Val_A"() -> (w2668:dbl)
                            n1456 = Format Value(format string="%#f", value (0)=w2668) -> (output string=w2665:string)  [unwired: 1 in]
                            n1457 = Format Value(format string="%#f", value (0)=w2667) -> (output string=w2664:string)  [unwired: 1 in]
                            n1458 = Concatenate Strings(w2665, w2663, w2664) -> (w2662:string)
                          }
                        }
                      }
                      frame 2 {
                        # "Pow"
                        n1459 = local read "A log/lin"() -> (w2676:u16)
                        n1460 = case shown="1, Default" w2676 {
                          tunnel: [w2677 w2719] -> w2675
                          frame 2 {
                            # "lin"
                            n1461 = local read "binary operation"() -> (w2678:u16)
                            n1462 = case shown="1" w2678 {
                              tunnel: [w2680 w2690 w2702 w2712] -> w2677
                              frame 0, Default {
                                # "+"
                                n1463 = local read "tmp Val_B"() -> (w2685:dbl)
                                n1464 = local read "tmp Val_A"() -> (w2679:dbl)
                                n1465 = Square(x=w2679) -> (x^2=w2687:dbl)
                                n1466 = Square(x=w2685) -> (x^2=w2684:dbl)
                                n1467 = Format Value(format string="(%#.3f", value (0)=w2687) -> (output string=w2683:string)  [unwired: 1 in]
                                n1468 = Format Value(format string="%#.3f)^1/2", value (0)=w2684) -> (output string=w2682:string)  [unwired: 1 in]
                                n1469 = Concatenate Strings(w2683, " + ", w2682) -> (w2680:string)
                              }
                              frame 1 {
                                # "+"
                                n1470 = local read "tmp Val_B"() -> (w2695:dbl)
                                n1471 = local read "tmp Val_A"() -> (w2689:dbl)
                                n1472 = Square(x=w2689) -> (x^2=w2697:dbl)
                                n1473 = Square(x=w2695) -> (x^2=w2694:dbl)
                                n1474 = Format Value(format string="(|%#.3f", value (0)=w2697) -> (output string=w2693:string)  [unwired: 1 in]
                                n1475 = Format Value(format string="%#.3f|)^1/2", value (0)=w2694) -> (output string=w2692:string)  [unwired: 1 in]
                                n1476 = Concatenate Strings(w2693, " - ", w2692) -> (w2690:string)
                              }
                              frame 2 {
                                # "+"
                                n1477 = local read "tmp Val_B"() -> (w2701:dbl)
                                n1478 = local read "tmp Val_A"() -> (w2699:dbl)
                                n1479 = Square(x=w2699) -> (x^2=w2707:dbl)
                                n1480 = Absolute Value(x=w2701) -> (abs(x)=w2700:dbl)
                                n1481 = Format Value(format string="(%#.3f", value (0)=w2707) -> (output string=w2705:string)  [unwired: 1 in]
                                n1482 = Format Value(format string="%#.3f)^1/2", value (0)=w2700) -> (output string=w2704:string)  [unwired: 1 in]
                                n1483 = Concatenate Strings(w2705, " * ", w2704) -> (w2702:string)
                              }
                              frame 3 {
                                # "+"
                                n1484 = local read "tmp Val_B"() -> (w2711:dbl)
                                n1485 = local read "tmp Val_A"() -> (w2709:dbl)
                                n1486 = Square(x=w2709) -> (x^2=w2717:dbl)
                                n1487 = Absolute Value(x=w2711) -> (abs(x)=w2710:dbl)
                                n1488 = Format Value(format string="(%#.3f", value (0)=w2717) -> (output string=w2715:string)  [unwired: 1 in]
                                n1489 = Format Value(format string="%#.3f)^1/2", value (0)=w2710) -> (output string=w2714:string)  [unwired: 1 in]
                                n1490 = Concatenate Strings(w2715, " / ", w2714) -> (w2712:string)
                              }
                            }
                          }
                          frame 1, Default {
                            # "log"
                            n1491 = local read "binary operation"() -> (w2720:u16)
                            n1492 = case shown="1" w2720 {
                              tunnel: [w2722 w2732 w2744 w2754] -> w2719
                              frame 0, Default {
                                # "+"
                                n1493 = local read "tmp Val_B"() -> (w2727:dbl)
                                n1494 = local read "tmp Val_A"() -> (w2721:dbl)
                                n1495 = Square(x=w2721) -> (x^2=w2729:dbl)
                                n1496 = Square(x=w2727) -> (x^2=w2726:dbl)
                                n1497 = Format Value(format string="20*log((%#.3f", value (0)=w2729) -> (output string=w2725:string)  [unwired: 1 in]
                                n1498 = Format Value(format string="%#.3f)^1/2)", value (0)=w2726) -> (output string=w2724:string)  [unwired: 1 in]
                                n1499 = Concatenate Strings(w2725, " + ", w2724) -> (w2722:string)
                              }
                              frame 1 {
                                # "+"
                                n1500 = local read "tmp Val_B"() -> (w2737:dbl)
                                n1501 = local read "tmp Val_A"() -> (w2731:dbl)
                                n1502 = Square(x=w2731) -> (x^2=w2739:dbl)
                                n1503 = Square(x=w2737) -> (x^2=w2736:dbl)
                                n1504 = Format Value(format string="20*log((|%#.3f", value (0)=w2739) -> (output string=w2735:string)  [unwired: 1 in]
                                n1505 = Format Value(format string="%#.3f|)^1/2)", value (0)=w2736) -> (output string=w2734:string)  [unwired: 1 in]
                                n1506 = Concatenate Strings(w2735, " - ", w2734) -> (w2732:string)
                              }
                              frame 2 {
                                # "*"
                                n1507 = local read "tmp Val_B"() -> (w2743:dbl)
                                n1508 = local read "tmp Val_A"() -> (w2741:dbl)
                                n1509 = Square(x=w2741) -> (x^2=w2749:dbl)
                                n1510 = Absolute Value(x=w2743) -> (abs(x)=w2742:dbl)
                                n1511 = Format Value(format string="20*log((%#.3f", value (0)=w2749) -> (output string=w2747:string)  [unwired: 1 in]
                                n1512 = Format Value(format string="%#.3f)^1/2)", value (0)=w2742) -> (output string=w2746:string)  [unwired: 1 in]
                                n1513 = Concatenate Strings(w2747, " * ", w2746) -> (w2744:string)
                              }
                              frame 3 {
                                # "/"
                                n1514 = local read "tmp Val_B"() -> (w2753:dbl)
                                n1515 = local read "tmp Val_A"() -> (w2751:dbl)
                                n1516 = Absolute Value(x=w2753) -> (abs(x)=w2752:dbl)
                                n1517 = Square(x=w2751) -> (x^2=w2759:dbl)
                                n1518 = Format Value(format string="20*log((%#.3f", value (0)=w2759) -> (output string=w2757:string)  [unwired: 1 in]
                                n1519 = Format Value(format string="%#.3f)^1/2)", value (0)=w2752) -> (output string=w2756:string)  [unwired: 1 in]
                                n1520 = Concatenate Strings(w2757, " / ", w2756) -> (w2754:string)
                              }
                            }
                          }
                        }
                      }
                    }
                  }
                  frame True {
                    n1521 = call "CRYGet Error Message.vi"("Error No"=17, "Kind"="Post Processing") -> ("Message Sub 3"=w2762:string)  [unwired: 4 in, 5 out]
                  }
                }
              }
            }
          }
        }
        n1522 = property on="Work in" class="Slide (strict)"("TipStrip"=w2578) -> ()  [unwired: 2 in, 2 out]
      }
    }
    n1523 = disable-structure shown="Disabled" {
      frame Disabled {
        n1524 = property on="Work in" class="Slide (strict)"("TipStrip"="") -> ()  [unwired: 2 in, 2 out]
        n1525 = call "CRYChange post_xyz mode.vi"() -> ()  [unwired: 6 in, 6 out]
        n1526 = local read "Work in"() -> (w69:u16)
        n1527 = local read "Constant"() -> (w68:dbl)
        n1528 = call "CRYSet Constant to TipStrip.vi"("Work in"=w69, "Constant"=w68) -> ("Tip Out"=w70:string)  [unwired: 9 in]
        n1529 = property on="Constant" class="DigNum (strict)"("TipStrip"=w70) -> ()  [unwired: 2 in, 2 out]
      }
      frame Enabled {
      }
    }
    n1530 = global read "CRYMain Sub Window Global.vi" "gStop"() -> (w58:bool)
    n1531 = Or(x="stop", y=w58) -> (x .or. y?=w55:bool)
    n1532 = Bundle("Load Test"="Load Test", "Apply"="Apply", "Unit_Cont"="Unit_Cont", "Edit Range"="Edit Range", "Clear All Fields"="Clear All Fields", "Add Lib"="Add Lib", "OK"="OK", "Cancel"="Cancel") -> (w64:T17)  [unwired: 1 out]
    n1533 = Cluster To Array(cluster=w64) -> (array=w63:bool[])
    n1534 = Search 1D Array(1D array=w63, element=TRUE) -> (index of element=w59:i32)  [unwired: 1 out]
    n1535 = case shown="5" w59 {
      tunnel: w52 -> [_ w71 _ _ _ _ _ _ _]
      tunnel: w50 -> [_ _ w173 _ _ _ _ _ _]
      frame Default {
      }
      frame 0 {
        n1536 = stacked-sequence {
          seq-local: [w87 _ _ _ _ _] -> [_ w164 _ _ _ _]
          tunnel: w71 -> [w73 _ _ _ _ _]
          frame #0 {
            w92 = 1.0 ("y")
            n1537 = local read "Post Processing"() -> (w156:T1)
            n1538 = Unbundle By Name(w156) -> ("Result Name"=w155:string, "Op Type"=w87:u16, "Curve A"=→"A_cur name":string, "Curve B"=→"B_cur name":string, "Axis Mode"=w154:u16, "Work Mode"=w80:u16, "Binary Operator"=w85:u16, "Unit"=w149:string, "Use Default Name"=w148:bool, "x"=w147:bool, "y"=w146:bool, "z"=w145:bool, "A_single val axis"=w138:u16, "B_single val axis"=w135:u16, "Constant"=w141:dbl, "Unary Operator"=w134:u16, "Smoothing Width"=w133:i32, "Window"=w132:u16, "Sampling Rate"=w86:dbl, "All points"=w129:bool, "Search Items"=w128:string[], "Statistical Operator"=w127:u16, "Para_dB"=w126:sgl, "Para_%"=w125:sgl, "Use Default Value"=w124:bool, "Exponent"=w84:sgl, "Weighting Curve"=w121:string, "Width"=w99:u16, "Hz"=w118:dbl, "Weighting win"=w117:u16, "Search Mode"=w116:u16, "New Resolution"=w102:u16, "Freq Mode"=w115:u16, "Curve Group"=w114:string[], "Direct Weighting"=w112:bool, "Auto Inc"=w111:bool, "Inc(deg)"=w110:i32, "Total Rotation"=w109:i32, "New Sampling Rate"=w90:dbl, "Ref Freq Mode"=w108:u16, "Ref Freq"=w106:dbl, "Ref Waveform"=→"Ref Waveform":string, "Custom unit info"=w97:T3, "user equation cluster"=w96:T2, "Help"=w94:string, "Tab Value"=w93:enum32{"Setting", "Help"}, "Freq Sampling Mode"=w83:u16, "Freq Sampling Rate"=w82:dbl, "Smoothing"=w81:bool, "Work in Statics"=w72:u16, "Result Data"=w75:string[])
            "Result Data" <- w75
            n1539 = local write "Frequencies"(w115) -> ()
            n1540 = local write "Constant"(w141) -> ()
            n1541 = local write "dB"(w126) -> ()
            n1542 = local write "Win Mode"(w132) -> ()
            n1543 = local write "Name"(w155) -> ()
            n1544 = local write "Weight Mode"(w117) -> ()
            n1545 = local write "Use Default Exp"(w124) -> ()
            n1546 = local write "Ref Freq Mode"(w108) -> ()
            n1547 = local write "Search Items"(w128) -> ()
            n1548 = local write "Total Rotation"(w109) -> ()
            n1549 = Bundle("x"=w147, "y"=w146, "z"=w145) -> (w142:cluster{"x":bool, "y":bool, "z":bool})  [unwired: 1 out]
            n1550 = local write "Auto Inc"(w111) -> ()
            n1551 = local write "Custom unit info"(w97) -> ()
            n1552 = local write "Use default"(w148) -> ()
            n1553 = local write "Smoo Width"(w133) -> ()
            n1554 = local write "Unit String"(w149) -> ()
            n1555 = local write "Axis Mode"(w154) -> ()
            n1556 = local write "Exponent"(w84) -> ()
            n1557 = local write "%"(w125) -> ()
            n1558 = local write "Unary Operator"(w134) -> ()
            n1559 = local write "Search Mode"(w116) -> ()
            n1560 = local write "Direct_weight"(w112) -> ()
            n1561 = local write "Ref Frequency"(w106) -> ()
            n1562 = local write "Inc(deg.)"(w110) -> ()
            n1563 = local write "Statistical Operator"(w127) -> ()
            n1564 = local write "Old Exponent"(w84) -> ()
            n1565 = property on="Freq Sampling Mode" class="Slide (strict)"("Value"=w83) -> ()  [unwired: 2 in, 2 out]
            n1566 = property on="Freq Sampling Rate" class="DigNum (strict)"("Value"=w82) -> ()  [unwired: 2 in, 2 out]
            n1567 = property on="Samp Rate" class="DigNum (strict)"("Value"=w86) -> ()  [unwired: 2 in, 2 out]
            n1568 = local read "Work array"() -> (w153:u16[])
            n1569 = local read "Ope_array"() -> (w151:u16[])
            n1570 = local write "binary operation"(w85) -> ()
            n1571 = property on="Smoothing_Res" class="Bool (strict)"("Value"=w81) -> ()  [unwired: 2 in, 2 out]
            n1572 = Index Array(array=string[] ["1/1 Octave", "1/3 Octave", "1/6 Octave", "1/12 Octave", "1/24 Octave", "User Defined log", "User Defined lin"] ("Array"), index=w99) -> (element=→"Width name":string)
            n1573 = Replace Array Subset(array=w151, new element=w85, index=w87) -> (w150:u16[])
            n1574 = Replace Array Subset(array=w153, new element=w80, index=w87) -> (w152:u16[])
            n1575 = local write "Work in Statics"(w72) -> ()
            n1576 = local write "Ope_array"(w150) -> ()
            n1577 = local write "Work array"(w152) -> ()
            n1578 = call "CRYFlatten User Equation Cluster.vi"("user equation cluster"=w96) -> ("Flatten String"=w79:string)  [unwired: 10 in]
            n1579 = local read "Hz_oct array"() -> (w120:dbl[])
            n1580 = Less?(x=w90, y=w92) -> (x < y?=w91:bool)
            n1581 = call "CRYGetPost Pro_all data.vi"("No.VI"=w73) -> ("Curve Names"=w95:string[])  [unwired: 1 in, 13 out]
            n1582 = local read "Weight_Cur array"() -> (w123:string[])
            n1583 = property on="Help" class="Str"("Value"=w94) -> ()  [unwired: 2 in, 2 out]
            n1584 = local write "User Equation String"(w79) -> ()
            n1585 = local read "A_xyz array"() -> (w140:u16[])
            n1586 = local write "Work in"(w80) -> ()
            n1587 = local read "B_xyz array"() -> (w137:u16[])
            n1588 = Select(t=w92, s=w91, f=w90) -> (s? t:f=w89:dbl)
            n1589 = local read "Show xyz"() -> (w144:cluster{"x":bool, "y":bool, "z":bool}[])
            n1590 = local read "All array"() -> (w131:bool[])
            n1591 = for {
              tunnel: w95 -> [w163]
              tunnel: w114 -> [w162] mode=indexing
              tunnel: [w161] -> w113 mode=indexing
              n1592 = Search 1D Array(1D array=w163, element=w162) -> (index of element=w161:i32)  [unwired: 1 out]
            }
            n1593 = case shown="8, Default" w87 {
              tunnel: [string[] ["1/1 Octave", "1/3 Octave", "1/6 Octave", "1/12 Octave", "1/24 Octave", "User Defined log", "User Defined lin"] ("Array") string[] ["1/1 Octave", "1/3 Octave", "1/6 Octave", "1/12 Octave", "1/24 Octave"] ("Array")] -> w103
              frame 8, Default {
              }
              frame 10 {
              }
            }
            n1594 = local write "New  Samp Val"(w89) -> ()
            n1595 = Replace Array Subset(array=w120, new element=w118, index=w87) -> (w119:dbl[])
            n1596 = property on="Main Tab" class="TabCtl (strict)"("Value"=w93) -> ()  [unwired: 2 in, 2 out]
            n1597 = local write "Hz_oct array"(w119) -> ()
            n1598 = call "CRYGet Upper Step Data.vi"("Type In"=enum16{"Curves", "Values", "Results", "WFM"}."Results", "No.VI"=w73) -> ("Result array"=w77:T12)  [unwired: 9 out]
            n1599 = Replace Array Subset(array=w140, new element=w138, index=w87) -> (w139:u16[])
            n1600 = Replace Array Subset(array=w144, new element=w142, index=w87) -> (w143:cluster{"x":bool, "y":bool, "z":bool}[])
            n1601 = Replace Array Subset(array=w137, new element=w135, index=w87) -> (w136:u16[])
            n1602 = Replace Array Subset(array=w131, new element=w129, index=w87) -> (w130:bool[])
            n1603 = Replace Array Subset(array=w123, new element=w121, index=w87) -> (w122:string[])
            n1604 = local write "Curve List"(w113) -> ()
            n1605 = for {
              tunnel: w77 -> [w158] mode=indexing
              tunnel: [w157] -> w74 mode=indexing
              n1606 = Unbundle By Name(w158) -> ("Name"=w157:string)
            }
            n1607 = local write "A_xyz array"(w139) -> ()
            n1608 = local write "Show xyz"(w143) -> ()
            n1609 = local write "Weight_Cur array"(w122) -> ()
            n1610 = local write "B_xyz array"(w136) -> ()
            n1611 = local write "All array"(w130) -> ()
            n1612 = call "CRYSelect DAT&RES list.vi"("Selected Result Item"=w75, "Result Names"=w74) -> ("Result Index"=w78:i32[])  [unwired: 3 in, 10 out]
            n1613 = local write "Loading_F"(TRUE ("Loading_F")) -> ()
            n1614 = property on="Result Listbox" class="LstBox (strict)"("Value"=w78) -> ()  [unwired: 2 in, 2 out]
            n1615 = Index Array(array=w103, index=w102) -> (element=→"New_res str":string)
          }
          frame #1 {
            n1616 = property on="Type" class="Ring (strict)"("Val(Sgnl)"=w164) -> ()  [unwired: 2 in, 2 out]
          }
          frame #2 {
            n1617 = control-ref of="Board Tab"() -> (w167:refnum<vi>)
            n1618 = control-ref of="This VI"() -> (w165:refnum<vi>)
            n1619 = call "CRYAlign Steps VI Center.vi"("Tab2"=w167, "Input/Output"=TRUE, "VIRef"=w165) -> ()  [unwired: 1 in, 8 out]
          }
          frame #3 {
            n1620 = local write "Load Test"(FALSE ("Load Test")) -> ()
            n1621 = property on="Board Tab" class="TabCtl (strict)"("Visible"=TRUE) -> ()  [unwired: 2 in, 2 out]
          }
          frame #4 {
            n1622 = local read "AddStep"() -> (w170:bool)
            n1623 = local write "Add Lib"(w170) -> ()
          }
          frame #5 {
            n1624 = local write "AddStep"(FALSE ("AddStep")) -> ()
          }
        }
      }
      frame 1 {
        n1625 = global read "CRYMainGlobal.vi" "Access Level"() -> (w172:enum16{"Engineer", "Technician", "Operator"})
        n1626 = case shown="\"Operator\", Default" w172 {
          tunnel: w173 -> [w175 _]
          frame "Engineer" {
            n1627 = flat-sequence {
              tunnel: [w182] -> w181
              tunnel: w181 -> [w192]
              tunnel: [w192] -> w180
              tunnel: [w191] -> w179
              tunnel: [w190] -> w178
              tunnel: [w186] -> w177
              tunnel: [w185] -> w176
              tunnel: w180 -> [w222]
              tunnel: w179 -> [w219]
              tunnel: w178 -> [w215]
              tunnel: w177 -> [w201]
              tunnel: w176 -> [w195]
              tunnel: w175 -> [w193]
              frame #0 {
                n1628 = call "CRYGet Current TS Steps.vi"() -> ("SelectStepNumber in Tree"=w183:i32, "Steps"=w184:T5[])  [unwired: 1 in, 9 out]
                n1629 = Index Array(array=w184, index=w183) -> (element=w182:T5)
              }
              frame #1 {
                n1630 = local read "Post Processing"() -> (w190:T1)
                n1631 = local read "Proper VI No"() -> (w188:i32)
                n1632 = call "CRYFlatten Post Processing.vi"("Post-Processing"=w190) -> ("Post Processing flattened"=w191:string)  [unwired: 10 out]
                n1633 = Build Array(w188) -> (w187:i32[])
                n1634 = call "CRYGet Curve Library Data Name.vi"("nData"=w187, "sAction"="GetNamebyStep" ("sOption")) -> ("sNames"=w186:string[], "Type Out"=w185:string[])  [unwired: 6 in, 2 out]
              }
              frame #2 {
                n1635 = Bundle By Name(cluster=w222, "Seq setup flattened"=w219) -> (w203:T5)
                n1636 = call "CRYPost Processing Name & Unit.vi"("Step setup"=w219) -> ("Result name and type"=w221:T18)  [unwired: 6 in, 4 out]
                n1637 = Unbundle By Name(w215) -> ("user equation cluster"=w218:T2)
                n1638 = local read "Type"() -> (w200:u16)
                n1639 = local read "Custom unit info"() -> (w209:T3)
                n1640 = local read "Equ_List"() -> (w214:string)
                n1641 = case shown="Default" w200 {
                  tunnel: w221 -> [w232 w235]
                  tunnel: [w231 w234] -> w220
                  frame Default {
                    n1642 = Index Array(array=w232) -> (element=w231:T19)  [unwired: 1 in]
                  }
                  frame 12 {
                    n1643 = Index Array(array=w235, index=1) -> (element=w234:T19)
                  }
                }
                n1644 = call "CRYPost Processing.vi"("Setup in"=w203, "Step name"=w193) -> ("Types Out"=w194:string[], "Inserted Names Out"=w202:string[], "Data out"=w204:T6, "Wave out"=w210:T14)  [unwired: 5 in, 5 out]
                n1645 = Unbundle By Name(w218) -> ("# input curves"=w217:i32, "# Desired result curves"=w216:i32)
                n1646 = Unbundle By Name(w220) -> ("Res Name"=w197:string)
                n1647 = call "CRYGet Formula & Result Variable.vi"("String"=w214) -> ("Out string"=w213:string)  [unwired: 8 in, 2 out]
                n1648 = Unbundle By Name(w209) -> ("lin/log"=w205:u16, "unit"=w206:string, "use custom"=w207:bool)
                n1649 = Array Size(array=w204) -> (size(s)=w212:i32)
                n1650 = local write "Equ_List"(w213) -> ()
                n1651 = Equal To 0?(x=w212) -> (x = 0?=w211:bool)
                n1652 = Not Equal?(x="", y=w197) -> (x != y?=w198:bool)
                n1653 = case shown="False" w211 {
                  tunnel: w204 -> [w240 _]
                  tunnel: w210 -> [_ w259]
                  tunnel: [w239 w258] -> w208
                  tunnel: w207 -> [w238 w257]
                  tunnel: w206 -> [w237 w256]
                  tunnel: w205 -> [w236 _]
                  frame False {
                    n1654 = case shown="False" w238 {
                      tunnel: w240 -> [w248 _]
                      tunnel: [w246 w251] -> w239
                      tunnel: w237 -> [_ w252]
                      tunnel: w236 -> [_ w253]
                      frame False {
                        n1655 = Index Array(array=w248) -> (element=w247:T7)  [unwired: 1 in]
                        n1656 = global read "CRYPost Processing Global.vi" "disp_unit"() -> (w241:string)
                        n1657 = Unbundle By Name(w247) -> ("Y data"=w244:u16, "Y dB ref"=w242:dbl)
                        n1658 = local read "Custom unit info"() -> (w245:T3)
                        n1659 = Bundle By Name(cluster=w245, "unit"=w241, "lin/log"=w244, "dB ref"=w242) -> (w243:T3)
                        n1660 = case shown="0, Default" w244 {
                          tunnel: ["dB" ("Y unit") w250] -> w246
                          tunnel: w241 -> [_ w250]
                          frame 0, Default {
                          }
                          frame 1 {
                          }
                        }
                        n1661 = local write "Custom unit info"(w243) -> ()
                      }
                      frame True {
                        n1662 = case shown="1" w253 {
                          tunnel: w252 -> [_ w255]
                          tunnel: ["dB" ("unit") w255] -> w251
                          frame 0, Default {
                          }
                          frame 1 {
                          }
                        }
                      }
                    }
                  }
                  frame True {
                    n1663 = case shown="False" w257 {
                      tunnel: w259 -> [w268 _]
                      tunnel: [w260 w271] -> w258
                      tunnel: w256 -> [_ w271]
                      frame False {
                        n1664 = Index Array(array=w268) -> (element=w265:T15)  [unwired: 1 in]
                        n1665 = global read "CRYPost Processing Global.vi" "disp_unit"() -> (w260:string)
                        n1666 = local read "Type"() -> (w262:u16)
                        n1667 = Unbundle By Name(w265) -> ("Y data"=w267:u16, "Y dB ref"=w266:dbl)
                        n1668 = case shown="Default" w262 {
                          tunnel: ["Error(Hz)" ("disp_unit") w270] -> w261
                          tunnel: w260 -> [_ w270]
                          frame 12 {
                          }
                          frame Default {
                          }
                        }
                        n1669 = local read "Custom unit info"() -> (w264:T3)
                        n1670 = Bundle By Name(cluster=w264, "unit"=w261, "lin/log"=w267, "dB ref"=w266) -> (w263:T3)
                        n1671 = local write "Custom unit info"(w263) -> ()
                      }
                      frame True {
                      }
                    }
                  }
                }
                n1672 = case shown="True" w198 {
                  tunnel: w197 -> [_ w230]
                  frame False {
                  }
                  frame True {
                    n1673 = local write "Name"(w230) -> ()
                  }
                }
                n1674 = local write "#Desired Results"(w216) -> ()
                n1675 = local write "#Operands"(w217) -> ()
                n1676 = local read "Exponent"() -> (w196:sgl)
                n1677 = disable-structure shown="Enabled" {
                  disable-tunnel: w202 -> [w225 w229]
                  disable-tunnel: w201 -> [w224 w228]
                  disable-tunnel: w195 -> [_ w227]
                  disable-tunnel: w194 -> [_ w226]
                  frame Disabled {
                    n1678 = call "CRYReplace Curve Name of Steps.vi"("Step Category"="Post Processing", "New Name"=w225, "Old Name"=w224) -> ()  [unwired: 8 in, 1 out]
                  }
                  frame Enabled {
                    n1679 = call "CRYChange Name by Step Editor.vi"("New Names Type"=w226, "Old Names Type"=w227, "Old Names"=w228, "New Names"=w229) -> ()  [unwired: 8 in]
                  }
                }
                n1680 = local write "Old Exponent"(w196) -> ()
                n1681 = local write "Unit String"(w208) -> ()
              }
            }
          }
          frame "Operator", Default {
            n1682 = call "CRYGet Error Message.vi"("Kind"="Step Setup") -> ("Window Title"=w273:string)  [unwired: 5 in, 5 out]
            n1683 = call "CRYGet Access Level Message.vi"() -> ("Multibyte string"=w275:string)  [unwired: 11 in]
            n1684 = call "CRYMessage Dialog.vi"("Window Title"=w273, "YesNoCancel"=T8."OK", "Message Content"=w275) -> ()  [unwired: 7 in, 2 out]
          }
        }
        n1685 = local write "Apply"(FALSE ("Apply")) -> ()
      }
      frame 2 {
        n1686 = local read "Custom unit info"() -> (w280:T3)
        n1687 = Unbundle By Name(w280) -> ("lin/log"=w281:u16, "unit"=w290:string, "dB ref"=w288:dbl, "common dB"=w287:u16, "use custom"=w292:bool)
        n1688 = local read "Unit String"() -> (w276:string)
        n1689 = Bundle(TRUE, "use custom"=w292) -> (w291:cluster{bool, "use custom":bool})  [unwired: 1 out]
        n1690 = call "CRYUnits setup.vi"("Scale visible?"=TRUE, "dB/Lin"=w281, "Unit:"=w290, "dB ref:"=w288, "Custom unit settings"=w291, "Common dB ref."=w287) -> ("New Scale"=w286:u16, "New unit Lin"=w285:string, "New dB ref"=w284:dbl, "Common dB #"=w283:u16, "Use custom unit out"=w279:bool, "Cancelled?"=w277:bool)  [unwired: 2 in, 2 out]
        n1691 = case shown="True" w277 {
          tunnel: w280 -> [w301 _]
          tunnel: w283 -> [w300 _]
          tunnel: w284 -> [w299 _]
          tunnel: w285 -> [w298 _]
          tunnel: w286 -> [w297 _]
          tunnel: [w295 w302] -> w278
          tunnel: w276 -> [_ w302]
          tunnel: w279 -> [w296 _]
          frame False {
            n1692 = Bundle By Name(cluster=w301, "lin/log"=w297, "unit"=w298, "dB ref"=w299, "common dB"=w300, "use custom"=w296) -> (w294:T3)
            n1693 = call "CRYCustom Unit Text.vi"("Custom unit info"=w294) -> ("Unit indicator text"=w295:string)  [unwired: 10 out]
            n1694 = property on="Custom unit info" class="Clust (strict)"("Val(Sgnl)"=w294) -> ()  [unwired: 2 in, 2 out]
          }
          frame True {
          }
        }
        n1695 = local write "Unit_Cont"(FALSE ("Unit")) -> ()
        n1696 = property on="Unit String" class="Str"("Val(Sgnl)"=w278) -> ()  [unwired: 2 in, 2 out]
      }
      frame 3 {
        n1697 = property on="Search List" class="LstBox (strict)"() -> ("Caption.Text"=w313:string, "Item Names"=w312:string[])  [unwired: 2 in, 2 out]
        n1698 = case shown="\"s\"" w313 {
          tunnel: [w321 w322] -> w311
          frame "Hz", Default {
            n1699 = local read "Check_Hz"() -> (w321:bool[])
          }
          frame "s" {
            n1700 = local read "Check_s"() -> (w322:bool[])
          }
        }
        n1701 = call "CRYListbox Editor.vi"("In Check"=w311, "In Items"=w312, "In Type"=w313) -> ("Out Check"=w309:bool[], "Out Items"=w308:string[])  [unwired: 1 in, 5 out]
        n1702 = local write "Edit Range"(FALSE ("Edit Range")) -> ()
        n1703 = call "CRYItemCheckSort.vi"("Check_s"=w309, "In Items"=w308) -> ("Out Check"=w307:bool[], "Out Items"=w306:string[], "Chked Items"=w303:string[])  [unwired: 6 in, 1 out]
        n1704 = case shown="\"s\"" w313 {
          tunnel: w307 -> [w319 w320]
          frame "Hz", Default {
            n1705 = local write "Check_Hz"(w319) -> ()
          }
          frame "s" {
            n1706 = local write "Check_s"(w320) -> ()
          }
        }
        n1707 = local read "Post Processing"() -> (w304:T1)
        n1708 = Bundle By Name(cluster=w304, "Search Items"=w303) -> (w305:T1)
        n1709 = property on="Search List" class="LstBox (strict)"("Item Names"=w306) -> ()  [unwired: 2 in, 2 out]
        n1710 = for {
          tunnel: w307 -> [w318] mode=indexing
          tunnel: [w317] -> w314 mode=indexing
          n1711 = Select(t=0, s=w318, f=1) -> (s? t:f=w317:i32)
        }
        n1712 = local write "Post Processing"(w305) -> ()
        n1713 = property on="Search List" class="LstBox (strict)"("Item Symbols"=w314) -> ()  [unwired: 2 in, 2 out]
      }
      frame 4 {
        w323 = u32 0 ("#Desired Results")
        n1714 = global read "CRYPost Processing Global.vi" "User Equation VI Ref"() -> (w325:refnum<vi>)
        n1715 = local write "Clear All Fields"(FALSE ("Clear All Fields")) -> ()
        n1716 = call "CRYGet Boolean Reference.vi"("Label Name"="Clear All", "VI Refnum"=w325) -> ("Boolean Ref"=w327:refnum<vi>)  [unwired: 7 in, 2 out]
        n1717 = local write "#Desired Results"(w323) -> ()
        n1718 = local write "#Operands"(w323) -> ()
        n1719 = local write "Equ_List"("") -> ()
        n1720 = property class="Bool"(reference=w327, "Val(Sgnl)"=TRUE) -> ()  [unwired: 1 in, 2 out]
      }
      frame 5 {
        n1721 = flat-sequence {
          tunnel: [w341] -> w336
          tunnel: [w339] -> w335
          tunnel: [w338] -> w330
          tunnel: w336 -> [w351]
          tunnel: w335 -> [w346]
          tunnel: [w351] -> w334
          tunnel: [w345] -> w333
          tunnel: [w344] -> w331
          tunnel: w330 -> [w344]
          tunnel: w334 -> [w354]
          tunnel: w333 -> [w353]
          tunnel: [w352] -> w332
          tunnel: w331 -> [w352]
          tunnel: w332 -> [w355]
          frame #0 {
            n1722 = local read "Post Processing"() -> (w340:T1)
            n1723 = local read "Proper VI No"() -> (w338:i32)
            n1724 = Build Array(w338) -> (w343:i32[])
            n1725 = call "CRYFlatten Post Processing.vi"("Post-Processing"=w340) -> ("Post Processing flattened"=w339:string)  [unwired: 10 in]
            n1726 = call "CRYGet Curve Library Data Name.vi"("nData"=w343, "sAction"="GetNamebyStep" ("sOption")) -> ("sNames"=w341:string[])  [unwired: 6 in, 3 out]
          }
          frame #1 {
            n1727 = call "CRYGet Current TS Steps.vi"() -> ("SelectStepNumber in Tree"=w347:i32, "Steps"=w348:T5[])  [unwired: 7 in, 3 out]
            n1728 = Index Array(array=w348, index=w347) -> (element=w349:T5)
            n1729 = call "CRYPost Processing Curve Name Replace.vi"("Setup in"=w349, "Step Setup in"=w346, "Type In"="AddStep") -> ("Inserted Names Out"=w345:string[])  [unwired: 8 in]
          }
          frame #2 {
            n1730 = call "CRYReplace Curve Name of Steps.vi"("New Name"=w353, "Old Name"=w354) -> ()  [unwired: 9 in, 1 out]
          }
          frame #3 {
            n1731 = global read "CRYStepSetup Global.vi" "Load from AddStep"() -> (w356:bool)
            n1732 = case shown="True" w356 {
              tunnel: w355 -> [_ w358]
              frame False {
              }
              frame True {
                n1733 = global write "CRYStepSetup Global.vi" "Load from AddStep"(FALSE ("Load from AddStep")) -> ()
                n1734 = call "CRYStepData Manipulate.vi"("sAction"="Backup", "StepNo."=w358) -> ()  [unwired: 10 in]
              }
            }
          }
        }
        n1735 = local write "Add Lib"(FALSE ("Add Lib")) -> ()
      }
      frame 6 {
        n1736 = flat-sequence {
          frame #0 {
            n1737 = global read "CRYMainGlobal.vi" "Access Level"() -> (w361:enum16{"Engineer", "Technician", "Operator"})
            n1738 = case shown="\"Engineer\"" w361 {
              frame "Engineer" {
                n1739 = flat-sequence {
                  tunnel: [w370] -> w363
                  tunnel: [w364] -> w362
                  tunnel: w363 -> [w379]
                  tunnel: w362 -> [w373]
                  frame #0 {
                    n1740 = local read "Post Processing"() -> (w369:T1)
                    n1741 = local read "Proper VI No"() -> (w365:i32)
                    n1742 = call "CRYFlatten Post Processing.vi"("Post-Processing"=w369) -> ("Post Processing flattened"=w364:string)  [unwired: 10 in]
                    n1743 = call "CRYPreUpdate Sequence.vi"("EventName"="SequenceUpdate", "Proper VI No"=w365, "Project View Step Name Identifier Arg1"="", "Step flattened Arg2"=w364, "AllChangeFlg"=TRUE ("Name/Identifier")) -> ()  [unwired: 11 in]
                    n1744 = Build Array(w365) -> (w372:i32[])
                    n1745 = call "CRYGet Curve Library Data Name.vi"("nData"=w372, "sAction"="GetNamebyStep" ("sOption")) -> ("sNames"=w370:string[])  [unwired: 6 in, 3 out]
                  }
                  frame #1 {
                    n1746 = call "CRYGet Current TS Steps.vi"() -> ("SelectStepNumber in Tree"=w374:i32, "Steps"=w375:T5[])  [unwired: 7 in, 3 out]
                    n1747 = Index Array(array=w375, index=w374) -> (element=w376:T5)
                    n1748 = call "CRYPost Processing Curve Name Replace.vi"("Setup in"=w376, "Step Setup in"=w373, "Type In"="StepOK") -> ("Inserted Names Out"=w378:string[])  [unwired: 8 in]
                    n1749 = call "CRYReplace Curve Name of Steps.vi"("New Name"=w378, "Old Name"=w379) -> ()  [unwired: 9 in, 1 out]
                  }
                }
              }
              frame "Technician", Default {
                n1750 = call "CRYGet Error Message.vi"("Kind"="Step Setup") -> ("Window Title"=w382:string)  [unwired: 5 in, 5 out]
                n1751 = call "CRYGet Access Level Message.vi"("sAction"="OK") -> ("Multibyte string"=w384:string)  [unwired: 10 in]
                n1752 = call "CRYMessage Dialog.vi"("Window Title"=w382, "YesNoCancel"=T8."OK", "Message Content"=w384) -> ()  [unwired: 7 in, 2 out]
              }
            }
          }
          frame #1 {
            n1753 = local write "OK"(FALSE ("OK")) -> ()
          }
        }
        n1754 = local write "stop"(TRUE ("stop")) -> ()
      }
      frame 7 {
        n1755 = flat-sequence {
          frame #0 {
            n1756 = local read "Proper VI No"() -> (w387:i32)
            n1757 = call "CRYStepData Manipulate.vi"("sAction"="Restore", "StepNo."=w387) -> ()  [unwired: 10 in]
          }
          frame #1 {
            n1758 = local write "Cancel"(FALSE ("Cancel")) -> ()
          }
        }
        n1759 = local write "stop"(TRUE ("stop")) -> ()
      }
    }
  }
  n1760 = flat-sequence {
    tunnel: w4 -> [w2768]
    frame #0 {
      n1761 = invoke class="VI" method="Ctrl Val.Set"(reference=w2768, "Control Name"="stop", "Value"=TRUE) -> (reference out=w2765:refnum<vi>, error out=w2764:errorcluster)  [unwired: 2 in, 3 out]
      n1762 = case shown="No Error" w2764 {
        tunnel: w2765 -> [w2769 _]
        frame No Error {
          n1763 = while {
            tunnel: w2769 -> [w2774]
            stop <- w2771 stop-if-true
            n1764 = property class="VI"(reference=w2774) -> ("FP.State"=w2773:T10)  [unwired: 1 in, 2 out]
            n1765 = Equal?(x=w2773, y=T10."Closed" ("Front Panel Window:State")) -> (x = y?=w2771:bool)
            n1766 = Wait (ms)(milliseconds to wait=u32 5) -> ()  [unwired: 1 out]
          }
        }
        frame Error {
        }
      }
    }
    frame #1 {
      n1767 = control-ref of="This VI"() -> (w2775:refnum<vi>)
      n1768 = call "CRYWork Before Step Close.vi"("StepVI Ref"=w2775) -> ()  [unwired: 11 in]
    }
    frame #2 {
      w2776 = TRUE ("EndFlag")
      n1769 = local write "StateOut"(w2776) -> ()
      n1770 = local write "EndFlag"(w2776) -> ()
    }
  }
